vi "Process.vi"(8 "error in":errorcluster, 11 "Lockin.UI":refnum<class "Instrument UI.Lockin.lvclass">) -> (0 "error out":errorcluster, 3 "Lockin.UI out":refnum<class "Instrument UI.Lockin.lvclass">)   [LabVIEW 2019, in "Instrument.Lockin.lvlib" / "Instrument UI.Lockin.lvclass"]
doc: "---------------------------------------------------------------\nJKI State Machine Objects™\nhttp://jki.net/state-machine-objects/\nCopyright (C) 2005-2015, JKI <info@jki.net>\nALL RIGHTS RESERVEDJKI State Machine Objects (SMO) 1.0.0.5\nJKI - JKI\nCopyright (c) 2016, JKI"
uses:
  Instrument UI.Lockin.lvclass
  Instrument.DAQ/Typedefs/DAQ.Calibration--Cluster--Array.ctl
  Instrument.DAQ/Typedefs/DAQ.Calibration--Cluster.ctl
  Instrument.Lockin/Typedefs/Results Type--Enum.ctl
  Instrument.DAQ/Typedefs/Channel.Gain--Cluster--Array.ctl
  Instrument.DAQ/Typedefs/Channel.Gain--Cluster.ctl
  Instrument.DAQ/Typedefs/Sweep.Channel--Cluster--Array.ctl
  Instrument.DAQ/Typedefs/Sweep.Channel--Cluster.ctl
  Instrument.DAQ/Typedefs/Sweep.Pattern--Enum.ctl
  Instrument.DAQ/Typedefs/DAQ.Configuration--Cluster--Array.ctl
  Instrument.DAQ/Typedefs/DAQ.Configuration--Cluster.ctl
  Instrument.DAQ/Typedefs/DAQ.Config.AO.Range--enum.ctl
  Instrument.DAQ/Typedefs/DAQ.Config.AI.Range--enum.ctl
  Instrument.DAQ/Typedefs/DAQ.Config.AI.Coupling--enum.ctl
  Instrument.DAQ/Typedefs/DAQ.Sampling.Fs Mode--enum.ctl
  Instrument.DAQ/Typedefs/Simulation Mode--enum.ctl
  Instrument.DAQ/Typedefs/AI.Channel--Cluster--Array.ctl
  Instrument.DAQ/Typedefs/AI.Channel--Cluster.ctl
  Instrument.DAQ/Typedefs/AO.Channel--Cluster--Array.ctl
  Instrument.DAQ/Typedefs/AO.Channel--Cluster.ctl
  Instrument.DAQ/Typedefs/AO.Channel.Function--Enum.ctl
  Instrument.DAQ/Typedefs/REF.Channel--Cluster--Array.ctl
  Instrument.DAQ/Typedefs/REF.Channel--Cluster.ctl
  Typedefs/Display-Enum.ctl
  C:/Program Files/National Instruments/LabVIEW 2019/vi.lib/JKI/JKI SMO/SMO/SMO.lvclass
  C:/Program Files/National Instruments/LabVIEW 2019/user.lib/LevyLab/Instrument Framework/Instrument UI/Instrument UI.lvclass
  C:/Program Files/National Instruments/LabVIEW 2019/vi.lib/JKI/JKI SMO/SMO.UI/SMO.UI.lvclass
  Instrument.DAQ/Typedefs/Get State-enum.ctl
  Instrument.Lockin/Typedefs/API/Lockin.Commands--Enum.ctl
  Instrument.Lockin/Typedefs/API/Lockin.Commands.Local--Enum.ctl
  Instrument.DAQ/Typedefs/Set State-enum.ctl
  Instrument.DAQ/Typedefs/DAQ.Sampling.Sample Mode--Ring.ctl
  Instrument.Lockin/Typedefs/API/Lockin.setSweep_Table--cluster.ctl
  Instrument.Lockin/Typedefs/Offset Mode--Enum.ctl
  Instrument.DAQ/Typedefs/PrivateEvents--DAQ.setCalibration.ctl
  Typedefs/UI.References--Cluster.ctl
  Typedefs/UI.References.Booleans--Cluster.ctl
  Typedefs/UI.References.Clusters--Cluster.ctl
  Typedefs/UI.References.Graphs--Cluster.ctl
  <userlib>/LevyLab/Configuration/Configuration.lvclass
  Instrument.Lockin/Typedefs/Lockin.getAllData--Cluster.ctl
  Instrument.DAQ/Typedefs/PublicEvents--DAQ.getWaveforms.ctl
  Instrument.DAQ/Typedefs/Results--Cluster.ctl
  Instrument.DAQ/Typedefs/PublicEvents--DAQ.getSweepWaveforms.ctl
  Typedefs/UI.Configuration--Cluster.ctl
  Instrument.DAQ/Typedefs/Configuration.Channels--Cluster.ctl
  Instrument.DAQ/Typedefs/DAQ.Sampling--Cluster.ctl
  Instrument.DAQ/Typedefs/DAQ.Sampling.Sampling--Cluster.ctl
  Instrument.DAQ/Typedefs/Configuration.Prefilter--Cluster.ctl
  Instrument.DAQ/Typedefs/Channel.GainsAndOffsets--Cluster.ctl
  Instrument.DAQ/Typedefs/Configuration.AmplitudeLimit--Cluster.ctl
  Instrument.DAQ/Typedefs/Configuration.DCLimit--Cluster.ctl
  Instrument.DAQ/Typedefs/Configuration.LinkFrequencies--Cluster.ctl
  Instrument.DAQ/Typedefs/Sweep.Configuration--Cluster.ctl
  Instrument.Lockin/Instrument.Lockin.lvclass
  C:/Program Files/National Instruments/LabVIEW 2019/user.lib/LevyLab/Instrument Framework/Instrument/Instrument.lvclass
  <userlib>/LevyLab/Instrument Framework/Instrument UI/Instrument UI.lvclass/Instrument UI.ctl
  <userlib>/LevyLab/Configuration/Configuration.lvclass/Configuration.ctl
  <vilib>/JKI/JKI SMO/SMO/SMO.lvclass/SMO.ctl
  <vilib>/JKI/JKI SMO/SMO.UI/SMO.UI.lvclass/SMO.UI.ctl
  Instrument.Lockin/Typedefs/API/Lockin.setState--cluster.ctl
  Instrument.DAQ/Typedefs/PrivateEvents--DAQ.showUI.ctl
  Instrument.Lockin/Typedefs/API/Lockin.setLogMode--cluster.ctl
  Instrument.Lockin/Typedefs/API/Lockin.setSamplingMode--cluster.ctl
  Instrument.Lockin/Typedefs/API/Lockin.setSamplingFsMode--cluster.ctl
  3787d8ba-7746-42f4-a076-e634e239a42a.vi
  <vilib>/JKI/JKI SMO/SMO/Private/ReftoDVR--SMO.vi
  <vilib>/JKI/JKI SMO/SMO.UI/SMO.UI.ReftoDVR.vi
  3787d8ba-7746-42f4-a076-e634e239a42a.vi/a8b20e46-8953-45b0-93f7-28fc699f087e.vi
  3787d8ba-7746-42f4-a076-e634e239a42a.vi/bdb78403-1b99-4c02-9c62-cc137de50f7f.vi
  <vilib>/Platform/browser.llb/Open URL in Default Browser (string).vi
  <vilib>/Waveform/WDTOps.llb/WDT Waveform Duration DBL.vi
  private/Set All Plot Visibility (WFChart).vi
  private/Get Plot Visibility (WFChart).vi
  private/Set Plot Visibility (WFChart).vi
  private/Set Plot Visibility (WDTWFGraph).vi
  private/Set Legend (WDTWFGraph).vi
  private/Set Plot Color (WFChart).vi
  <vilib>/Utility/Data Type/Get Type Information.vi
  <vilib>/Utility/Data Type/Get Numeric Information.vi
  <userlib>/_OpenG.lib/lvdata/lvdata.llb/Unwrap VVariant__ogtk.vi
  <vilib>/JDP Science/JSONtext/Variant to JSON Text.vi
  <userlib>/LevyLab/Instrument Framework/Instrument/API/Instrument.sendMessageToProcess (string).vi
  <userlib>/LevyLab/Instrument Framework/Instrument/Instrument.lvclass
  <vilib>/JDP Science/JSONtext/LVClass Serializer/JSONtext LVClass Serializer.lvclass
  <userlib>/LevyLab/Instrument Framework/Instrument UI/Instrument UI.lvclass
  Instrument.DAQ/Instrument.DAQ.lvclass
  <vilib>/measure/NI_MAPro.lvlib
  <vilib>/JKI/JKI SMO/SMO/SMO.lvclass
  <vilib>/JKI/JKI SMO/SMO.UI/SMO.UI.lvclass
  Lockin.Utilities/Lockin.Utilities.lvlib
  private/Set All Plot Visibility (WFGraph).vi
  private/Set All Plot Visibility (XYGraph).vi
  private/Get Plot Visibility (WFGraph).vi
  private/Set Plot Visibility (WFGraph).vi
  private/Set Plot Visibility (XYGraph).vi
  private/Set Legend (WFGraph).vi
  private/Set Plot Color (WFGraph).vi
  private/Set Plot Color (WDTWFGraph).vi
  private/Set Legend (WFChart).vi
  private/Set Legend (XYGraph).vi
  private/Set Plot Color (XYGraph).vi
  <vilib>/measure/maspectr.llb/FFT Power Spectrum and PSD for N Chan.vi
panel:
  in  "Decimation (post DSP)":i32=1
  in  "....................State....................":bool
  in  "....................Graph and UI....................":bool
  in  "....................DAQ and Channel....................":bool
  in  "....................Dynamic Events....................":bool
  out "Version":string="vDevelopment" caption="V"
  in  "Left Tab":T1(tab)=enum."Sweep"
  in  "AO DC Limit":dbl=0.009999999 format="%.3p"
  in  "Limit DC (V)":bool
  in  "Disable all AI Ref":bool
  in  "Enable only AI Ref1":bool
  in  "Reset Phase":bool
  in  "AI Channels":T2 {"References" items=["", "1", "2", "3"]; "Channel" min=1}
  in  "AO freq link":dbl=13.0 format="%.3p"
  in  "AO Amp Limit":dbl=0.009999999 format="%.3p"
  in  "Limit Amplitude (V)":bool
  in  "Link Frequencies":bool
  in  "LP f (Hz)":dbl=100.0 format="%.3p"
  in  "Line":bool
  in  "Lowpass":bool
  in  "AO Channels":T4 {"Phase" format="%.3g"; "Frequency" min=0.0001 max=10000.0 format="%.3g"; "Offset" format="%.3p"; "Amplitude" min=0.0 max=10.0 format="%.3p"}
  in  "REF Channels":T7 {"Roll-Off" min=1; "TC" min=0.0001 format="%#_3p"; "Phase" format="%.3g"; "Frequency" min=0.0001 max=10000.0 format="%.3g"; "Channel" min=1}
  in  "Input Gain":T9
  in  "Output Gain":T9
  in  "Input Offsets":T9 {"Gain" format="%#_3p"}
  in  "Show UI":bool
  in  "Fs Output (S/s)":dbl=10.0 format="%#_13g"
  in  "Fs (S/s)":dbl=10.0 format="%#_13g"
  in  "#s (S)":i32=10
  in  "DAQ Config":T11 {"AI.Coupling" items=["AC"=10045, "DC"=10050, "GND"=10066]}
  in  "Auto DAQ":bool caption="Auto"
  in  "Refresh Rate (Hz)":dbl=10.0 format="%#_13g"
  in  "Fs Mode":T16
  in  "Fs Multiplier":dbl=5000.0 format="%#_13g"
  in  "Decimation (pre DSP)":i32=1
  in  "Remove Offset":bool caption="Remove"
  in  "Measure Offset":bool caption="Measure"
  in  "Logging":bool
  in  "AI Simulation mode":T17=enum."AI = noise*AO"
  in  "Sweep Pattern":cluster{"Channel":u16, "Sweep Pattern":dbl[]}[](array[cluster])=[{"Channel"=0, "Sweep Pattern"=[]}] {"Sweep Pattern" format="%#_3p"; "Channel" min=1 max=128}
  in  "Sweep Channels":T18=[{"Enable?"=FALSE, "Channel"=0, "Start"=0.0, "End"=0.1, "Pattern"=enum."Table", "Table"=[]}] {"Table" format="%#_1f"; "Channel" min=1 max=128; "Start" format="%#_6p"; "End" format="%#_6p"}
  in  "Sweep Time (s)":dbl=20.0
  in  "Initial Wait (s)":dbl=1.0
  out "Sweep Timer (s)":dbl caption="Timer (s)"
  in  "Return to Start?":bool
  out "Sampling Status":string="Good"
  out "State History":string
  out "WFM Refresh time (ms)":u32=103
  out "Instrument.DAQ SMO State":string caption="SMO State"
  out "UI Refresh time (ms)":u32=103
  in  "Update":bool
  in  "Enable Output":bool caption="Enable"
  in  "Output Channel":i32=1 min=1
  out "Output (V)":dbl
  in  "Aux Channel":tag="Dev2/ao0"
  in  "Voltage Output (V)":dbl min=-50.0 max=50.0
  in  "Amplifier Gain":dbl=1.0 min=-15.0 max=15.0
  out "DAQ Output (V)":dbl=-0.0 min=-3.5 max=3.5
  out "Amplified Output (V)":dbl=-0.0 min=-3.5 max=3.5
  in  "AI Channel":i32=1
  in  "Reference Channel":i32=1
  in  "Type":T21
  out "state":T22=enum."created"
  out "current time":dbl format="%<%I:%M:%S %p %m/%d/%Y>T"
  out "getAll.DAQ state":T22=enum."created"
  out "current time 2":dbl format="%<%I:%M:%S %p %m/%d/%Y>T"
  in  "Get Calibration":bool
  out "Cal Info":T23 {"DevTemp" format="%.1f"; "SelfCal.LastTemp" format="%.1f"; "SelfCal.LastDate/Time" format="%<%I:%M %p %m/%d/%Y>T"}
  in  "Self Calibrate":bool
  in  "Tab Control 3":enum32{"Page 1"}(tab)
  out "X":dbl caption="X (V)" format="%#_3p"
  out "Y":dbl caption="Y (V)" format="%#_3p"
  in  "Channel":i32(ring)=1 items=["AI1 Ref1", "AI2 Ref1", "AI3 Ref1", "AI4 Ref1", "AI5 Ref1", "AI6 Ref1", "AI7 Ref1", "AI8 Ref1"]
  out "R":dbl caption="R (V)" format="%#_3p"
  out "Theta":dbl caption="Theta (°)" format="%#_3p"
  in  "Display":T25=enum."R and Theta" caption="Enum"
  in  "Close":bool
  out "Status":string="Shutdown"
  in  "Pause":bool
  in  "Reset":bool
  in  "Start":bool
  in  "Help":bool
  in  "Start Sweep":bool
  in  "Stop Sweep":bool
  in  "Right Tab":T26(tab)
  in  "AI Graph All":bool
  in  "AI Graph None":bool
  in  "Y Axis (Output)":enum16{"Analog Output", "Reference"}(ring) caption="Enum 3"
  in  "Y Axis (Input)":enum16{"Device", "ADC"}(ring) caption="Enum 3"
  in  "Decimate (UI)":enum16{"1", "10", "100", "1000"}(ring) caption="Enum 3"
  in  "X Axis":enum16{"Time", "Samples"}(ring) caption="Enum 3"
  out "AI Graph":waveform(dbl)[](graph)
  out "AO Graph":waveform(dbl)[](graph)
  in  "AO Graph All":bool
  in  "AO Graph None":bool
  in  "Y/Theta Range":dbl caption="Axis Range" format="%#_6p"
  in  "X/R Range":dbl caption="Axis Range" format="%#_6p"
  out "Lockin 2":waveform(dbl)[](graph) caption="Lockin Display 2"
  out "Lockin 1":waveform(dbl)[](graph)
  in  "Lockin Graph None":bool
  in  "Lockin Graph All":bool
  out "Results":string[][](table)
  out "XY Graph":cluster{"Wavenumber":dbl[], "Data":dbl[]}[](graph)
  in  "XY Range":dbl caption="Axis Range" format="%#_6p"
  out "Sweep AI":waveform(dbl)[](graph)
  out "Sweep AO":waveform(dbl)[](graph)
  out "Sweep Results Y":waveform(dbl)[](graph)
  out "Sweep Results X":waveform(dbl)[](graph)
  in  "# averages":u32=10 min=1
  in  "weighting mode":enum16{"Linear", "Exponential"}(ring)=enum."Exponential"
  in  "averaging mode":T27(ring)=enum."RMS averaging"
  in  "window":u16(ring) items=["Rectangle", "Hanning"]
  in  "export mode":u16(ring)=1 items=["Power Spectrum", "Power Spectral Density"]
  in  "restart":bool
  out "done?":bool=TRUE
  out "PS Chart":dbl[][](graph)
  out "PS WFGraph":cluster{"f0":dbl, "df":dbl, "magnitude":dbl[]}[](graph)
  out "averages":dbl=180.0
  # "Lockin UI"
  # "For instructions on how to use the JKI State Machine Objects, examples and video tutorials, visit:\nhttp://jki.net/state-machine-objects/\n\nJKI State Machine Objects™\nhttp://jki.net/state-machine-objects/\nCopyright (C) 2005-2015, JKI <info@jki.net>\nALL RIGHTS RESERVED"
  # "Output"
  # "Input"
  # ">> DEVICE >>"
  # "(*)"
  # "Ch"
  # "Amp (V)"
  # "DC (V)"
  # "f (Hz)"
  # "Phase (°)"
  # "Function"
  # "Sweep"
  # "(*)"
  # "Ch"
  # "Ref1   2     3    4"
  # "Input: Pre-Filter"
  # "Output Settings"
  # "Reference"
  # "Reference Settings"
  # "Ch"
  # "f (Hz)"
  # "Phase (°)"
  # "TC (s)"
  # "Order (n/2)"
  # "Ch"
  # "Input Gain"
  # "Ch"
  # "Output Gain"
  # "Ch"
  # "Offset"
  # "DAQ Channels"
  # "AI"
  # "Device"
  # "AO"
  # "DAQ"
  # "Ch"
  # "Range"
  # "Ch"
  # "Range"
  # "Coupling"
  # "Logging"
  # "Sampling"
  # "Input: Offset"
  # "Sweep"
  # "Pattern"
  # "(*)"
  # "Ch"
  # "Start"
  # "End"
  # "Ch"
  # "Table"
  # "Status"
  # "Auxiliary Output"
  # "Configuration"
  # "- Use to control an auxiliiary card such as a multifunction DAQ (6115, 6120, etc)"
  # "Forward Lockin Input --> Lockin Output"
  # "- Choose an input lockin channel and value (X,Y, etc) and it will be written as a DC value to an output channel of your choosing.\n- Output is scaled by the input amplifier gain."
  # "Calibration"
  # "Self Cal\nLast Time"
  # "Self Cal\nLast Temp"
  # "Temp\nNow"
  # "Cal\nDue"
  # "Device"
  # "DAQ"
  # "Sweep"
  # "Application"
  # "Status"
  # "AI Graph"
  # "AO/Reference Graph"
  # "Lockin Results 1"
  # "Lockin Results 2"
  # "Lockin Results 3"
  # "Sweep AO/AI"
  # "Sweep Results"
  # "Power Spectra"
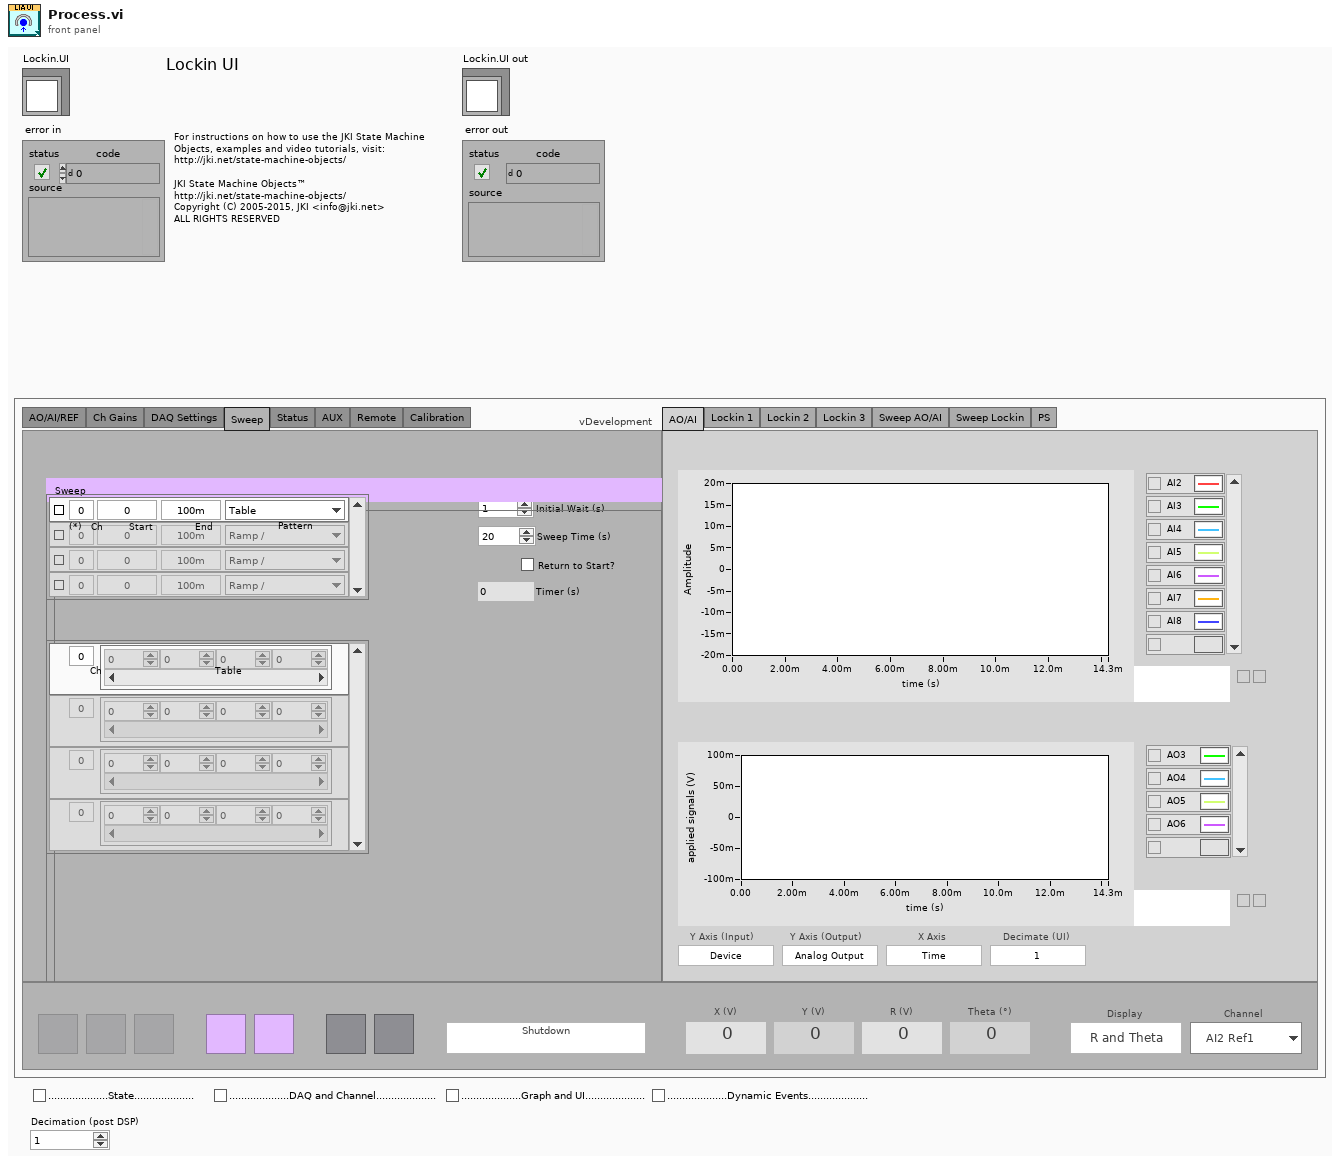
[diagram p1: front panel]
types:
  T1 = enum32{"AO/AI/REF", "Ch Gains", "DAQ Settings", "Sweep", "Status", "AUX", "Remote", "Calibration"}
  T2 = typedef "Instrument.Lockin.lvlib/Instrument.DAQ.lvclass/AI.Channel--Cluster--Array.ctl" = T3[]
  T3 = typedef "Instrument.Lockin.lvlib/Instrument.DAQ.lvclass/AI.Channel--Cluster.ctl" = cluster{"Enable?":bool, "Channel":i32, "References":i32[]}
  T4 = typedef "Instrument.Lockin.lvlib/Instrument.DAQ.lvclass/AO.Channel--Cluster--Array.ctl" = T5[]
  T5 = typedef "Instrument.Lockin.lvlib/Instrument.DAQ.lvclass/AO.Channel--Cluster.ctl" = cluster{"Enable?":bool, "Channel":i32, "Amplitude":dbl, "Offset":dbl, "Frequency":dbl, "Phase":dbl, "Function":T6, "Sweeping?":bool}
  T6 = typedef "Instrument.Lockin.lvlib/Instrument.DAQ.lvclass/AO.Channel.Function--Enum.ctl" = enum16{"Sine", "Triangle", "Square"}
  T7 = typedef "Instrument.Lockin.lvlib/Instrument.DAQ.lvclass/REF.Channel--Cluster--Array.ctl" = T8[]
  T8 = typedef "Instrument.Lockin.lvlib/Instrument.DAQ.lvclass/REF.Channel--Cluster.ctl" = cluster{"Enable?":bool, "Channel":i32, "Frequency":dbl, "Phase":dbl, "TC":dbl, "Roll-Off":i32}
  T9 = typedef "Instrument.Lockin.lvlib/Instrument.DAQ.lvclass/Channel.Gain--Cluster--Array.ctl" = T10[]
  T10 = typedef "Instrument.Lockin.lvlib/Instrument.DAQ.lvclass/Channel.Gain--Cluster.ctl" = cluster{"Channel":string, "Gain":dbl}
  T11 = typedef "Instrument.Lockin.lvlib/Instrument.DAQ.lvclass/DAQ.Configuration--Cluster--Array.ctl" = T12[]
  T12 = typedef "Instrument.Lockin.lvlib/Instrument.DAQ.lvclass/DAQ.Configuration--Cluster.ctl" = cluster{"Device":string, "AO.Ch":string, "AO.Range":T13, "AI.Ch":string, "AI.Range":T14, "AI.Coupling":T15}
  T13 = typedef "Instrument.Lockin.lvlib/Instrument.DAQ.lvclass/DAQ.Config.AO.Range--enum.ctl" = enum16{"±0.1", "±1.0", "±10.0"}
  T14 = typedef "Instrument.Lockin.lvlib/Instrument.DAQ.lvclass/DAQ.Config.AI.Range--enum.ctl" = enum16{"±0.316", "±1.00", "±3.16", "±10.0", "±31.6", "±42.4"}
  T15 = typedef "Instrument.Lockin.lvlib/Instrument.DAQ.lvclass/DAQ.Config.AI.Coupling--enum.ctl" = u16
  T16 = typedef "Instrument.Lockin.lvlib/Instrument.DAQ.lvclass/DAQ.Sampling.Fs Mode--enum.ctl" = enum16{"Manual", "Auto Fs", "Max Fs"}
  T17 = typedef "Instrument.Lockin.lvlib/Instrument.DAQ.lvclass/Simulation Mode--enum.ctl" = enum16{"AI = HW simulated", "AI = noise*AO", "AI = waveguide"}
  T18 = typedef "Instrument.Lockin.lvlib/Instrument.DAQ.lvclass/Sweep.Channel--Cluster--Array.ctl" = T19[]
  T19 = typedef "Instrument.Lockin.lvlib/Instrument.DAQ.lvclass/Sweep.Channel--Cluster.ctl" = cluster{"Enable?":bool, "Channel":u16, "Start":dbl, "End":dbl, "Pattern":T20, "Table":dbl[]}
  T20 = typedef "Instrument.Lockin.lvlib/Instrument.DAQ.lvclass/Sweep.Pattern--Enum.ctl" = enum16{"Ramp /", "Ramp /\\", "Smooth Ramp _/", "Smooth Ramp _/\\_", "Table"}
  T21 = typedef "Instrument.Lockin.lvlib/Instrument.Lockin.lvclass/Results Type--Enum.ctl" = enum16{"X", "Y", "R", "Theta", "Mean"}
  T22 = typedef "Instrument.Lockin.lvlib/Instrument.DAQ.lvclass/Get State-enum.ctl" = enum16{"idle", "created", "started", "stopped", "sweeping"}
  T23 = typedef "Instrument.Lockin.lvlib/Instrument.DAQ.lvclass/DAQ.Calibration--Cluster--Array.ctl" = T24[]
  T24 = typedef "Instrument.Lockin.lvlib/Instrument.DAQ.lvclass/DAQ.Calibration--Cluster.ctl" = cluster{"Active Device":string, "SelfCal.LastDate/Time":dbl, "SelfCal.LastTemp":dbl, "DevTemp":dbl, "calibration due?":bool}
  T25 = typedef "Instrument.Lockin.lvlib/Instrument UI.Lockin.lvclass/Display-Enum.ctl" = enum16{"X and Y", "R and Theta", "Mean"}
  T26 = enum32{"AO/AI", "Lockin 1", "Lockin 2", "Lockin 3", "Sweep AO/AI", "Sweep Lockin", "PS"}
  T27 = enum16{"No averaging", "Vector averaging", "RMS averaging", "Peak hold"}
  T28 = typedef "Instrument.Lockin.lvlib/Instrument.Lockin.lvclass/Lockin.Commands.Local--Enum.ctl" = enum16{"autoConfigureDAQ", "setSimulationMode", "zeroPhase", "setCalibration", "setPreFilter", "setLinkFrequencies", "setLimitAmplitude", "setLimitDC", "setSamplingDecimationPreDSP", "setSamplingDecimationPostDSP", "setSamplingMode", "setSamplingFsMultiplier", "setSamplingFsOutput", "setSamplingRefreshRate", "setData_State", "setData_DAQ", "setData_Sampling", "setData_Waveforms", "setData_Results", "setData_SweepWaveforms", "setData_AIChannels", "setData_AOChannels", "setData_REFChannels", "setData_InputGain", "setData_OutputGain", "showUI", "setAI", "setOffset", "setOffsetMode"}
  T29 = typedef "Instrument.Lockin.lvlib/Instrument.Lockin.lvclass/Lockin.Commands--Enum.ctl" = enum16{"setAO", "setAO_Amplitude", "setAO_DC", "setAO_Frequency", "setAO_Phase", "setAO_Function", "setREF", "setREF_Frequency", "setREF_Phase", "setREF_TC", "setREF_Roll-Off", "setDAQ", "setSampling", "setState", "getState", "getAO", "getAI", "getResults", "getSampling", "getAOconfig", "getREFconfig", "setInputGain", "setOutputGain", "getInputGain", "getOutputGain", "setSamplingFsMode", "getSamplingFsMode", "setSweep", "setSweep_Time", "setSweep_Table", "getStatus", "getSweepResults", "getSweepWaveforms", "startLogging", "stopLogging"}
  T30 = enum16{"Spinner 1", "Spinner 2", "Spinner 3", "Spinner 4", "Spinner 5", "Spinner 6"}
  T31 = typedef "Instrument.Lockin.lvlib/Instrument.DAQ.lvclass/Set State-enum.ctl" = enum16{"start", "stop", "reset", "start sweep", "stop sweep"}
  T32 = typedef "Instrument.Lockin.lvlib/Instrument.Lockin.lvclass/Lockin.setSweep_Table--cluster.ctl" = cluster{"Channel":i32, "Table":dbl[]}
  T33 = typedef "Instrument.Lockin.lvlib/Instrument.Lockin.lvclass/Offset Mode--Enum.ctl" = enum16{"Measure", "Remove"}
  T34 = typedef "Instrument.Lockin.lvlib/Instrument.DAQ.lvclass/PrivateEvents--DAQ.setCalibration.ctl" = enum16{"Check", "Calibrate"}
  T35 = enum32{"invalid app kind", "Development System", "Run Time System", "Student Edition", "Embedded LabVIEW", "Evaluation", "Custom"}
  T36 = enum8{"Enabled", "Disabled", "Disabled and Grayed Out"}
  T37 = enum32{"Invalid", "Standard", "Closed", "Hidden", "Minimized", "Maximized"}
  T38 = typedef "Instrument.Lockin.lvlib/Instrument.Lockin.lvclass/Lockin.setState--cluster.ctl" = cluster{"State":T31}
  T39 = typedef "Instrument.Lockin.lvlib/Instrument.DAQ.lvclass/PrivateEvents--DAQ.showUI.ctl" = bool
  T40 = typedef "Instrument.Lockin.lvlib/Instrument.Lockin.lvclass/Lockin.setLogMode--cluster.ctl" = cluster{"interval":u32}
  T41 = typedef "Instrument.Lockin.lvlib/Instrument.Lockin.lvclass/Lockin.setSamplingMode--cluster.ctl" = cluster{"SampleMode":T42}
  T42 = typedef "Instrument.Lockin.lvlib/Instrument.DAQ.lvclass/DAQ.Sampling.Sample Mode--Ring.ctl" = i32
  T43 = typedef "Instrument.Lockin.lvlib/Instrument.Lockin.lvclass/Lockin.setSamplingFsMode--cluster.ctl" = cluster{"FsMode":T16}
  T44 = cluster{"averaging mode":enum16{"No averaging", "Vector averaging", "RMS averaging", "Peak hold"}, "weighting mode":enum16{"Linear", "Exponential"}, "number of averages":u32}
  T45 = typedef "Instrument.Lockin.lvlib/Instrument UI.Lockin.lvclass/UI.Configuration--Cluster.ctl" = cluster{"Channels":T46, "DAQ":cluster{"Configuration":T11, "cfg.Sampling":T47, "Calibration":T23, "Simulation mode":T17}, "PreFilter":T49, "Amplifers":T50, "Limit Amplitude":T51, "Limit DC":T52, "Link Frequencies":T53, "Aux Channel":tag, "Sweep":T54, "Plot":cluster{"visibility.AI":bool[], "visibility.AO":bool[], "visibility.Lockin":bool[]}}
  T46 = typedef "Instrument.Lockin.lvlib/Instrument.DAQ.lvclass/Configuration.Channels--Cluster.ctl" = cluster{"Cfg_AO":T4, "Cfg_AI":T2, "Cfg_REF":T7}
  T47 = typedef "Instrument.Lockin.lvlib/Instrument.DAQ.lvclass/DAQ.Sampling--Cluster.ctl" = cluster{"Sampling":T48, "sample mode":i32, "Fs Mode":T16, "Fs Multiplier":dbl, "Refresh Rate (Hz)":dbl, "Decimation.PreDSP":i32, "Decimation.PostDSP":i32, "Fs.Output":dbl}
  T48 = typedef "Instrument.Lockin.lvlib/Instrument.DAQ.lvclass/DAQ.Sampling.Sampling--Cluster.ctl" = cluster{"Fs":dbl, "#s":i32}
  T49 = typedef "Instrument.Lockin.lvlib/Instrument.DAQ.lvclass/Configuration.Prefilter--Cluster.ctl" = cluster{"60 Hz":bool, "Low Pass":bool, "Low Pass Cutoff (Hz)":dbl}
  T50 = typedef "Instrument.Lockin.lvlib/Instrument.DAQ.lvclass/Channel.GainsAndOffsets--Cluster.ctl" = cluster{"Offset_AI":T9, "Gain_AI":T9, "Gain_AO":T9}
  T51 = typedef "Instrument.Lockin.lvlib/Instrument.DAQ.lvclass/Configuration.AmplitudeLimit--Cluster.ctl" = cluster{"Limit?":bool, "Limit (V)":dbl}
  T52 = typedef "Instrument.Lockin.lvlib/Instrument.DAQ.lvclass/Configuration.DCLimit--Cluster.ctl" = cluster{"Limit?":bool, "Limit (V)":dbl}
  T53 = typedef "Instrument.Lockin.lvlib/Instrument.DAQ.lvclass/Configuration.LinkFrequencies--Cluster.ctl" = cluster{"Link?":bool, "Frequency (Hz)":dbl}
  T54 = typedef "Instrument.Lockin.lvlib/Instrument.DAQ.lvclass/Sweep.Configuration--Cluster.ctl" = cluster{"Sweep Time (s)":dbl, "Initial Wait (s)":dbl, "Return to Start":bool, "Channels":T18}
  T55 = typedef "Instrument.Lockin.lvlib/Instrument.Lockin.lvclass/Lockin.getAllData--Cluster.ctl" = cluster{"DAQ State":T22, "Waveforms":T56, "Results":T57, "SweepWaveforms":T58}
  T56 = typedef "Instrument.Lockin.lvlib/Instrument.DAQ.lvclass/PublicEvents--DAQ.getWaveforms.ctl" = cluster{"AO_wfm":waveform(dbl)[], "AI_wfm":waveform(dbl)[], "Ref_X_wfm":waveform(dbl)[], "Ref_Y_wfm":waveform(dbl)[], "X_wfm":waveform(dbl)[], "Y_wfm":waveform(dbl)[]}
  T57 = typedef "Instrument.Lockin.lvlib/Instrument.DAQ.lvclass/Results--Cluster.ctl" = cluster{"Time Stamp":timestamp, "Results (Dictionary)":cluster{"key":string, "value":dbl}[]}
  T58 = typedef "Instrument.Lockin.lvlib/Instrument.DAQ.lvclass/PublicEvents--DAQ.getSweepWaveforms.ctl" = cluster{"AO_wfm":waveform(dbl)[], "AI_wfm":waveform(dbl)[], "X_wfm":waveform(dbl)[], "Y_wfm":waveform(dbl)[]}
  T59 = typedef "Instrument.Lockin.lvlib/Instrument UI.Lockin.lvclass/UI.References--Cluster.ctl" = cluster{"Booleans":T60, "Clusters":T61, "Graphs":T62}
  T60 = typedef "Instrument.Lockin.lvlib/Instrument UI.Lockin.lvclass/UI.References.Booleans--Cluster.ctl" = cluster{"Start":refnum<vi>, "Pause":refnum<vi>, "Reset":refnum<vi>, "Trigger":refnum<vi>, "Help":refnum<vi>, "Close":refnum<vi>, "Start Sweep":refnum<vi>, "Stop Sweep":refnum<vi>}
  T61 = typedef "Instrument.Lockin.lvlib/Instrument UI.Lockin.lvclass/UI.References.Clusters--Cluster.ctl" = cluster{"AO Channels":refnum<vi>, "AI Channels":refnum<vi>, "REF Channels":refnum<vi>, "DAQ Config":refnum<vi>, "Sweep Channels":refnum<vi>, "Cal Info":refnum<vi>}
  T62 = typedef "Instrument.Lockin.lvlib/Instrument UI.Lockin.lvclass/UI.References.Graphs--Cluster.ctl" = cluster{"AI Graph":refnum<vi>, "AO Graph":refnum<vi>, "Lockin 1":refnum<vi>, "Lockin 2":refnum<vi>, "XY Graph":refnum<vi>, "Sweep X Graph":refnum<vi>, "Sweep Y Graph":refnum<vi>, "Sweep AI Graph":refnum<vi>, "Sweep AO Graph":refnum<vi>, "PS WFGraph":refnum<vi>, "PS Chart":refnum<vi>}
  T63 = cluster{"Core":cluster{"Current VI Reference":refnum<vi>, "Close Panel on Exit?":bool, "Last Error":cluster{"error":errorcluster, "previous state":string, "remaining states":string}, "Shutdown?":bool}, "SelfRef":refnum<class "Instrument UI.Lockin.lvclass">, "Lockin":refnum<class "Instrument.Lockin.lvclass">, "Configuration":refnum<class "Configuration.lvclass">, "UI Config":T45, "DAQ state":T22, "getAll":T55, "References":T59, "Message":cluster{"Command":variant, "Data":variant}, "Plot Names":string[], "Front Panel":refnum<vi>}
  T64 = typedef "SMO.lvclass/SMOState --Enum.ctl" = enum16{"unknown", "Created", "Started", "Stopped"}
  T65 = cluster{"Current VI Reference":refnum<vi>, "Close Panel on Exit?":bool, "Last Error":cluster{"error":errorcluster, "previous state":string, "remaining states":string}, "Shutdown?":bool}
  T66 = typedef "SMO.lvclass/Protected Events.ctl" = cluster{"StopProcesses":refnum<user-event>, "AbortProcesses":refnum<user-event>, "Config Changed":refnum<user-event>, "Dependency":refnum<user-event>}
  T67 = typedef "Instrument.lvlib/Instrument.lvclass/PublicEvents--Cluster.ctl" = cluster{"MessageFromProcess":refnum<user-event>}
  T68 = typedef "SMO.UI.lvclass/PublicEvents--Cluster.ctl" = cluster{"UI Hidden":refnum<user-event>, "UI State":refnum<user-event>}
  T69 = typedef "SMO.lvclass/Public Events.ctl" = cluster{"Error":refnum<user-event>, "State":refnum<user-event>, "Reserve State":refnum<user-event>}
  T70 = typedef "Instrument.Lockin.lvlib/Instrument.DAQ.lvclass/PublicEvents--Cluster.ctl" = cluster{"getAIChannels":refnum<user-event>, "getAOChannels":refnum<user-event>, "getREFChannels":refnum<user-event>, "getWaveforms":refnum<user-event>, "getResults":refnum<user-event>, "getSweepWaveforms":refnum<user-event>, "getCalibration":refnum<user-event>, "getDAQState":refnum<user-event>, "getDAQconfig":refnum<user-event>, "getInputGain":refnum<user-event>, "getOutputGain":refnum<user-event>, "getInputOffset":refnum<user-event>, "getSampling":refnum<user-event>, "getSweepChannels":refnum<user-event>, "getDeviceIDN":refnum<user-event>}
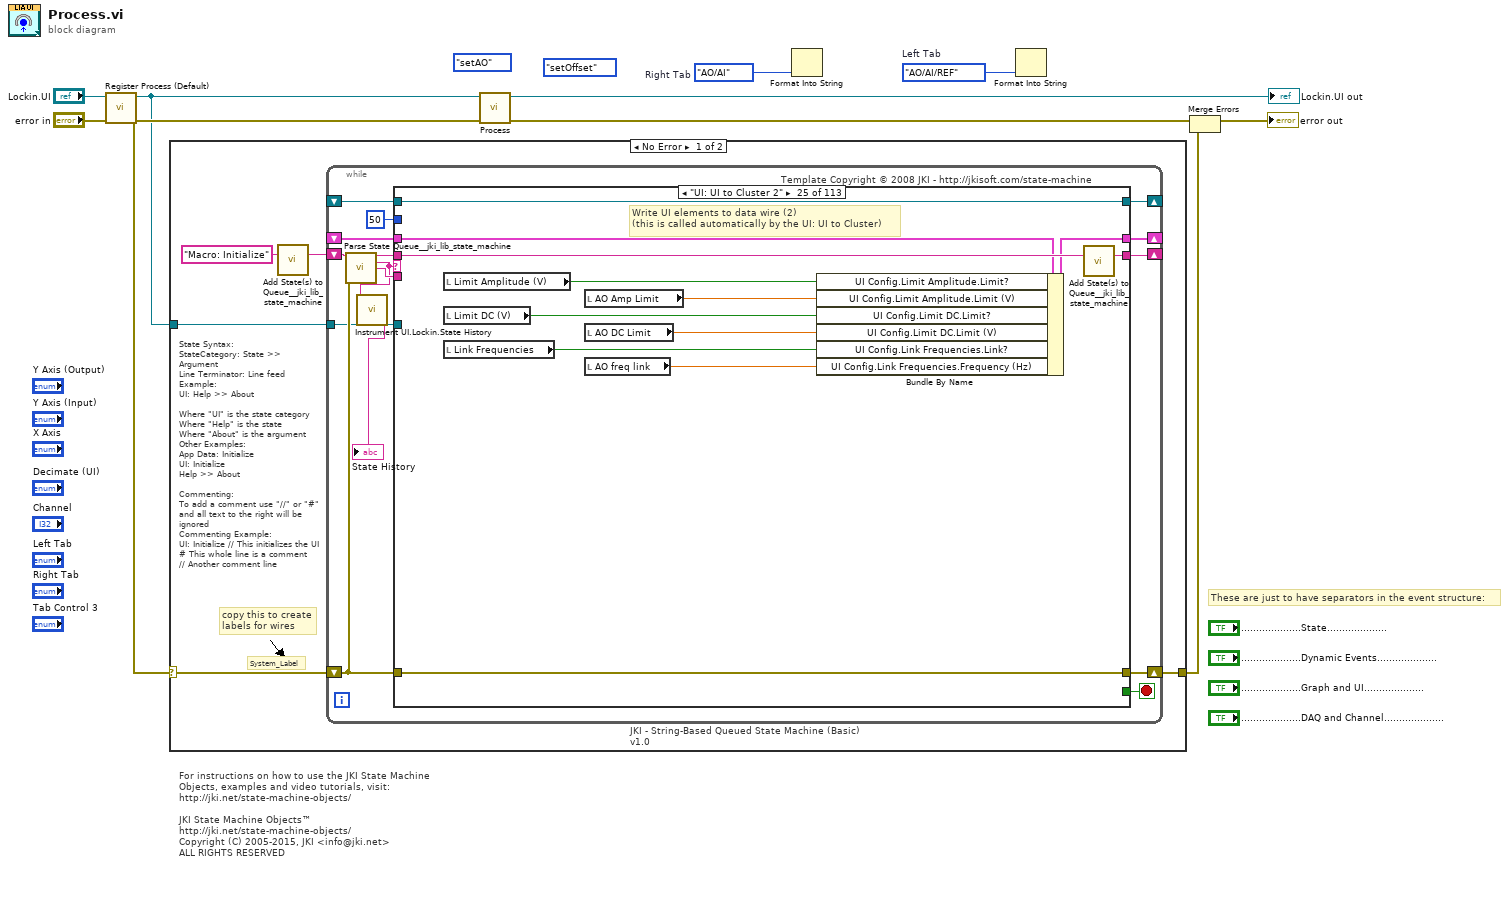
[diagram p0: block diagram]
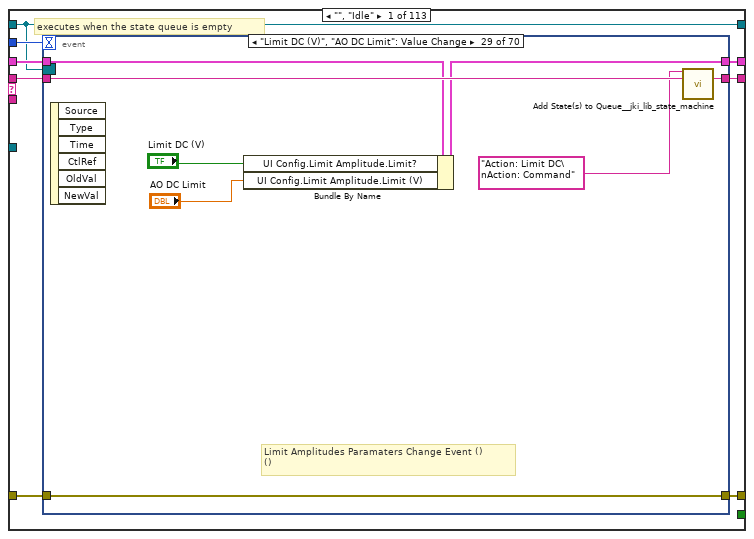
[diagram p2: hidden frame]
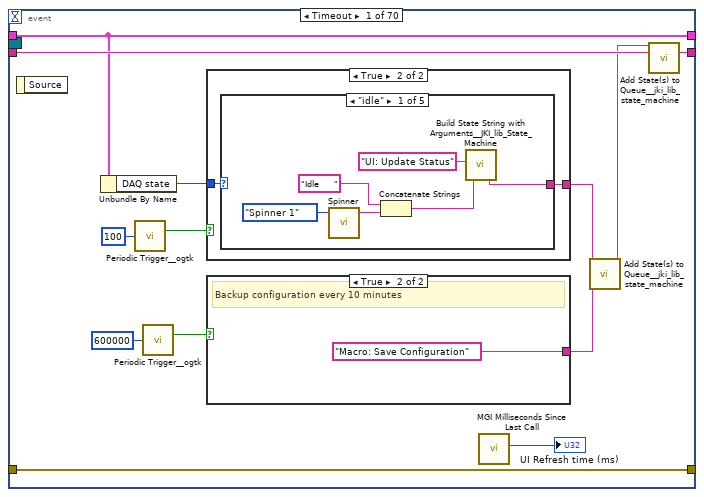
[diagram p3: hidden frame]
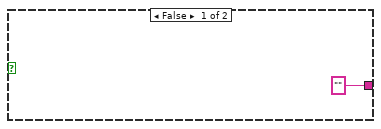
[diagram p4: hidden frame]
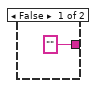
[diagram p5: hidden frame]
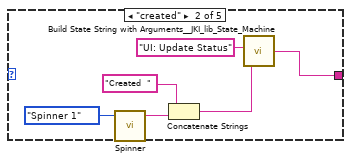
[diagram p6: hidden frame]
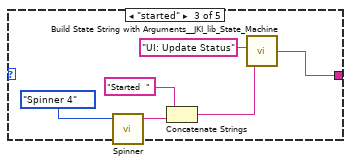
[diagram p7: hidden frame]
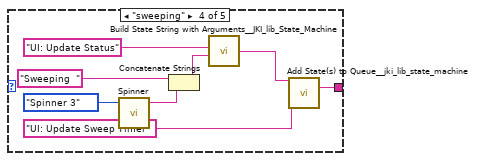
[diagram p8: hidden frame]
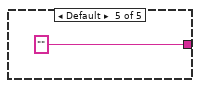
[diagram p9: hidden frame]
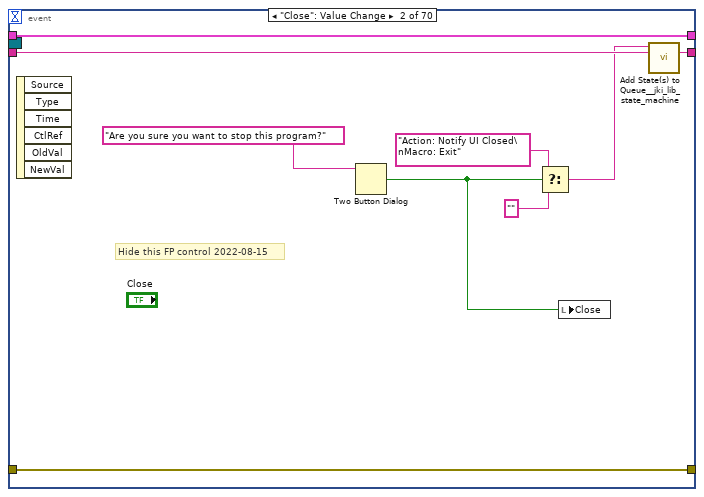
[diagram p10: hidden frame]
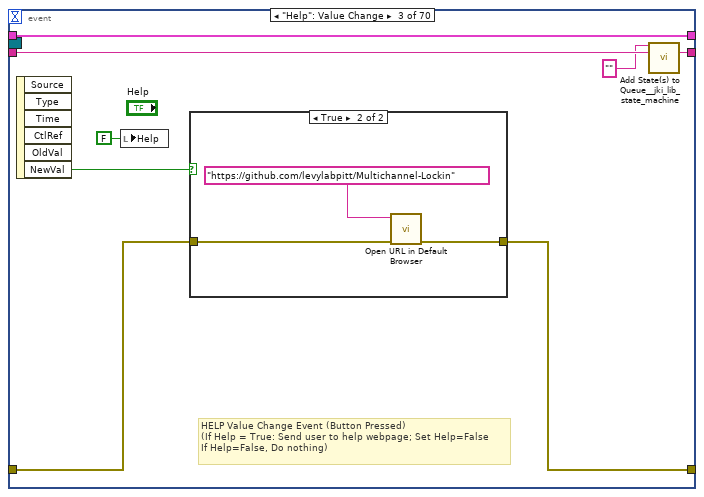
[diagram p11: hidden frame]
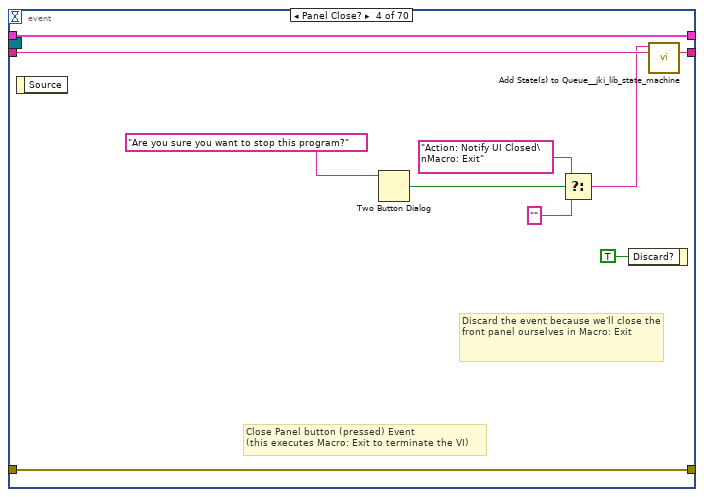
[diagram p13: hidden frame]
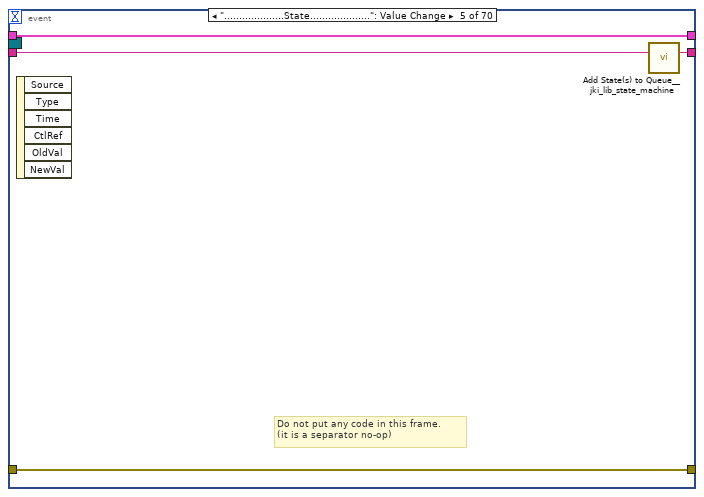
[diagram p14: hidden frame]
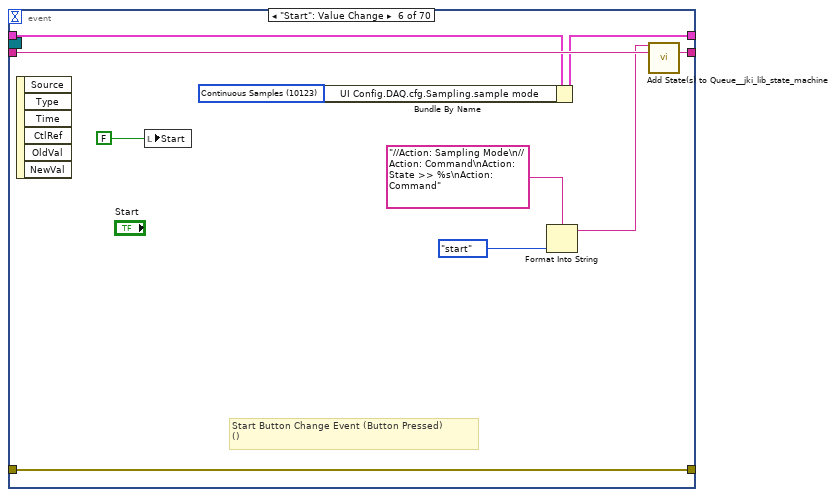
[diagram p15: hidden frame]
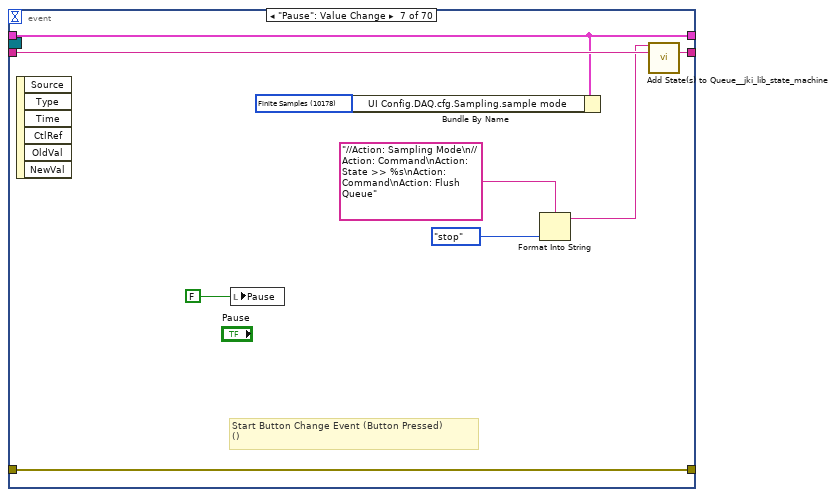
[diagram p16: hidden frame]
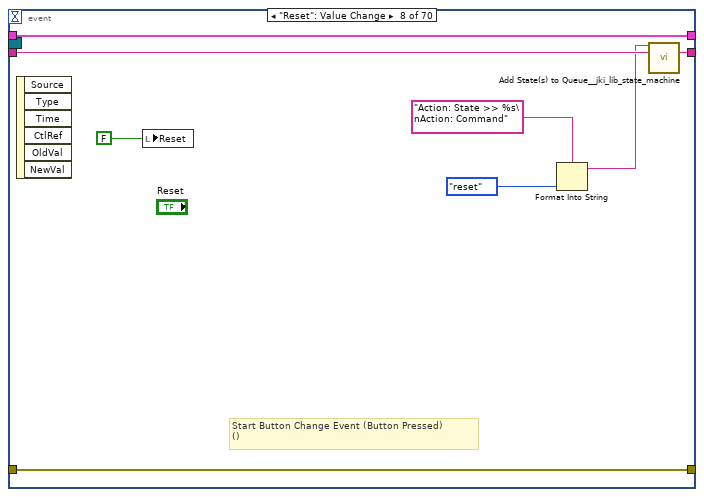
[diagram p17: hidden frame]
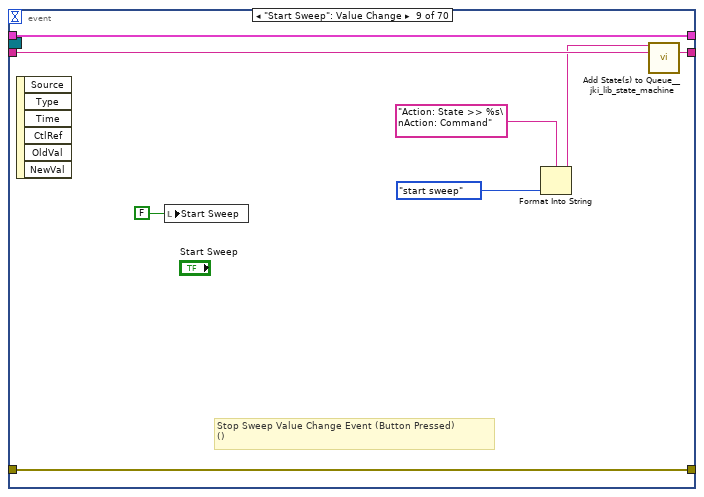
[diagram p18: hidden frame]
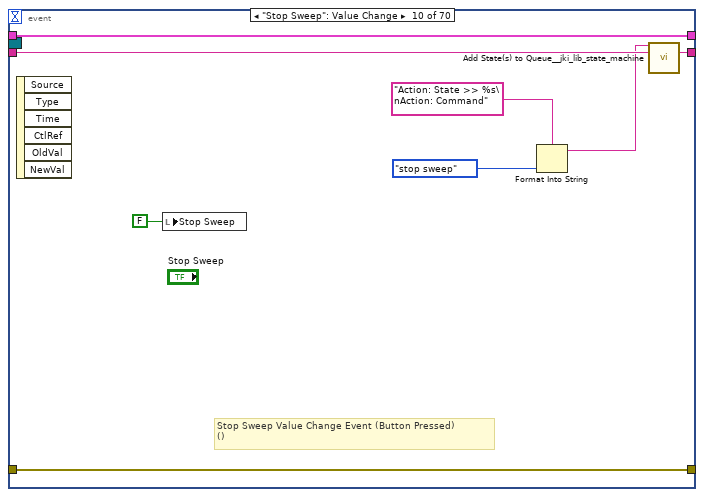
[diagram p19: hidden frame]
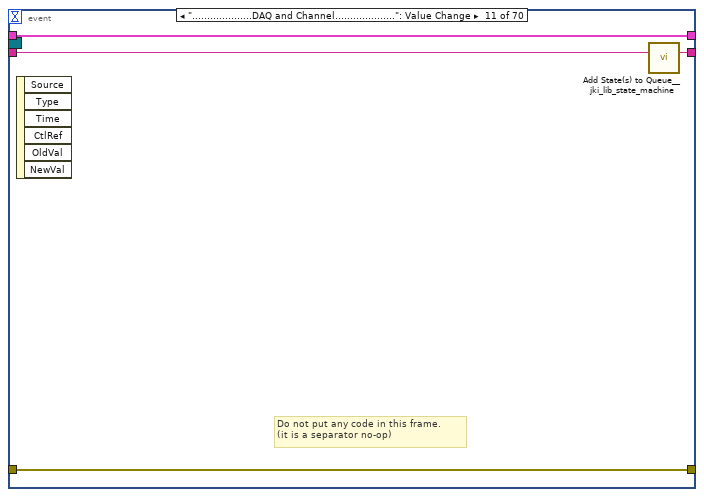
[diagram p20: hidden frame]
diagram:
  w1 = T26."AO/AI"  # Right Tab
  w2 = T1."AO/AI/REF"  # Left Tab
  (unwired) Lockin.Commands.Local--Enum."setOffset" ("Locking.Commands.Local")
  (unwired) Lockin.Commands--Enum."setAO" ("Locking.Commands")
  # "These are just to have separators in the event structure:"
  # "For instructions on how to use the JKI State Machine Objects, examples and video tutorials, visit:\nhttp://jki.net/state-machine-objects/\n\nJKI State Machine Objects™\nhttp://jki.net/state-machine-objects/\nCopyright (C) 2005-2015, JKI <info@jki.net>\nALL RIGHTS RESERVED"
  n1 = call <vilib>:"Register Process (Default).vi"("error in (no error)"="error in", "SMO"="Lockin.UI") -> ("error out"=w7:errorcluster, "SelfRef"=w6:refnum<class "Instrument UI.Lockin.lvclass">)  [unwired: 8 in]
  n2 = case shown="No Error" w7 {
    selector: w7 -> [w12 w2205]
    tunnel: w6 -> [w13 _]
    tunnel: [w11 w2205] -> w3
    frame No Error {
      # "State Syntax:\nStateCategory: State >> Argument\nLine Terminator: Line feed\nExample:\nUI: Help >> About\n\nWhere \"UI\" is the state category\nWhere \"Help\" is the state\nWhere \"About\" is the argument\nOther Examples:\nApp Data: Initialize\nUI: Initialize\nHelp >> About\n\nCommenting:\nTo add a comment use \"//\" or \"#\" and all text to the right will be ignored\nCommenting Example:\nUI: Initialize // This initializes the UI\n# This whole line is a comment\n// Another comment line"
      # "copy this to create labels for wires"
      # "System_Label"
      n3 = call <vilib>:"Add State(s) to Queue__jki_lib_state_machine.vi"("State(s) in (\"\")"="Macro: Initialize") -> ("States Out"=w15:string)  [unwired: 14 in]
      n4 = while "JKI - String-Based Queued State Machine (Basic) v1.0" {
        shift-right: [w24] -> _
        shift-left: _ -> [w23]
        shift-right: [w27] -> w11
        shift-left: w12 -> [w21]
        shift-right: [w26] -> _
        shift-left: w15 -> [w28]
        tunnel: w13 -> [w20]
        shift-right: [w19] -> _
        shift-left: _ -> [w18]
        stop <- w25 stop-if-true
        # "Template Copyright © 2008 JKI - http://jkisoft.com/state-machine"
        n5 = call <vilib>:"Parse State Queue__jki_lib_state_machine.vi"("State Queue"=w28, "Error In (no error)"=w21) -> ("Remaining States"=w30:string, "Current State"=w17:string, "Arguments"=w29:string)  [unwired: 11 in]
        n6 = call "Instrument UI.Lockin.State History.vi"("Current State"=w17) -> ("History"=→"State History":string)  [unwired: 10 in]
        n7 = case shown="\"UI: UI to Cluster 2\"" w17 {
          selector: w17 -> [_ _ w732 _ _ _ _ _ _ _ _ _ _ _ _ _ _ _ _ _ _ _ _ _ _ _ _ _ _ _ _ _ _ _ _ _ _ _ _ _ _ _ _ _ _ _ _ _ _ _ _ _ _ _ _ _ _ _ _ _ _ _ _ _ _ _ _ _ _ _ _ _ _ _ _ _ _ _ _ _ _ _ _ _ _ _ _ _ _ _ _ _ _ _ _ _ _ _ _ _ _ _ _ _ _ _ _ _ _ _ _ _ _]
          tunnel: w30 -> [w38 w730 w736 w755 w758 w774 w779 w799 w821 w838 w846 w853 w858 w872 w882 w895 w900 w911 w919 w927 w933 w962 w973 w1002 w1014 w1023 w1031 w1040 w1053 w1066 w1085 w1107 w1137 w1164 w1186 w1207 w1237 w1264 w1293 w1326 w1352 w1383 w1430 w1453 w1461 w1488 w1502 w1512 w1531 w1540 w1549 w1569 w1580 w1589 w1598 w1608 w1620 w1637 w1645 w1677 w1688 w1700 w1711 w1720 w1729 w1743 w1753 w1774 w1783 w1800 w1805 w1816 w1823 w1828 w1847 w1853 w1860 w1865 w1872 w1880 w1896 w1908 w1918 w1936 w1943 w1951 w1959 w1967 w1977 w1988 w1996 w2004 w2014 w2024 w2032 w2040 w2048 w2056 w2064 w2072 w2080 w2088 w2096 w2104 w2113 w2124 w2135 w2148 w2158 w2165 w2184 w2192 w2204]
          tunnel: w29 -> [_ _ _ _ _ _ _ _ _ _ w839 _ _ _ _ _ _ _ w914 w922 w928 _ _ _ _ _ _ _ w1045 w1058 w1079 _ _ _ _ _ _ _ _ _ _ _ _ _ _ _ _ _ _ _ _ _ _ _ _ w1600 w1614 w1630 w1639 _ _ _ _ _ _ _ _ _ _ _ _ _ _ _ _ _ _ _ _ _ _ w1901 w1912 w1930 _ _ _ _ _ _ _ _ _ _ _ _ _ _ _ _ _ _ _ _ _ _ _ w2141 w2151 _ _ _ _]
          tunnel: w23 -> [w36 w727 w734 w746 w761 w770 w776 _ w801 w827 w843 w848 w855 w868 w878 w891 w897 w905 w916 w924 w930 w943 w969 w997 w1003 w1015 w1026 w1036 w1047 w1060 w1080 w1104 w1123 w1161 w1183 w1204 w1234 w1261 w1290 w1323 w1349 w1380 w1414 w1450 w1457 w1485 w1496 w1505 w1528 w1536 w1542 w1565 w1576 w1584 w1595 w1601 w1618 w1633 w1641 w1674 w1684 w1690 w1708 w1717 w1726 w1740 w1747 w1759 w1780 w1786 w1802 w1813 w1818 w1825 w1845 w1851 w1854 w1861 w1868 w1876 w1889 w1903 w1913 w1931 w1938 w1946 w1954 w1962 w1968 w1983 w1991 w1999 w2009 w2019 w2027 w2035 w2043 w2051 w2059 w2067 w2075 w2083 w2091 w2099 w2108 w2119 w2128 w2143 w2153 w2160 w2181 w2186 w2198]
          tunnel: [w35 w728 w738 w752 w763 w769 w777 w789 w819 w836 w844 w849 w856 w860 w877 w886 w898 w907 w917 w925 w931 w960 w971 w1000 w1012 w1021 w1029 w1038 w1049 w1057 w1075 w1094 w1127 w1160 w1181 w1202 w1233 w1260 w1289 w1322 w1343 w1374 w1409 w1444 w1459 w1483 w1500 w1510 w1524 w1538 w1547 w1567 w1574 w1581 w1592 w1606 w1615 w1635 w1642 w1675 w1686 w1698 w1709 w1718 w1727 w1741 w1745 w1768 w1781 w1798 w1803 w1807 w1819 w1826 w1843 w1848 w1857 w1862 w1866 w1873 w1890 w1905 w1915 w1933 w1940 w1948 w1956 w1964 w1974 w1985 w1993 w2001 w2011 w2021 w2029 w2037 w2045 w2053 w2061 w2069 w2077 w2085 w2093 w2101 w2110 w2121 w2132 w2145 w2155 w2162 w2179 w2189 w2201] -> w27
          tunnel: w21 -> [w34 w728 w737 w752 w766 _ w777 w788 w819 w836 w844 w850 w856 w866 w875 w887 w898 w908 w917 w925 w931 w960 w971 w1000 w1012 w1021 w1029 w1038 w1048 w1061 w1081 w1091 w1124 w1155 w1177 w1195 w1229 w1256 w1285 w1318 w1341 w1372 w1408 w1443 w1459 w1484 w1500 w1510 w1524 w1538 w1547 w1567 w1577 w1582 w1591 w1606 w1616 w1635 w1643 w1675 w1686 w1698 w1709 w1718 w1727 w1741 w1746 w1767 w1781 w1798 w1803 w1808 w1820 w1826 w1838 w1849 w1857 w1862 w1867 w1874 w1891 w1905 w1915 w1933 w1940 w1948 w1956 w1964 w1974 w1985 w1993 w2001 w2011 w2021 w2029 w2037 w2045 w2053 w2061 w2069 w2077 w2085 w2093 w2101 w2110 w2121 w2132 w2145 w2155 w2162 w2178 w2189 w2201]
          tunnel: [w37 w729 w735 w754 w757 w773 w778 w798 w820 w837 w845 w852 w857 w871 w881 w894 w899 w910 w918 w926 w932 w961 w972 w1001 w1013 w1022 w1030 w1039 w1052 w1065 w1084 w1106 w1136 w1163 w1185 w1206 w1236 w1263 w1292 w1325 w1351 w1382 w1429 w1452 w1460 w1487 w1501 w1511 w1530 w1539 w1548 w1568 w1579 w1588 w1597 w1607 w1619 w1636 w1644 w1676 w1687 w1699 w1710 w1719 w1728 w1742 w1752 w1773 w1782 w1799 w1804 w1815 w1822 w1827 w1846 w1852 w1859 w1864 w1871 w1879 w1895 w1907 w1917 w1935 w1942 w1950 w1958 w1966 w1976 w1987 w1995 w2003 w2013 w2023 w2031 w2039 w2047 w2055 w2063 w2071 w2079 w2087 w2095 w2103 w2112 w2123 w2134 w2147 w2157 w2164 w2183 w2191 w2203] -> w26
          tunnel: [_ _ _ _ _ TRUE _ _ _ _ _ _ _ _ _ _ _ _ _ _ _ _ _ _ _ _ _ _ _ _ _ _ _ _ _ _ _ _ _ _ _ _ _ _ _ _ _ _ _ _ _ _ _ _ _ _ _ _ _ _ _ _ _ _ _ _ _ _ _ _ _ _ _ _ _ _ _ _ _ _ _ _ _ _ _ _ _ _ _ _ _ _ _ _ _ _ _ _ _ _ _ _ _ _ _ _ _ _ _ _ _ _ _] -> w25
          tunnel: [w33 w727 w734 w753 w760 w770 w776 w797 w817 w826 w843 w848 w855 w869 w879 w892 w897 w905 w916 w924 w930 w943 w969 w998 w1004 w1015 w1026 w1036 w1047 w1060 w1080 w1103 w1123 w1161 w1183 w1204 w1234 w1261 w1290 w1323 w1349 w1380 w1414 w1450 w1457 w1485 w1496 w1505 w1528 w1536 w1542 w1565 w1576 w1584 w1595 w1602 w1618 w1633 w1641 w1674 w1684 w1691 w1708 w1717 w1726 w1740 w1749 w1760 w1780 w1787 w1802 w1813 w1818 w1825 w1845 w1851 w1855 w1861 w1868 w1877 w1893 w1904 w1914 w1932 w1939 w1947 w1955 w1963 w1969 w1984 w1992 w2000 w2010 w2020 w2028 w2036 w2044 w2052 w2060 w2068 w2076 w2084 w2092 w2100 w2109 w2120 w2131 w2144 w2154 w2161 w2181 w2187 w2199] -> w24
          tunnel: 50 ("Timeout") -> [w32 _ _ _ _ _ _ _ _ _ _ _ _ _ _ _ _ _ _ _ _ _ _ _ _ _ _ _ _ _ _ _ _ _ _ _ _ _ _ _ _ _ _ _ _ _ _ _ _ _ _ _ _ _ _ _ _ _ _ _ _ _ _ _ _ _ _ _ _ _ _ _ _ _ _ _ _ _ _ _ _ _ _ _ _ _ _ _ _ _ _ _ _ _ _ _ _ _ _ _ _ _ _ _ _ _ _ _ _ _ _ _ _]
          tunnel: w20 -> [_ _ _ _ _ _ _ w790 _ _ _ _ _ _ _ _ _ _ _ _ _ _ _ _ _ _ _ _ _ _ _ _ _ _ _ _ _ _ _ _ _ _ _ _ _ _ _ _ _ _ _ _ _ _ _ _ _ _ _ _ _ _ _ _ _ _ _ _ _ _ _ _ _ _ _ _ _ _ _ _ _ _ _ _ _ _ _ _ _ _ _ _ _ _ _ _ _ _ _ _ _ _ _ _ _ _ _ _ _ _ _ _ _]
          tunnel: [w31 w726 w731 w743 w768 w771 w775 w796 w818 w835 w842 w847 w854 w870 w880 w893 w896 w909 w915 w923 w929 w959 w970 w999 w1011 w1020 w1028 w1037 w1051 w1064 w1083 w1105 w1135 w1162 w1184 w1205 w1235 w1262 w1291 w1324 w1350 w1381 w1428 w1451 w1458 w1486 w1499 w1509 w1529 w1537 w1546 w1566 w1578 w1587 w1596 w1605 w1617 w1634 w1638 w1673 w1685 w1697 w1707 w1716 w1725 w1739 w1751 w1772 w1779 w1793 w1801 w1814 w1821 w1824 w1844 w1850 w1858 w1863 w1870 w1875 w1894 w1906 w1916 w1934 w1941 w1949 w1957 w1965 w1975 w1986 w1994 w2002 w2012 w2022 w2030 w2038 w2046 w2054 w2062 w2070 w2078 w2086 w2094 w2102 w2111 w2122 w2133 w2146 w2156 w2163 w2182 w2190 w2202] -> w19
          tunnel: w18 -> [w31 w726 w731 w743 w768 w771 w775 w796 w818 w835 w842 w847 w854 w870 w880 w893 w896 w909 w915 w923 w929 w959 w970 w999 w1011 w1020 w1028 w1037 w1051 w1064 w1083 w1105 w1135 w1162 w1184 w1205 w1235 w1262 w1291 w1324 w1350 w1381 w1428 w1451 w1458 w1486 w1499 w1509 w1529 w1537 w1546 w1566 w1578 w1587 w1596 w1605 w1617 w1634 w1638 w1673 w1685 w1697 w1707 w1716 w1725 w1739 w1751 w1772 w1779 w1793 w1801 w1814 w1821 w1824 _ w1850 w1858 w1863 w1870 w1875 w1894 w1906 w1916 w1934 w1941 w1949 w1957 w1965 w1975 w1986 w1994 w2002 w2012 w2022 w2030 w2038 w2046 w2054 w2062 w2070 w2078 w2086 w2094 w2102 w2111 w2122 w2133 w2146 w2156 w2163 w2182 w2190 w2202]
          frame "", "Idle" {
            # "executes when the state queue is empty"
            n8 = event shown="[28] \"Limit DC (V)\", \"AO DC Limit\": Value Change" {
              selector: w31 -> [_ _ _ _ _ _ _ _ _ _ _ _ _ _ _ _ _ _ _ _ _ _ _ _ _ _ _ _ _ _ _ _ _ _ _ _ _ _ _ _ _ _ _ _ _ _ _ _ _ _ _ _ _ _ _ _ _ _ _ _ _ _ _ _ _ _ _ _ _ _]
              dyn-events: _ -> [_ _ _ _ _ _ _ _ _ _ _ _ _ _ _ _ _ _ _ _ _ _ _ _ _ _ _ _ _ _ _ _ _ _ _ _ _ _ _ _ _ _ _ _ _ _ _ _ _ _ _ _ _ _ _ _ _ _ _ _ _ _ _ _ _ _ _ _ _ _]
              timeout: w32 -> [_ _ _ _ _ _ _ _ _ _ _ _ _ _ _ _ _ _ _ _ _ _ _ _ _ _ _ _ _ _ _ _ _ _ _ _ _ _ _ _ _ _ _ _ _ _ _ _ _ _ _ _ _ _ _ _ _ _ _ _ _ _ _ _ _ _ _ _ _ _]
              tunnel: w38 -> [w51 w92 w100 w114 w118 w128 w137 w145 w153 w161 w165 w171 w178 w188 w205 w222 w241 w254 w267 w280 w292 w299 w306 w313 w320 w327 w334 w342 w350 w358 w364 w373 w389 w402 w410 w418 w426 w433 w440 w444 w449 w454 w459 w464 w478 w492 w504 w516 w521 w526 w530 w535 w540 w544 w548 w554 w576 w629 w636 w643 w650 w657 w664 w671 w688 w695 w704 w711 w718 w725]
              tunnel: [w50 w91 w99 w113 w117 w127 w136 w144 w152 w160 w164 w170 w177 w187 w204 w221 w240 w253 w266 w279 w291 w298 w305 w312 w319 w326 w333 w341 w349 w357 w363 w372 w388 w401 w409 w417 w425 w432 w439 w443 w448 w453 w458 w463 w477 w491 w503 w515 w520 w525 w529 w534 w539 w543 w547 w553 w575 w628 w635 w642 w649 w656 w663 w670 w687 w694 w703 w710 w717 w724] -> w37
              tunnel: w36 -> [w48 w89 w97 w111 w116 w120 w129 w138 w149 w155 w163 w166 w173 w183 w200 w212 w236 w248 w260 w273 w287 w294 w301 w308 w315 w322 w329 w337 w345 w353 w359 w368 w376 w395 w403 w414 w422 w430 w437 w442 w445 w450 w455 w460 w475 w489 w501 w513 w518 w523 w528 w532 w537 w541 w545 w551 w570 w625 w632 w638 w645 w652 w659 w666 w680 w690 w699 w706 w713 w720]
              tunnel: [w49 w90 w96 w110 w115 w125 w134 w142 w150 w158 w162 w167 w175 w186 w203 w216 w239 w252 w265 w278 w289 w296 w303 w310 w317 w324 w331 w339 w347 w355 w360 w370 w386 w399 w407 w415 w423 w431 w438 w441 w446 w451 w456 w461 w476 w490 w502 w514 w517 w522 w527 w533 w538 w542 w546 w552 w574 w616 w630 w641 w648 w655 w662 w669 w686 w693 w702 w709 w716 w723] -> w35
              tunnel: w34 -> [w49 w90 w95 w110 w115 w125 w134 w142 w150 w158 w162 w167 w175 w186 w203 w216 w239 w252 w265 w278 w289 w296 w303 w310 w317 w324 w331 w339 w347 w355 w360 w370 w386 w399 w407 w415 w423 w431 w438 w441 w446 w451 w456 w461 w476 w490 w502 w514 w517 w522 w527 w533 w538 w542 w546 w552 w574 w615 w630 w641 w648 w655 w662 w669 w686 w693 w702 w709 w716 w723]
              tunnel: [w48 w89 w97 w111 w116 w121 w129 w138 w149 w155 w163 w166 w174 w185 w202 w215 w238 w251 w264 w277 w288 w295 w302 w309 w316 w323 w330 w338 w346 w354 w359 w369 w385 w395 w403 w414 w422 w430 w437 w442 w445 w450 w455 w460 w475 w489 w501 w513 w518 w523 w528 w532 w537 w541 w545 w551 w573 w626 w633 w639 w646 w653 w660 w667 w685 w691 w700 w707 w714 w721] -> w33
              event Timeout {
                n9 = event-data() -> ()  [unwired: 1 in, 1 out]
                n10 = Unbundle By Name(w48) -> ("DAQ state"=w47:T22)
                n11 = call <userlib>:"Periodic Trigger__ogtk.vi"("time (ms)"=u32 100) -> ("Triggered"=w45:bool)  [unwired: 12 in, 2 out]
                n12 = call <userlib>:"Periodic Trigger__ogtk.vi"("time (ms)"=u32 600000) -> ("Triggered"=w42:bool)  [unwired: 12 in, 2 out]
                n13 = case shown="True" w45 {
                  tunnel: w47 -> [_ w56]
                  tunnel: ["" ("States Out") w55] -> w40
                  frame False {
                  }
                  frame True {
                    n14 = case shown="\"idle\"" w56 {
                      tunnel: [w57 w63 w69 w75 ""] -> w55
                      frame "idle" {
                        n15 = call "Spinner.vi"("Enum"=enum16{"Spinner 1", "Spinner 2", "Spinner 3"}."Spinner 1") -> ("Spinner Out"=w60:string)  [unwired: 4 in]
                        n16 = Concatenate Strings("Idle     " ("Status"), w60) -> (w58:string)
                        n17 = call <vilib>:"Build State String with Arguments__JKI_lib_State_Machine.vi"("Arguments (\"\")"=w58, "State"="UI: Update Status") -> ("State with Arguments"=w57:string)  [unwired: 4 in]
                      }
                      frame "created" {
                        n18 = call "Spinner.vi"("Enum"=enum16{"Spinner 1", "Spinner 2", "Spinner 3"}."Spinner 1") -> ("Spinner Out"=w66:string)  [unwired: 4 in]
                        n19 = Concatenate Strings("Created  " ("Status"), w66) -> (w64:string)
                        n20 = call <vilib>:"Build State String with Arguments__JKI_lib_State_Machine.vi"("Arguments (\"\")"=w64, "State"="UI: Update Status") -> ("State with Arguments"=w63:string)  [unwired: 4 in]
                      }
                      frame "started" {
                        n21 = call "Spinner.vi"("Enum"=T30."Spinner 4") -> ("Spinner Out"=w73:string)  [unwired: 4 in]
                        n22 = Concatenate Strings("Started  " ("Status"), w73) -> (w70:string)
                        n23 = call <vilib>:"Build State String with Arguments__JKI_lib_State_Machine.vi"("Arguments (\"\")"=w70, "State"="UI: Update Status") -> ("State with Arguments"=w69:string)  [unwired: 4 in]
                      }
                      frame "sweeping" {
                        n24 = call "Spinner.vi"("Enum"=T30."Spinner 3") -> ("Spinner Out"=w81:string)  [unwired: 4 in]
                        n25 = Concatenate Strings("Sweeping  ", w81) -> (w77:string)
                        n26 = call <vilib>:"Build State String with Arguments__JKI_lib_State_Machine.vi"("Arguments (\"\")"=w77, "State"="UI: Update Status") -> ("State with Arguments"=w78:string)  [unwired: 4 in]
                        n27 = call <vilib>:"Add State(s) to Queue__jki_lib_state_machine.vi"("State(s) in Front (\"\")"=w78, "State(s) at Back (\"\")"="UI: Update Sweep Timer") -> ("States Out"=w75:string)  [unwired: 13 in]
                      }
                      frame Default {
                      }
                    }
                  }
                }
                n28 = case shown="True" w42 {
                  tunnel: ["" "Macro: Save Configuration"] -> w41
                  frame False {
                  }
                  frame True {
                    # "Backup configuration every 10 minutes"
                  }
                }
                n29 = call <userlib>:"MGI Milliseconds Since Last Call.vi"() -> ("ms"=→"UI Refresh time (ms)":u32)  [unwired: 6 in, 1 out]
                n30 = call <vilib>:"Add State(s) to Queue__jki_lib_state_machine.vi"("State(s) in Front (\"\")"=w40, "State(s) at Back (\"\")"=w41) -> ("States Out"=w39:string)  [unwired: 13 in]
                n31 = call <vilib>:"Add State(s) to Queue__jki_lib_state_machine.vi"("State(s) in Front (\"\")"=w39, "State(s) in (\"\")"=w51) -> ("States Out"=w50:string)  [unwired: 13 in]
              }
              event "Close": Value Change {
                # "Hide this FP control 2022-08-15"
                n32 = event-data() -> ()  [unwired: 1 in, 6 out]
                n33 = Two Button Dialog(message="Are you sure you want to stop this program?") -> (T button?=w84:bool)  [unwired: 2 in]
                n34 = Select(t="Action: Notify UI Closed\nMacro: Exit", s=w84, f="") -> (s? t:f=w85:string)
                n35 = local write "Close"(w84) -> ()
                n36 = call <vilib>:"Add State(s) to Queue__jki_lib_state_machine.vi"("State(s) in Front (\"\")"=w85, "State(s) in (\"\")"=w92) -> ("States Out"=w91:string)  [unwired: 13 in]
              }
              event "Help": Value Change {
                # "HELP Value Change Event (Button Pressed)\n(If Help = True: Send user to help webpage; Set Help=False\nIf Help=False, Do nothing)"
                n37 = event-data() -> ("NewVal"=w94:bool)  [unwired: 1 in, 5 out]
                n38 = local write "Help"(FALSE ("Help")) -> ()
                n39 = case shown="True" w94 {
                  tunnel: w95 -> [w101 w104]
                  tunnel: [w101 w103] -> w96
                  frame False {
                  }
                  frame True {
                    n40 = call-poly <vilib>:"Open URL in Default Browser.vi"("error in (no error)"=w104, "URL"="https://github.com/levylabpitt/Multichannel-Lockin") -> ("error out"=w103:errorcluster)  [unwired: 4 in, 1 out]
                  }
                }
                n41 = call <vilib>:"Add State(s) to Queue__jki_lib_state_machine.vi"("State(s) in Front (\"\")"="", "State(s) in (\"\")"=w100) -> ("States Out"=w99:string)  [unwired: 13 in]
              }
              event Panel Close? {
                # "Discard the event because we'll close the front panel ourselves in Macro: Exit"
                # "Close Panel button (pressed) Event\n(this executes Macro: Exit to terminate the VI)"
                n42 = event-data() -> ()  [unwired: 1 in, 1 out]
                n43 = Two Button Dialog(message="Are you sure you want to stop this program?") -> (T button?=w109:bool)  [unwired: 2 in]
                n44 = Select(t="Action: Notify UI Closed\nMacro: Exit", s=w109, f="") -> (s? t:f=w105:string)
                n45 = event-data("Discard?"=TRUE) -> ()  [unwired: 1 in, 1 out]
                n46 = call <vilib>:"Add State(s) to Queue__jki_lib_state_machine.vi"("State(s) in Front (\"\")"=w105, "State(s) in (\"\")"=w114) -> ("States Out"=w113:string)  [unwired: 13 in]
              }
              event "....................State....................": Value Change {
                # "Do not put any code in this frame.\n(it is a separator no-op)"
                n47 = event-data() -> ()  [unwired: 1 in, 6 out]
                n48 = call <vilib>:"Add State(s) to Queue__jki_lib_state_machine.vi"("State(s) in (\"\")"=w118) -> ("States Out"=w117:string)  [unwired: 14 in]
              }
              event "Start": Value Change {
                w119 = T42 10123 items=["Finite Samples"=10178, "Continuous Samples"=10123] ("UI Config.DAQ.Sampling.Sample Mode")
                # "Start Button Change Event (Button Pressed)\n()"
                n49 = event-data() -> ()  [unwired: 1 in, 6 out]
                n50 = local write "Start"(FALSE ("Help")) -> ()
                n51 = Bundle By Name(cluster=w120, "UI Config.DAQ.cfg.Sampling.sample mode"=w119) -> (w121:T63)
                n52 = Format Into String(format string="//Action: Sampling Mode\n//Action: Command\nAction: State >> %s\nAction: Command", Set_State-enum."start" ("State")) -> (resulting string=w122:string)  [unwired: 2 in, 1 out]
                n53 = call <vilib>:"Add State(s) to Queue__jki_lib_state_machine.vi"("State(s) in Front (\"\")"=w122, "State(s) in (\"\")"=w128) -> ("States Out"=w127:string)  [unwired: 13 in]
              }
              event "Pause": Value Change {
                w130 = T42 10178 items=["Finite Samples"=10178, "Continuous Samples"=10123] ("UI Config.DAQ.Sampling.Sample Mode")
                # "Start Button Change Event (Button Pressed)\n()"
                n54 = event-data() -> ()  [unwired: 1 in, 6 out]
                n55 = local write "Pause"(FALSE ("Help")) -> ()
                n56 = Bundle By Name(cluster=w129, "UI Config.DAQ.cfg.Sampling.sample mode"=w130) -> ()  [unwired: 1 out]
                n57 = Format Into String(format string="//Action: Sampling Mode\n//Action: Command\nAction: State >> %s\nAction: Command\nAction: Flush Queue", Set_State-enum."stop" ("State")) -> (resulting string=w131:string)  [unwired: 2 in, 1 out]
                n58 = call <vilib>:"Add State(s) to Queue__jki_lib_state_machine.vi"("State(s) in Front (\"\")"=w131, "State(s) in (\"\")"=w137) -> ("States Out"=w136:string)  [unwired: 13 in]
              }
              event "Reset": Value Change {
                # "Start Button Change Event (Button Pressed)\n()"
                n59 = event-data() -> ()  [unwired: 1 in, 6 out]
                n60 = local write "Reset"(FALSE ("Help")) -> ()
                n61 = Format Into String(format string="Action: State >> %s\nAction: Command", Set_State-enum."reset" ("State")) -> (resulting string=w139:string)  [unwired: 2 in, 1 out]
                n62 = call <vilib>:"Add State(s) to Queue__jki_lib_state_machine.vi"("State(s) in Front (\"\")"=w139, "State(s) in (\"\")"=w145) -> ("States Out"=w144:string)  [unwired: 13 in]
              }
              event "Start Sweep": Value Change {
                # "Stop Sweep Value Change Event (Button Pressed)\n()"
                n63 = event-data() -> ()  [unwired: 1 in, 6 out]
                n64 = local write "Start Sweep"(FALSE ("Help")) -> ()
                n65 = Format Into String(format string="Action: State >> %s\nAction: Command", Set_State-enum."start sweep" ("State")) -> (resulting string=w147:string)  [unwired: 2 in, 1 out]
                n66 = call <vilib>:"Add State(s) to Queue__jki_lib_state_machine.vi"("State(s) in Front (\"\")"=w147, "State(s) in (\"\")"=w153) -> ("States Out"=w152:string)  [unwired: 13 in]
              }
              event "Stop Sweep": Value Change {
                # "Stop Sweep Value Change Event (Button Pressed)\n()"
                n67 = event-data() -> ()  [unwired: 1 in, 6 out]
                n68 = local write "Stop Sweep"(FALSE ("Help")) -> ()
                n69 = Format Into String(format string="Action: State >> %s\nAction: Command", Set_State-enum."stop sweep" ("State")) -> (resulting string=w154:string)  [unwired: 2 in, 1 out]
                n70 = call <vilib>:"Add State(s) to Queue__jki_lib_state_machine.vi"("State(s) in Front (\"\")"=w154, "State(s) in (\"\")"=w161) -> ("States Out"=w160:string)  [unwired: 13 in]
              }
              event "....................DAQ and Channel....................": Value Change {
                # "Do not put any code in this frame.\n(it is a separator no-op)"
                n71 = event-data() -> ()  [unwired: 1 in, 6 out]
                n72 = call <vilib>:"Add State(s) to Queue__jki_lib_state_machine.vi"("State(s) in (\"\")"=w165) -> ("States Out"=w164:string)  [unwired: 14 in]
              }
              event "Auto DAQ": Value Change {
                # "auto DAQ Value Change Event (Button Pressed)\n()"
                n73 = event-data() -> ()  [unwired: 1 in, 6 out]
                n74 = local write "Auto DAQ"(FALSE ("Help")) -> ()
                n75 = call <vilib>:"Add State(s) to Queue__jki_lib_state_machine.vi"("State(s) in Front (\"\")"="Action: Auto DAQ\nAction: Command", "State(s) in (\"\")"=w171) -> ("States Out"=w170:string)  [unwired: 13 in]
              }
              event Value Change {
                # "DAQ Config Value Change Event (Button Pressed)\n()"
                n76 = event-data() -> ()  [unwired: 1 in, 6 out]
                n77 = Bundle By Name(cluster=w173, "UI Config.DAQ.Configuration"="DAQ Config") -> (w174:T63)
                n78 = call <vilib>:"Add State(s) to Queue__jki_lib_state_machine.vi"("State(s) in Front (\"\")"="Action: DAQ Config\nAction: Command", "State(s) in (\"\")"=w178) -> ("States Out"=w177:string)  [unwired: 13 in]
              }
              event "Fs (S/s)", "#s (S)": Value Change {
                # "DAQ Config Value Change Event (Button Pressed)\n()"
                n79 = event-data() -> ()  [unwired: 1 in, 6 out]
                n80 = local read "Fs Output (S/s)"() -> (w179:dbl)
                n81 = Unbundle By Name(w183) -> ("DAQ state"=w182:T22)
                n82 = property on="Fs Output (S/s)" class="DigNum (strict)"("Val(Sgnl)"=w179) -> ()  [unwired: 2 in, 2 out]
                n83 = Bundle By Name(cluster=w183, "UI Config.DAQ.cfg.Sampling.Sampling.Fs"="Fs (S/s)", "UI Config.DAQ.cfg.Sampling.Sampling.#s"="#s (S)") -> (w185:T63)
                n84 = case shown="\"started\"" w182 {
                  tunnel: ["Action: Sampling\nAction: Command" w191] -> w184
                  frame Default {
                  }
                  frame "started" {
                    n85 = Format Into String(format string="Action: State >> %s\nAction: Command\nAction: Sampling\nAction: Command\nAction: State >> %s\nAction: Command", Set_State-enum."stop" ("State"), Set_State-enum."start" ("State")) -> (resulting string=w191:string)  [unwired: 2 in, 1 out]
                  }
                }
                n86 = call <vilib>:"Add State(s) to Queue__jki_lib_state_machine.vi"("State(s) in Front (\"\")"=w184, "State(s) in (\"\")"=w188) -> ("States Out"=w187:string)  [unwired: 13 in]
              }
              event "Fs Output (S/s)": Value Change {
                # "DAQ Config Value Change Event (Button Pressed)\n()"
                n87 = event-data() -> ()  [unwired: 1 in, 6 out]
                n88 = Unbundle By Name(w200) -> ("UI Config.DAQ.cfg.Sampling.Sampling.Fs"=w197:dbl, "UI Config.DAQ.cfg.Sampling.Sampling.#s"=w198:i32, "DAQ state"=w199:T22)
                n89 = Divide(x=w197, y=w198) -> (x/y=w196:dbl)
                n90 = In Range and Coerce(upper limit=w197, x="Fs Output (S/s)", lower limit=w196) -> (coerced(x)=w194:dbl)  [unwired: 1 out]
                n91 = local write "Fs Output (S/s)"(w194) -> ()
                n92 = Bundle By Name(cluster=w200, "UI Config.DAQ.cfg.Sampling.Fs.Output"=w194) -> (w202:T63)
                n93 = case shown="Default" w199 {
                  tunnel: ["Action: Sampling Fs Output\nAction: Command" w208] -> w201
                  frame Default {
                  }
                  frame "started" {
                    n94 = Format Into String(format string="Action: State >> %s\nAction: Command\nAction: Sampling Fs Output\nAction: Command\nAction: State >> %s\nAction: Command", Set_State-enum."stop" ("State"), Set_State-enum."start" ("State")) -> (resulting string=w208:string)  [unwired: 2 in, 1 out]
                  }
                }
                n95 = call <vilib>:"Add State(s) to Queue__jki_lib_state_machine.vi"("State(s) in Front (\"\")"=w201, "State(s) in (\"\")"=w205) -> ("States Out"=w204:string)  [unwired: 13 in]
              }
              event Value Change {
                n96 = event-data() -> ()  [unwired: 1 in, 6 out]
                n97 = control-ref of="Fs Multiplier"() -> (w220:refnum<vi>)
                n98 = control-ref of="Refresh Rate (Hz)"() -> (w219:refnum<vi>)
                n99 = Bundle By Name(cluster=w212, "UI Config.DAQ.cfg.Sampling.Fs Mode"="Fs Mode") -> (w215:T63)
                n100 = Unbundle By Name(w212) -> ("DAQ state"=w213:T22)
                n101 = case shown="\"Manual\"" "Fs Mode" {
                  tunnel: [FALSE ("Visible") TRUE ("Visible") FALSE ("Visible")] -> w218
                  tunnel: [FALSE ("Visible") FALSE ("Visible") TRUE ("Visible")] -> w217
                  frame "Manual" {
                  }
                  frame "Auto Fs" {
                  }
                  frame "Max Fs" {
                  }
                }
                n102 = case shown="Default" w213 {
                  tunnel: ["Action: Sampling Fs Mode\nAction: Command" w225] -> w211
                  frame Default {
                  }
                  frame "started" {
                    n103 = Format Into String(format string="Action: State >> %s\nAction: Command\nAction: Sampling Fs Mode\nAction: Command\nAction: State >> %s\nAction: Command", Set_State-enum."stop" ("State"), Set_State-enum."start" ("State")) -> (resulting string=w225:string)  [unwired: 2 in, 1 out]
                  }
                }
                n104 = property class="DigNum (strict)"(reference=w220, "Visible"=w218) -> ()  [unwired: 1 in, 2 out]
                n105 = property class="DigNum (strict)"(reference=w219, "Visible"=w217) -> ()  [unwired: 1 in, 2 out]
                n106 = call <vilib>:"Add State(s) to Queue__jki_lib_state_machine.vi"("State(s) in Front (\"\")"=w211, "State(s) in (\"\")"=w222) -> ("States Out"=w221:string)  [unwired: 13 in]
              }
              event "Fs Multiplier": Value Change {
                # "DAQ Config Value Change Event (Button Pressed)\n()"
                n107 = event-data() -> ()  [unwired: 1 in, 6 out]
                n108 = Unbundle By Name(w236) -> ("DAQ state"=w234:T22)
                n109 = Bundle By Name(cluster=w236, "UI Config.DAQ.cfg.Sampling.Fs Multiplier"="Fs Multiplier") -> (w238:T63)
                n110 = case shown="Default" w234 {
                  tunnel: ["Action: Sampling Fs Multiplier\nAction: Command" w244] -> w235
                  frame Default {
                  }
                  frame "started" {
                    n111 = Format Into String(format string="Action: State >> %s\nAction: Command\nAction: Sampling Fs Multiplier\nAction: Command\nAction: State >> %s\nAction: Command", Set_State-enum."stop" ("State"), Set_State-enum."start" ("State")) -> (resulting string=w244:string)  [unwired: 2 in, 1 out]
                  }
                }
                n112 = call <vilib>:"Add State(s) to Queue__jki_lib_state_machine.vi"("State(s) in Front (\"\")"=w235, "State(s) in (\"\")"=w241) -> ("States Out"=w240:string)  [unwired: 13 in]
              }
              event "Refresh Rate (Hz)": Value Change {
                # "DAQ Config Value Change Event (Button Pressed)\n()"
                n113 = event-data() -> ()  [unwired: 1 in, 6 out]
                n114 = Unbundle By Name(w248) -> ("DAQ state"=w249:T22)
                n115 = Bundle By Name(cluster=w248, "UI Config.DAQ.cfg.Sampling.Refresh Rate (Hz)"="Refresh Rate (Hz)") -> (w251:T63)
                n116 = case shown="\"started\"" w249 {
                  tunnel: ["Action: Sampling Refresh Rate\nAction: Command" w257] -> w247
                  frame Default {
                  }
                  frame "started" {
                    n117 = Format Into String(format string="Action: State >> %s\nAction: Command\nAction: Sampling Refresh Rate\nAction: Command\nAction: State >> %s\nAction: Command", Set_State-enum."stop" ("State"), Set_State-enum."start" ("State")) -> (resulting string=w257:string)  [unwired: 2 in, 1 out]
                  }
                }
                n118 = call <vilib>:"Add State(s) to Queue__jki_lib_state_machine.vi"("State(s) in Front (\"\")"=w247, "State(s) in (\"\")"=w254) -> ("States Out"=w253:string)  [unwired: 13 in]
              }
              event "Decimation (pre DSP)": Value Change {
                # "Decimation Value Change Event (Button Pressed)\n()"
                n119 = event-data() -> ()  [unwired: 1 in, 6 out]
                n120 = Unbundle By Name(w260) -> ("DAQ state"=w262:T22)
                n121 = Bundle By Name(cluster=w260, "UI Config.DAQ.cfg.Sampling.Decimation.PreDSP"="Decimation (pre DSP)") -> (w264:T63)
                n122 = case shown="Default" w262 {
                  tunnel: ["Action: Sampling Decimation Pre DSP\nAction: Command" w270] -> w261
                  frame Default {
                  }
                  frame "started" {
                    n123 = Format Into String(format string="Action: State >> %s\nAction: Command\nAction: Sampling Decimation Pre DSP\nAction: Command\nAction: State >> %s\nAction: Command", Set_State-enum."stop" ("State"), Set_State-enum."start" ("State")) -> (resulting string=w270:string)  [unwired: 2 in, 1 out]
                  }
                }
                n124 = call <vilib>:"Add State(s) to Queue__jki_lib_state_machine.vi"("State(s) in Front (\"\")"=w261, "State(s) in (\"\")"=w267) -> ("States Out"=w266:string)  [unwired: 13 in]
              }
              event "Decimation (post DSP)": Value Change {
                # "hide from user for now (8/12/2022)"
                # "Decimation Value Change Event (Button Pressed)\n()"
                n125 = event-data() -> ()  [unwired: 1 in, 6 out]
                n126 = Unbundle By Name(w273) -> ("DAQ state"=w275:T22)
                n127 = Bundle By Name(cluster=w273, "UI Config.DAQ.cfg.Sampling.Decimation.PostDSP"="Decimation (post DSP)") -> (w277:T63)
                n128 = case shown="\"started\"" w275 {
                  tunnel: ["Action: Sampling Decimation Post DSP\nAction: Command" w283] -> w274
                  frame Default {
                  }
                  frame "started" {
                    n129 = Format Into String(format string="Action: State >> %s\nAction: Command\nAction: Sampling Decimation Post DSP\nAction: Command\nAction: State >> %s\nAction: Command", Set_State-enum."stop" ("State"), Set_State-enum."start" ("State")) -> (resulting string=w283:string)  [unwired: 2 in, 1 out]
                  }
                }
                n130 = call <vilib>:"Add State(s) to Queue__jki_lib_state_machine.vi"("State(s) in Front (\"\")"=w274, "State(s) in (\"\")"=w280) -> ("States Out"=w279:string)  [unwired: 13 in]
              }
              event Value Change {
                # "AI Channels Value Change Event (Button Pressed)\n()"
                n131 = event-data() -> ()  [unwired: 1 in, 6 out]
                n132 = Bundle By Name(cluster=w287, "UI Config.Channels.Cfg_AI"="AI Channels") -> (w288:T63)
                n133 = call <vilib>:"Add State(s) to Queue__jki_lib_state_machine.vi"("State(s) in Front (\"\")"="Action: AI Channels\nAction: Command", "State(s) in (\"\")"=w292) -> ("States Out"=w291:string)  [unwired: 13 in]
              }
              event Value Change {
                # "AO Channels Value Change Event (Button Pressed)\n()"
                n134 = event-data() -> ()  [unwired: 1 in, 6 out]
                n135 = Bundle By Name(cluster=w294, "UI Config.Channels.Cfg_AO"="AO Channels") -> (w295:T63)
                n136 = call <vilib>:"Add State(s) to Queue__jki_lib_state_machine.vi"("State(s) in Front (\"\")"="Action: AO Channels\nAction: Command", "State(s) in (\"\")"=w299) -> ("States Out"=w298:string)  [unwired: 13 in]
              }
              event Value Change {
                # "REF Channels Value Change Event (Button Pressed)\n()"
                n137 = event-data() -> ()  [unwired: 1 in, 6 out]
                n138 = Bundle By Name(cluster=w301, "UI Config.Channels.Cfg_REF"="REF Channels") -> (w302:T63)
                n139 = call <vilib>:"Add State(s) to Queue__jki_lib_state_machine.vi"("State(s) in Front (\"\")"="Action: REF Channels\nAction: Command", "State(s) in (\"\")"=w306) -> ("States Out"=w305:string)  [unwired: 13 in]
              }
              event Value Change {
                # "DAQ Config Value Change Event (Button Pressed)\n()"
                n140 = event-data() -> ()  [unwired: 1 in, 6 out]
                n141 = Bundle By Name(cluster=w308, "UI Config.DAQ.Simulation mode"="AI Simulation mode") -> (w309:T63)
                n142 = call <vilib>:"Add State(s) to Queue__jki_lib_state_machine.vi"("State(s) in Front (\"\")"="Action: AI Simulate Mode\nAction: Command", "State(s) in (\"\")"=w313) -> ("States Out"=w312:string)  [unwired: 13 in]
              }
              event Value Change {
                # "DAQ Config Value Change Event (Button Pressed)\n()"
                n143 = event-data() -> ()  [unwired: 1 in, 6 out]
                n144 = Bundle By Name(cluster=w315, "UI Config.Amplifers.Gain_AI"="Input Gain") -> (w316:T63)
                n145 = call <vilib>:"Add State(s) to Queue__jki_lib_state_machine.vi"("State(s) in Front (\"\")"="Action: Input Gain\nAction: Command", "State(s) in (\"\")"=w320) -> ("States Out"=w319:string)  [unwired: 13 in]
              }
              event Value Change {
                # "DAQ Config Value Change Event (Button Pressed)\n()"
                n146 = event-data() -> ()  [unwired: 1 in, 6 out]
                n147 = Bundle By Name(cluster=w322, "UI Config.Amplifers.Offset_AI"="Input Offsets") -> (w323:T63)
                n148 = call <vilib>:"Add State(s) to Queue__jki_lib_state_machine.vi"("State(s) in Front (\"\")"="Action: Offset\nAction: Command", "State(s) in (\"\")"=w327) -> ("States Out"=w326:string)  [unwired: 13 in]
              }
              event Value Change {
                # "DAQ Config Value Change Event (Button Pressed)\n()"
                n149 = event-data() -> ()  [unwired: 1 in, 6 out]
                n150 = Bundle By Name(cluster=w329, "UI Config.Amplifers.Gain_AO"="Output Gain") -> (w330:T63)
                n151 = call <vilib>:"Add State(s) to Queue__jki_lib_state_machine.vi"("State(s) in Front (\"\")"="Action: Output Gain\nAction: Command", "State(s) in (\"\")"=w334) -> ("States Out"=w333:string)  [unwired: 13 in]
              }
              event "Limit Amplitude (V)", "AO Amp Limit": Value Change {
                # "Limit Amplitudes Paramaters Change Event ()\n()"
                n152 = event-data() -> ()  [unwired: 1 in, 6 out]
                n153 = Bundle By Name(cluster=w337, "UI Config.Limit Amplitude.Limit?"="Limit Amplitude (V)", "UI Config.Limit Amplitude.Limit (V)"="AO Amp Limit") -> (w338:T63)
                n154 = call <vilib>:"Add State(s) to Queue__jki_lib_state_machine.vi"("State(s) in Front (\"\")"="Action: Limit Amplitude\nAction: Command", "State(s) in (\"\")"=w342) -> ("States Out"=w341:string)  [unwired: 13 in]
              }
              event "Limit DC (V)", "AO DC Limit": Value Change {
                # "Limit Amplitudes Paramaters Change Event ()\n()"
                n155 = event-data() -> ()  [unwired: 1 in, 6 out]
                n156 = Bundle By Name(cluster=w345, "UI Config.Limit Amplitude.Limit?"="Limit DC (V)", "UI Config.Limit Amplitude.Limit (V)"="AO DC Limit") -> (w346:T63)
                n157 = call <vilib>:"Add State(s) to Queue__jki_lib_state_machine.vi"("State(s) in Front (\"\")"="Action: Limit DC\nAction: Command", "State(s) in (\"\")"=w350) -> ("States Out"=w349:string)  [unwired: 13 in]
              }
              event "Link Frequencies", "AO freq link": Value Change {
                # "Link Frequencies Parameters Change Event ()\n()"
                n158 = event-data() -> ()  [unwired: 1 in, 6 out]
                n159 = Bundle By Name(cluster=w353, "UI Config.Link Frequencies.Link?"="Link Frequencies", "UI Config.Link Frequencies.Frequency (Hz)"="AO freq link") -> (w354:T63)
                n160 = call <vilib>:"Add State(s) to Queue__jki_lib_state_machine.vi"("State(s) in Front (\"\")"="Action: Link Frequencies\nAction: Command", "State(s) in (\"\")"=w358) -> ("States Out"=w357:string)  [unwired: 13 in]
              }
              event "Reset Phase": Value Change {
                # "Reset Phase Value Change Event (Button Pressed)\n()"
                n161 = event-data() -> ()  [unwired: 1 in, 6 out]
                n162 = local write "Reset Phase"(FALSE ("Help")) -> ()
                n163 = call <vilib>:"Add State(s) to Queue__jki_lib_state_machine.vi"("State(s) in Front (\"\")"="Action: Zero Phase\nAction: Command", "State(s) in (\"\")"=w364) -> ("States Out"=w363:string)  [unwired: 13 in]
              }
              event "Line", "Lowpass", "LP f (Hz)": Value Change {
                # "Prefilter Paramters Change Event ()\n()"
                n164 = event-data() -> ()  [unwired: 1 in, 6 out]
                n165 = Bundle By Name(cluster=w368, "UI Config.PreFilter.60 Hz"="Line", "UI Config.PreFilter.Low Pass"="Lowpass", "UI Config.PreFilter.Low Pass Cutoff (Hz)"="LP f (Hz)") -> (w369:T63)
                n166 = call <vilib>:"Add State(s) to Queue__jki_lib_state_machine.vi"("State(s) in Front (\"\")"="Action: PreFilter\nAction: Command", "State(s) in (\"\")"=w373) -> ("States Out"=w372:string)  [unwired: 13 in]
              }
              event "Sweep Time (s)", "Return to Start?", "Initial Wait (s)", "Sweep Pattern": Value Change {
                # "Sweep Parameters (Time, Wait, Return, Channels) Change Event ()\n()"
                n167 = event-data() -> ()  [unwired: 1 in, 6 out]
                n168 = Unbundle By Name(w376) -> ("UI Config.Sweep"=w381:T54)
                n169 = for {
                  tunnel: [w394] -> w374 mode=indexing
                  tunnel: "Sweep Pattern" -> [w393] mode=indexing
                  n170 = Unbundle By Name(w393) -> ("Channel"=w392:u16, "Sweep Pattern"=w391:dbl[])
                  n171 = Bundle By Name(cluster=T32 {"Channel"=1, "Table"=[]} ("setSweep_Table"), "Channel"=w392, "Table"=w391) -> (w394:T32)
                }
                n172 = Bundle By Name(cluster=w381, "Sweep Time (s)"="Sweep Time (s)", "Initial Wait (s)"="Initial Wait (s)", "Return to Start"="Return to Start?", "Channels"="Sweep Channels") -> (w375:T54)
                n173 = call "Replace Sweep Waveforms.vi"("Channels New"=w374, "Sweep in"=w375) -> ("Sweep out"=w382:T54)  [unwired: 9 in]
                n174 = Bundle By Name(cluster=w376, "UI Config.Sweep"=w382) -> (w385:T63)
                n175 = call <vilib>:"Add State(s) to Queue__jki_lib_state_machine.vi"("State(s) in Front (\"\")"="Action: Sweep\nAction: Command", "State(s) in (\"\")"=w389) -> ("States Out"=w388:string)  [unwired: 13 in]
                "Sweep Timer (s)" <- 0.0 ("Sweep Timer (s)")
              }
              event "Remove Offset": Value Change {
                # "Remove Offset Value Change Event (Button Pressed)\n()"
                n176 = event-data() -> ()  [unwired: 1 in, 6 out]
                n177 = local write "Remove Offset"(FALSE ("Help")) -> ()
                n178 = Format Into String(format string="Action: Offset Mode >> %s\nAction: Command", Offset_Mode--Enum."Remove" ("Offset Mode")) -> (resulting string=w396:string)  [unwired: 2 in, 1 out]
                n179 = call <vilib>:"Add State(s) to Queue__jki_lib_state_machine.vi"("State(s) in Front (\"\")"=w396, "State(s) in (\"\")"=w402) -> ("States Out"=w401:string)  [unwired: 13 in]
              }
              event "Measure Offset": Value Change {
                # "Measure Offset Value Change Event (Button Pressed)\n()"
                n180 = event-data() -> ()  [unwired: 1 in, 6 out]
                n181 = local write "Measure Offset"(FALSE ("Help")) -> ()
                n182 = Format Into String(format string="Action: Offset Mode >> %s\nAction: Command", Offset_Mode--Enum."Measure" ("Offset Mode")) -> (resulting string=w404:string)  [unwired: 2 in, 1 out]
                n183 = call <vilib>:"Add State(s) to Queue__jki_lib_state_machine.vi"("State(s) in Front (\"\")"=w404, "State(s) in (\"\")"=w410) -> ("States Out"=w409:string)  [unwired: 13 in]
              }
              event "Get Calibration": Value Change {
                # "Get Calibration Value Change Event (Button Pressed)\n()"
                n184 = event-data() -> ()  [unwired: 1 in, 6 out]
                n185 = local write "Get Calibration"(FALSE ("Help")) -> ()
                n186 = Format Into String(format string="Action: Calibrate >> %s\nAction: Command", PrivateEvents--DAQ.setCalibration."Check" ("setCalibration")) -> (resulting string=w412:string)  [unwired: 2 in, 1 out]
                n187 = call <vilib>:"Add State(s) to Queue__jki_lib_state_machine.vi"("State(s) in Front (\"\")"=w412, "State(s) in (\"\")"=w418) -> ("States Out"=w417:string)  [unwired: 13 in]
              }
              event "Self Calibrate": Value Change {
                # "Get Calibration Value Change Event (Button Pressed)\n()"
                n188 = event-data() -> ()  [unwired: 1 in, 6 out]
                n189 = local write "Self Calibrate"(FALSE ("Help")) -> ()
                n190 = Format Into String(format string="Action: Calibrate >> %s\nAction: Command", PrivateEvents--DAQ.setCalibration."Calibrate" ("setCalibration")) -> (resulting string=w419:string)  [unwired: 2 in, 1 out]
                n191 = call <vilib>:"Add State(s) to Queue__jki_lib_state_machine.vi"("State(s) in Front (\"\")"=w419, "State(s) in (\"\")"=w426) -> ("States Out"=w425:string)  [unwired: 13 in]
              }
              event "Show UI": Value Change {
                # "Get Calibration Value Change Event (Button Pressed)\n()"
                n192 = event-data() -> ()  [unwired: 1 in, 6 out]
                n193 = Format Into String(format string="Action: showUI >> %s\nAction: Command", "Show UI") -> (resulting string=w427:string)  [unwired: 2 in, 1 out]
                n194 = call <vilib>:"Add State(s) to Queue__jki_lib_state_machine.vi"("State(s) in Front (\"\")"=w427, "State(s) in (\"\")"=w433) -> ("States Out"=w432:string)  [unwired: 13 in]
              }
              event "Logging": Value Change {
                # "Get Calibration Value Change Event (Button Pressed)\n()"
                n195 = event-data() -> ("NewVal"=w434:bool)  [unwired: 1 in, 5 out]
                n196 = Format Into String(format string="Action: Logging >> %s\nAction: Command", w434) -> (resulting string=w435:string)  [unwired: 2 in, 1 out]
                n197 = call <vilib>:"Add State(s) to Queue__jki_lib_state_machine.vi"("State(s) in Front (\"\")"=w435, "State(s) in (\"\")"=w440) -> ("States Out"=w439:string)  [unwired: 13 in]
              }
              event "....................Graph and UI....................": Value Change {
                # "Do not put any code in this frame.\n(it is a separator no-op)"
                n198 = event-data() -> ()  [unwired: 1 in, 6 out]
                n199 = call <vilib>:"Add State(s) to Queue__jki_lib_state_machine.vi"("State(s) in (\"\")"=w444) -> ("States Out"=w443:string)  [unwired: 14 in]
              }
              event Value Change {
                # "Display Value Change Event (Button Pressed)\n()"
                n200 = event-data() -> ()  [unwired: 1 in, 6 out]
                n201 = call <vilib>:"Add State(s) to Queue__jki_lib_state_machine.vi"("State(s) in Front (\"\")"="UI: Update Lockin Graph Labels", "State(s) in (\"\")"=w449) -> ("States Out"=w448:string)  [unwired: 13 in]
              }
              event "AI Graph": Plot Attribute Change {
                # "Display Value Change Event (Button Pressed)\n()"
                n202 = event-data() -> ()  [unwired: 1 in, 8 out]
                n203 = call <vilib>:"Add State(s) to Queue__jki_lib_state_machine.vi"("State(s) in Front (\"\")"="UI: Sync AI Plot Visibility", "State(s) in (\"\")"=w454) -> ("States Out"=w453:string)  [unwired: 13 in]
              }
              event "AO Graph": Value Change {
                # "Display Value Change Event (Button Pressed)\n()"
                n204 = event-data() -> ()  [unwired: 1 in, 6 out]
                n205 = call <vilib>:"Add State(s) to Queue__jki_lib_state_machine.vi"("State(s) in Front (\"\")"="UI: Sync AO Plot Visibility", "State(s) in (\"\")"=w459) -> ("States Out"=w458:string)  [unwired: 13 in]
              }
              event "Lockin 1": Plot Attribute Change {
                # "Display Value Change Event (Button Pressed)\n()"
                n206 = event-data() -> ()  [unwired: 1 in, 8 out]
                n207 = call <vilib>:"Add State(s) to Queue__jki_lib_state_machine.vi"("State(s) in Front (\"\")"="UI: Sync Lockin Plot Visibility", "State(s) in (\"\")"=w464) -> ("States Out"=w463:string)  [unwired: 13 in]
              }
              event "Disable all AI Ref", "Enable only AI Ref1": Value Change {
                # "AI Disable or Enable Change Event (Button Pressed)\n()"
                n208 = event-data() -> ("CtlRef"=w465:refnum<vi>)  [unwired: 1 in, 5 out]
                n209 = control-ref of="Disable all AI Ref"() -> (w467:refnum<vi>)
                n210 = Equal?(x=w465, y=w467) -> (x = y?=w466:bool)
                n211 = flat-sequence {
                  tunnel: w466 -> [_]
                  frame #0 {
                    n212 = local write "Enable only AI Ref1"(FALSE ("Disable all AI Ref")) -> ()
                    n213 = local write "Disable all AI Ref"(FALSE ("Disable all AI Ref")) -> ()
                  }
                }
                n214 = Select(t="Disable" ("Arguments (\"\")"), s=w466, f="ALL 1" ("Arguments (\"\")")) -> (s? t:f=w468:string)
                n215 = call <vilib>:"Build State String with Arguments__JKI_lib_State_Machine.vi"("Arguments (\"\")"=w468, "State"="UI: Update AI REF Channels") -> ("State with Arguments"=w473:string)  [unwired: 4 in]
                n216 = call <vilib>:"Add State(s) to Queue__jki_lib_state_machine.vi"("State(s) in Front (\"\")"=w473, "State(s) at Back (\"\")"="Action: AI Channels\nAction: Command") -> ("States Out"=w471:string)  [unwired: 13 in]
                n217 = call <vilib>:"Add State(s) to Queue__jki_lib_state_machine.vi"("State(s) in Front (\"\")"=w471, "State(s) in (\"\")"=w478) -> ("States Out"=w477:string)  [unwired: 13 in]
              }
              event "AI Graph All", "AI Graph None": Value Change {
                # "AI Graph All/None Value Change Event (Button Pressed)\n()"
                n218 = event-data() -> ("CtlRef"=w486:refnum<vi>)  [unwired: 1 in, 5 out]
                n219 = control-ref of="AI Graph All"() -> (w485:refnum<vi>)
                n220 = Equal?(x=w486, y=w485) -> (x = y?=w481:bool)
                n221 = Select(t="ALL" ("Arguments (\"\")"), s=w481, f="NONE" ("Arguments (\"\")")) -> (s? t:f=w482:string)
                n222 = call <vilib>:"Build State String with Arguments__JKI_lib_State_Machine.vi"("Arguments (\"\")"=w482, "State"="UI: AI Graphs Plot Visibility") -> ("State with Arguments"=w487:string)  [unwired: 4 in]
                n223 = call <vilib>:"Add State(s) to Queue__jki_lib_state_machine.vi"("State(s) in Front (\"\")"=w487, "State(s) in (\"\")"=w492) -> ("States Out"=w491:string)  [unwired: 13 in]
              }
              event "AO Graph All", "AO Graph None": Value Change {
                # "AO Graph All Value Change Event (Button Pressed)\n()"
                n224 = event-data() -> ("CtlRef"=w498:refnum<vi>)  [unwired: 1 in, 5 out]
                n225 = control-ref of="AO Graph All"() -> (w497:refnum<vi>)
                n226 = Equal?(x=w498, y=w497) -> (x = y?=w496:bool)
                n227 = Select(t="ALL" ("Arguments (\"\")"), s=w496, f="NONE" ("Arguments (\"\")")) -> (s? t:f=w493:string)
                n228 = call <vilib>:"Build State String with Arguments__JKI_lib_State_Machine.vi"("Arguments (\"\")"=w493, "State"="UI: AO Graphs Plot Visibility") -> ("State with Arguments"=w499:string)  [unwired: 4 in]
                n229 = call <vilib>:"Add State(s) to Queue__jki_lib_state_machine.vi"("State(s) in Front (\"\")"=w499, "State(s) in (\"\")"=w504) -> ("States Out"=w503:string)  [unwired: 13 in]
              }
              event "Lockin Graph All", "Lockin Graph None": Value Change {
                # "Lockin Graph All Value Change Event (Button Pressed)\n()"
                n230 = event-data() -> ("CtlRef"=w510:refnum<vi>)  [unwired: 1 in, 5 out]
                n231 = control-ref of="Lockin Graph All"() -> (w509:refnum<vi>)
                n232 = Equal?(x=w510, y=w509) -> (x = y?=w506:bool)
                n233 = Select(t="ALL" ("Arguments (\"\")"), s=w506, f="NONE" ("Arguments (\"\")")) -> (s? t:f=w505:string)
                n234 = call <vilib>:"Build State String with Arguments__JKI_lib_State_Machine.vi"("Arguments (\"\")"=w505, "State"="UI: Lockin Graphs Plot Visibility") -> ("State with Arguments"=w511:string)  [unwired: 4 in]
                n235 = call <vilib>:"Add State(s) to Queue__jki_lib_state_machine.vi"("State(s) in Front (\"\")"=w511, "State(s) in (\"\")"=w516) -> ("States Out"=w515:string)  [unwired: 13 in]
              }
              event "X/R Range", "Y/Theta Range", "XY Range": Value Change {
                # "X/R Range, Y/Theta Range, XY Range Value Change Event\n(this executes UI: Update Lockin Graph Range)"
                n236 = event-data() -> ()  [unwired: 1 in, 6 out]
                n237 = call <vilib>:"Add State(s) to Queue__jki_lib_state_machine.vi"("State(s) in Front (\"\")"="UI: Update Lockin Graph Range", "State(s) in (\"\")"=w521) -> ("States Out"=w520:string)  [unwired: 13 in]
              }
              event "Y Axis (Output)", "X Axis": Value Change {
                # "Y Axis (Output), X Axis Value Change Event\n(this executes UI: Update Waveform Graph Labels)"
                n238 = event-data() -> ()  [unwired: 1 in, 6 out]
                n239 = call <vilib>:"Add State(s) to Queue__jki_lib_state_machine.vi"("State(s) in Front (\"\")"="UI: Update Waveform Graph Labels", "State(s) in (\"\")"=w526) -> ("States Out"=w525:string)  [unwired: 13 in]
              }
              event "....................Dynamic Events....................": Value Change {
                # "Do not put any code in this frame.\n(it is a separator no-op)"
                n240 = event-data() -> ()  [unwired: 1 in, 6 out]
                n241 = call <vilib>:"Add State(s) to Queue__jki_lib_state_machine.vi"("State(s) in (\"\")"=w530) -> ("States Out"=w529:string)  [unwired: 14 in]
              }
              event User Event {
                # "<SMO Protected Events.StopProcesses>: User Event"
                n242 = event-data() -> ()  [unwired: 1 in, 5 out]
                n243 = call <vilib>:"Add State(s) to Queue__jki_lib_state_machine.vi"("State(s) in Front (\"\")"="Macro: Exit", "State(s) in (\"\")"=w535) -> ("States Out"=w534:string)  [unwired: 13 in]
              }
              event User Event {
                # "<SMO Protected Events.AbortProcesses>: User Event"
                # "On Abort, no nice macro exit, but exit right away"
                n244 = event-data() -> ()  [unwired: 1 in, 5 out]
                n245 = call <vilib>:"Add State(s) to Queue__jki_lib_state_machine.vi"("State(s) in Front (\"\")"="Exit", "State(s) in (\"\")"=w540) -> ("States Out"=w539:string)  [unwired: 13 in]
              }
              event User Event {
                # "<SMO.UI Public Events.UI Hidden>: User Event"
                n246 = event-data() -> ()  [unwired: 1 in, 5 out]
                n247 = call <vilib>:"Add State(s) to Queue__jki_lib_state_machine.vi"("State(s) in (\"\")"=w544) -> ("States Out"=w543:string)  [unwired: 14 in]
              }
              event User Event {
                # "<DAQ SMO Public Events.Error>: User Event"
                n248 = event-data() -> ()  [unwired: 1 in, 7 out]
                n249 = call <vilib>:"Add State(s) to Queue__jki_lib_state_machine.vi"("State(s) in (\"\")"=w548) -> ("States Out"=w547:string)  [unwired: 14 in]
              }
              event User Event {
                # "<DAQ SMO Public Events.State>: User Event"
                n250 = event-data() -> ("SMO State"=w549:T64)  [unwired: 1 in, 4 out]
                n251 = case shown="\"Started\"" w549 {
                  tunnel: ["UI: Enable Buttons" ("State Queue") "//DONE: Stop\n//DONE: Start" ("State Queue")] -> w550
                  frame "Started" {
                  }
                  frame Default {
                  }
                }
                n252 = call <vilib>:"Add State(s) to Queue__jki_lib_state_machine.vi"("State(s) in Front (\"\")"=w550, "State(s) in (\"\")"=w554) -> ("States Out"=w553:string)  [unwired: 13 in]
              }
              event User Event {
                # "<DAQ Public Events.getDAQState>: User Event"
                n253 = event-data() -> ("state"=w559:T22)  [unwired: 1 in, 4 out]
                "state" <- w559
                n254 = Unbundle By Name(w570) -> ("References.Booleans.Start"=w568:refnum<vi>, "References.Booleans.Pause"=w567:refnum<vi>, "References.Booleans.Reset"=w569:refnum<vi>, "References.Booleans.Trigger"=w566:refnum<vi>, "References.Booleans.Start Sweep"=w565:refnum<vi>, "References.Booleans.Stop Sweep"=w561:refnum<vi>)
                n255 = Get Date/Time In Seconds() -> (seconds since 1Jan1904=w558:timestamp)
                n256 = Format Into String(w559) -> (resulting string=→"Instrument.DAQ SMO State":string)  [unwired: 3 in, 1 out]
                n257 = To Double Precision Float(number=w558) -> (double precision float=→"current time":dbl)
                n258 = Bundle By Name(cluster=w570, "DAQ state"=w559) -> (w573:T63)
                n259 = case shown="\"started\"" w559 {
                  tunnel: ["Idle" ("Status") "Started" ("Status") "Stopped" ("Status") "Running" ("Status") "Sweeping" ("Status")] -> w564
                  tunnel: w569 -> [w583 w590 w594 w598 _]
                  tunnel: w568 -> [w584 w587 w595 w599 _]
                  tunnel: w567 -> [_ _ _ _ _]
                  tunnel: w566 -> [w582 _ w593 _ _]
                  tunnel: w565 -> [_ w589 _ _ _]
                  tunnel: [w581 w591 w596 w601 _] -> w563
                  tunnel: [_ w586 _ w600 _] -> w562
                  tunnel: w561 -> [_ w588 _ _ _]
                  frame "idle", Default {
                    n260 = Build Array(w584, w583, w582) -> (w581:refnum<vi>[])
                  }
                  frame "started" {
                    n261 = Build Array(w587) -> (w586:refnum<vi>[])
                    n262 = Build Array(w590, w589, w588) -> (w591:refnum<vi>[])
                  }
                  frame "stopped" {
                    n263 = Build Array(w595, w594, w593) -> (w596:refnum<vi>[])
                  }
                  frame "created" {
                    n264 = Build Array(w599) -> (w600:refnum<vi>[])
                    n265 = Build Array(w598) -> (w601:refnum<vi>[])
                  }
                  frame "sweeping" {
                    n266 = call <userlib>:"MGI Milliseconds Since Last Reset.vi"("Reset (F)"=TRUE) -> ()  [unwired: 5 in, 2 out]
                  }
                }
                n267 = call <vilib>:"Build State String with Arguments__JKI_lib_State_Machine.vi"("Arguments (\"\")"=w564, "State"="UI: Update Status") -> ("State with Arguments"=w571:string)  [unwired: 4 in]
                n268 = for {
                  tunnel: w562 -> [w577] mode=indexing
                  n269 = property class="Bool (strict)"(reference=w577, "Value"=TRUE) -> ()  [unwired: 1 in, 2 out]
                }
                n270 = for {
                  tunnel: w563 -> [w579] mode=indexing
                  n271 = property class="Bool (strict)"(reference=w579, "Value"=FALSE) -> ()  [unwired: 1 in, 2 out]
                }
                n272 = call <vilib>:"Add State(s) to Queue__jki_lib_state_machine.vi"("State(s) in Front (\"\")"=w571, "State(s) in (\"\")"=w576) -> ("States Out"=w575:string)  [unwired: 13 in]
              }
              event User Event {
                # "<DAQ Public Events.getWaveforms>: User Event"
                n273 = event-data() -> ("AO_wfm"=w609:waveform(dbl)[], "AI_wfm"=w608:waveform(dbl)[], "Ref_X_wfm"=w607:waveform(dbl)[], "Ref_Y_wfm"=w606:waveform(dbl)[])  [unwired: 1 in, 4 out]
                n274 = Bundle By Name(cluster=w625, "getAll.Waveforms.AO_wfm"=w609, "getAll.Waveforms.AI_wfm"=w608, "getAll.Waveforms.Ref_X_wfm"=w607, "getAll.Waveforms.Ref_Y_wfm"=w606) -> (w626:T63)
                n275 = call <userlib>:"MGI Milliseconds Since Last Call.vi"() -> ("ms"=w605:u32)  [unwired: 6 in, 1 out]
                "WFM Refresh time (ms)" <- w605
                n276 = Index Array(array=w608) -> (element=w624:waveform(dbl))  [unwired: 1 in]
                n277 = call-poly <vilib>:"Waveform Duration.vi"("error in (no error)"=w615, "waveform in"=w624) -> ("error out"=w616:errorcluster, "duration"=w623:dbl)  [unwired: 7 in, 1 out]
                n278 = Multiply(x=w623, y=1000.0) -> (x*y=w618:dbl)
                n279 = Multiply(x=w618, y=2.0) -> (x*y=w617:dbl)
                n280 = Less?(x=w605, y=w617) -> (x < y?=w611:bool)
                n281 = Select(t=u32 6618880, s=w611, f=u32 16711680) -> (s? t:f=w614:u32)
                n282 = Select(t="Good", s=w611, f="#s/Fs: too small!") -> (s? t:f=→"Sampling Status":string)
                n283 = property on="Sampling Status" class="Str"("Text.BGColor"=w614) -> ()  [unwired: 2 in, 2 out]
                n284 = call <vilib>:"Add State(s) to Queue__jki_lib_state_machine.vi"("State(s) in Front (\"\")"="Macro: Update Graphs", "State(s) in (\"\")"=w629) -> ("States Out"=w628:string)  [unwired: 13 in]
              }
              event User Event {
                # "<DAQ Public Events.getResults>: User Event"
                n285 = event-data() -> ("Results"=w631:T57)  [unwired: 1 in, 4 out]
                n286 = Bundle By Name(cluster=w632, "getAll.Results"=w631) -> (w633:T63)
                n287 = call <vilib>:"Add State(s) to Queue__jki_lib_state_machine.vi"("State(s) in Front (\"\")"="", "State(s) in (\"\")"=w636) -> ("States Out"=w635:string)  [unwired: 13 in]
              }
              event User Event {
                # "<DAQ Public Events.getCalibration>: User Event"
                n288 = event-data() -> ("Calibration"=w637:T23)  [unwired: 1 in, 4 out]
                "Cal Info" <- w637
                n289 = Bundle By Name(cluster=w638, "UI Config.DAQ.Calibration"=w637) -> (w639:T63)
                n290 = call <vilib>:"Add State(s) to Queue__jki_lib_state_machine.vi"("State(s) in Front (\"\")"="", "State(s) in (\"\")"=w643) -> ("States Out"=w642:string)  [unwired: 13 in]
              }
              event User Event {
                # "<DAQ Public Events.getAOChannels>: User Event"
                n291 = event-data() -> ("Channels: AO"=w644:T4)  [unwired: 1 in, 4 out]
                n292 = Bundle By Name(cluster=w645, "UI Config.Channels.Cfg_AO"=w644) -> (w646:T63)
                n293 = local write "AO Channels"(w644) -> ()
                n294 = call <vilib>:"Add State(s) to Queue__jki_lib_state_machine.vi"("State(s) in Front (\"\")"="", "State(s) in (\"\")"=w650) -> ("States Out"=w649:string)  [unwired: 13 in]
              }
              event User Event {
                # "<DAQ Public Events.getAIChannels>: User Event"
                n295 = event-data() -> ("Channels.AI"=w651:T2)  [unwired: 1 in, 4 out]
                n296 = Bundle By Name(cluster=w652, "UI Config.Channels.Cfg_AI"=w651) -> (w653:T63)
                n297 = local write "AI Channels"(w651) -> ()
                n298 = call <vilib>:"Add State(s) to Queue__jki_lib_state_machine.vi"("State(s) in Front (\"\")"="", "State(s) in (\"\")"=w657) -> ("States Out"=w656:string)  [unwired: 13 in]
              }
              event User Event {
                # "<DAQ Public Events.getREFChannels>: User Event"
                n299 = event-data() -> ("Channels: REF"=w658:T7)  [unwired: 1 in, 4 out]
                n300 = Bundle By Name(cluster=w659, "UI Config.Channels.Cfg_REF"=w658) -> (w660:T63)
                n301 = local write "REF Channels"(w658) -> ()
                n302 = call <vilib>:"Add State(s) to Queue__jki_lib_state_machine.vi"("State(s) in Front (\"\")"="UI: Update Channel Ring\nUI: Update AI REF Channel Ring\nUI: Remove Unused References", "State(s) in (\"\")"=w664) -> ("States Out"=w663:string)  [unwired: 13 in]
              }
              event User Event {
                # "<DAQ Public Events.getSweepChannels>: User Event"
                n303 = event-data() -> ("Channels.Sweep"=w665:T54)  [unwired: 1 in, 4 out]
                n304 = Bundle By Name(cluster=w666, "UI Config.Sweep"=w665) -> (w667:T63)
                n305 = call <vilib>:"Add State(s) to Queue__jki_lib_state_machine.vi"("State(s) in Front (\"\")"="UI: Update Sweep Config", "State(s) in (\"\")"=w671) -> ("States Out"=w670:string)  [unwired: 13 in]
              }
              event User Event {
                # "<DAQ Public Events.getSweepWaveforms>: User Event"
                n306 = event-data() -> ("AO_wfm"=w684:waveform(dbl)[], "AI_wfm"=w683:waveform(dbl)[], "X_wfm"=w682:waveform(dbl)[], "Y_wfm"=w681:waveform(dbl)[])  [unwired: 1 in, 4 out]
                n307 = Bundle By Name(cluster=w680, "getAll.Waveforms.AO_wfm"=w684, "getAll.Waveforms.AI_wfm"=w683, "getAll.Waveforms.X_wfm"=w682, "getAll.Waveforms.Y_wfm"=w681) -> (w685:T63)
                n308 = Unbundle By Name(w680) -> ("DAQ state"=w674:T22)
                "getAll.DAQ state" <- w674
                n309 = Get Date/Time In Seconds() -> (seconds since 1Jan1904=w673:timestamp)
                n310 = To Double Precision Float(number=w673) -> (double precision float=→"current time 2":dbl)
                n311 = Equal?(x=Get_State-enum."idle" ("getAll.DAQ state"), y=w674) -> (x = y?=w677:bool)
                n312 = Select(t="Macro: Initialize Graphs", s=w677, f="UI: Update Sweep Graphs") -> (s? t:f=w675:string)
                n313 = call <vilib>:"Add State(s) to Queue__jki_lib_state_machine.vi"("State(s) in Front (\"\")"=w675, "State(s) in (\"\")"=w688) -> ("States Out"=w687:string)  [unwired: 13 in]
              }
              event User Event {
                # "<DAQ Public Events.getDAQconfig>: User Event"
                n314 = event-data() -> ("New Ch []"=w689:T11)  [unwired: 1 in]
                n315 = Bundle By Name(cluster=w690, "UI Config.DAQ.Configuration"=w689) -> (w691:T63)
                n316 = local write "DAQ Config"(w689) -> ()
                n317 = call <vilib>:"Add State(s) to Queue__jki_lib_state_machine.vi"("State(s) in Front (\"\")"="UI: Update AI Waveform Graphs Legends\nUI: Update AI Waveform Graphs Colors\nUI: Update AO Waveform Graphs Legends\nUI: Update AO Waveform Graphs Colors", "State(s) in (\"\")"=w695) -> ("States Out"=w694:string)  [unwired: 13 in]
              }
              event User Event {
                # "<DAQ Public Events.getSampling>: User Event"
                n318 = event-data() -> ("Sampling"=w698:T47)  [unwired: 1 in]
                n319 = Unbundle By Name(w698) -> ("Sampling.Fs"=w697:dbl, "Sampling.#s"=w696:i32)
                n320 = Bundle By Name(cluster=w699, "UI Config.DAQ.cfg.Sampling"=w698) -> (w700:T63)
                n321 = local write "Fs (S/s)"(w697) -> ()
                n322 = local write "#s (S)"(w696) -> ()
                n323 = call <vilib>:"Add State(s) to Queue__jki_lib_state_machine.vi"("State(s) in Front (\"\")"="", "State(s) in (\"\")"=w704) -> ("States Out"=w703:string)  [unwired: 13 in]
              }
              event User Event {
                # "<DAQ Public Events.getInputGain>: User Event"
                n324 = event-data() -> ("Input Gain"=w705:T9)  [unwired: 1 in, 4 out]
                n325 = Bundle By Name(cluster=w706, "UI Config.Amplifers.Gain_AI"=w705) -> (w707:T63)
                n326 = local write "Input Gain"(w705) -> ()
                n327 = call <vilib>:"Add State(s) to Queue__jki_lib_state_machine.vi"("State(s) in Front (\"\")"="", "State(s) in (\"\")"=w711) -> ("States Out"=w710:string)  [unwired: 13 in]
              }
              event User Event {
                # "<DAQ Public Events.getOutputGain>: User Event"
                n328 = event-data() -> ("Output Gain"=w712:T9)  [unwired: 1 in, 4 out]
                n329 = Bundle By Name(cluster=w713, "UI Config.Amplifers.Gain_AO"=w712) -> (w714:T63)
                n330 = local write "Output Gain"(w712) -> ()
                n331 = call <vilib>:"Add State(s) to Queue__jki_lib_state_machine.vi"("State(s) in Front (\"\")"="", "State(s) in (\"\")"=w718) -> ("States Out"=w717:string)  [unwired: 13 in]
              }
              event User Event {
                # "<DAQ Public Events.getInputOffset>: User Event"
                n332 = event-data() -> ("Input Offset"=w719:T9)  [unwired: 1 in, 4 out]
                n333 = Bundle By Name(cluster=w720, "UI Config.Amplifers.Offset_AI"=w719) -> (w721:T63)
                n334 = local write "Input Offsets"(w719) -> ()
                n335 = call <vilib>:"Add State(s) to Queue__jki_lib_state_machine.vi"("State(s) in Front (\"\")"="", "State(s) in (\"\")"=w725) -> ("States Out"=w724:string)  [unwired: 13 in]
              }
            }
          }
          frame "---------- Core ----------" {
            # "Do not put any code in this frame.\n(it is a separator no-op)"
            n336 = call <vilib>:"Add State(s) to Queue__jki_lib_state_machine.vi"("State(s) in (\"\")"=w730) -> ("States Out"=w729:string)  [unwired: 14 in]
          }
          frame Default {
            w741 = 42 items=["No error", "Argument error", "Memory is full", "Out of zone", "End of file", "File already open", "Generic file I/O error", "File not found", "File permission error", "Disk is full", "Duplicate path", "Too many files open", "System feature not enabled", "Resource file not found", "Cannot add resource", "Resource not found", "Image not found", "Image memory error", "Pen does not exist", "Config type invalid", "Config token not found", "Config parse error", "Config memory error", "Bad external code format", "Bad external code offset", "External code not present", "Null window", "Destroy window error", "Null menu", "Print aborted", "Bad print record", "Print driver error", "Windows error during printing", "Memory error during printing", "Print dialog error", "Generic print error", "Invalid device refnum", "Device not found", "Device parameter error", "Device unit error", "Cannot open device", "Device call aborted", "Generic error", "Cancelled by user", "Object ID too low", "Object ID too high", "Object not in heap", "Unknown heap", "Unknown object (invalid DefProc)", "Unknown object (DefProc not in table)", "Message out of range", "Invalid (null) method", "Unknown message", "Manager call not supported", "Bad address", "Network operation in progress", "Network operation timed out", "Connection is busy", "Network attribute not supported", "Network error", "Address in use", "System out of memory", "Connection aborted", "Connection refused", "Not connected", "Already connected", "Connection closed", "Initialization error (interapplication manager)", "Bad occurrence", "Wait on unbound occurrence handler", "Occurrence queue overflow", "Datalog type conflict", "Unused", "Unrecognized type (interapplication manager)", "Memory corrupt", "Failed to make temporary DLL", "Old CIN version", "Drag socket not found", "Failed to load drop-object", "Failed to register OLE object", "Failed to release OLE object", "Format specifier type mismatch", "Unknown format specifier", "Too few format specifiers", "Too many format specifiers", "Scan failed", "Newer CIN version", "Error converting to variant", "Runtime menu error", "Password tampered", "Variant attribute not found", "Incompatible variant data type", "Event data is not available", "Event Store is not present", "Occurrence is not found", "Event Queue is not created", "Event info is not available", "Refnum passed is NULL", "Error retrieving Class GUID", "Error retrieving CoClass GUID", "Error retrieving TypeLib GUID.", "Bad built application magic bytes.", "Specific driver is different from the specific driver associated with the Logical Name.", "There is no session opened to the class driver.", "Max Error", "MAX - Error with config objects", "MAX - Error loading configuration", "MAX - Group not supported"]
            # "Current State"
            # "Do not delete, rename, or modify this frame.\n(this is used to capture unhandled states and typos)"
            # "Handle mistyped state name (developer tool)"
            n337 = Format Into String(format string="Software Exception: Unhandled State \"%s\"." ("message"), error in=w737, w732) -> (resulting string=w740:string, error out=w739:errorcluster)  [unwired: 1 in]
            n338 = call <vilib>:"Error Cluster From Error Code.vi"("show call chain? (False)"=TRUE, "error in (no error)"=w739, "error message (\"\")"=w740, "error code (0)"=w741) -> ("error out"=w738:errorcluster)  [unwired: 5 in]
            n339 = call <vilib>:"Add State(s) to Queue__jki_lib_state_machine.vi"("State(s) in (\"\")"=w736) -> ("States Out"=w735:string)  [unwired: 14 in]
          }
          frame "Initialize Core Data" {
            # "Do not delete, rename, or modify this frame.\n(this is used to determine panel behavior on exit)"
            # "originally closed?"
            # "exe?"
            # "If panel starts closed or is an EXE, then close it when we exit"
            n340 = property class="VI"() -> ("Front Panel.Open"=w751:bool)  [unwired: 2 in, 2 out]
            n341 = property class="App"() -> ("App.Kind"=w750:T35)  [unwired: 2 in, 2 out]
            n342 = control-ref of="Current VI Reference"() -> (w744:refnum<vi>)
            n343 = Not(x=w751) -> (.not. x?=w748:bool)
            n344 = Equal?(x=w750, y=T35."Run Time System" ("Application:Kind")) -> (x = y?=w747:bool)
            n345 = Or(x=w748, y=w747) -> (x .or. y?=w745:bool)
            n346 = Bundle By Name(cluster=w746, "Core.Current VI Reference"=w744, "Core.Close Panel on Exit?"=w745) -> (w753:T63)
            n347 = call <vilib>:"Add State(s) to Queue__jki_lib_state_machine.vi"("State(s) in (\"\")"=w755) -> ("States Out"=w754:string)  [unwired: 14 in]
          }
          frame "Error Handler" {
            w763 = errorcluster {"status"=FALSE, "code"=0, "source"=""}  # No error
            # "There was an error while handling the error.\nStop the process. This error can only occur if public events references are invalid or if the state machine object is destroyed."
            # "Overwrite this method to handle errors and pass to parent if not handled. Parent will fire a public event if the error is not handled up the chain of classes."
            # "Handle any errors here.\nYou can also output any states to clean-up after errors occur"
            n348 = Unbundle By Name(w761) -> ("SelfRef"=w767:refnum<class "Instrument UI.Lockin.lvclass">)
            n349 = call-dynamic "Handle Error.vi"("Stop on Unhandled Error (T)"=FALSE, "error in"=w766, "SMO"=w767) -> ("handling error"=w764:errorcluster, "Unhandled error"=w762:errorcluster)  [unwired: 6 in, 1 out]
            n350 = Bundle By Name(cluster=w761, "Core.Last Error.remaining states"=w758, "Core.Last Error.error"=w762) -> (w760:T63)
            n351 = Select(t="Exit", s=w764, f="Macro: Post Error Handling") -> (s? t:f=w757:string)
          }
          frame "Exit" {
            # "Do not put any code in this frame.\n(No errors that occur here will be handled.)"
            n352 = Unbundle By Name(w770) -> ("Core.Last Error.error"=w769:errorcluster)
            n353 = call <vilib>:"Add State(s) to Queue__jki_lib_state_machine.vi"("State(s) in (\"\")"=w774) -> ("States Out"=w773:string)  [unwired: 14 in]
          }
          frame "---------- Data ----------" {
            # "Do not put any code in this frame.\n(It is a separator no-op. You can make a copy of this frame to create a new Data frame)"
            n354 = call <vilib>:"Add State(s) to Queue__jki_lib_state_machine.vi"("State(s) in (\"\")"=w779) -> ("States Out"=w778:string)  [unwired: 14 in]
          }
          frame "Data: Initialize" {
            w783 = T65 {"Current VI Reference"=refnum, "Close Panel on Exit?"=FALSE, "Last Error"={"error"={"status"=FALSE, "code"=0, "source"=""}, "previous state"="", "remaining states"=""}, "Shutdown?"=FALSE}  # Core
            w782 = refnum<vi> refnum  # Front Panel
            w781 = Get_State-enum."idle"  # DAQ state
            w784 = string[] []  # Plot Names
            w786 = refnum<class "Instrument.Lockin.lvclass"> refnum  # Lockin
            w792 = T45 {"Channels"={"Cfg_AO"=[], "Cfg_AI"=[], "Cfg_REF"=[]}, "DAQ"={"Configuration"=[], "cfg.Sampling"={"Sampling"={"Fs"=0.0, "#s"=0}, "sample mode"=0, "Fs Mode"=enum."Manual", "Fs Multiplier"=0.0, "Refresh Rate (Hz)"=0.0, "Decimation.PreDSP"=0, "Decimation.PostDSP"=0, "Fs.Output"=204789.0}, "Calibration"=[], "Simulation mode"=enum."AI = HW simulated"}, "PreFilter"={"60 Hz"=FALSE, "Low Pass"=FALSE, "Low Pass Cutoff (Hz)"=0.0}, "Amplifers"={"Offset_AI"=[], "Gain_AI"=[], "Gain_AO"=[]}, "Limit Amplitude"={"Limit?"=FALSE, "Limit (V)"=0.0}, "Limit DC"={"Limit?"=FALSE, "Limit (V)"=0.0}, "Link Frequencies"={"Link?"=FALSE, "Frequency (Hz)"=0.0}, "Aux Channel"="", "Sweep"={"Sweep Time (s)"=0.0, "Initial Wait (s)"=0.0, "Return to Start"=FALSE, "Channels"=[]}, "Plot"={"visibility.AI"=[], "visibility.AO"=[], "visibility.Lockin"=[]}}  # UI Config
            w793 = cluster{"Command":variant, "Data":variant} {"Command"=variant, "Data"=variant}  # Message
            w780 = T55 {"DAQ State"=enum."idle", "Waveforms"={"AO_wfm"=[], "AI_wfm"=[], "Ref_X_wfm"=[], "Ref_Y_wfm"=[], "X_wfm"=[], "Y_wfm"=[]}, "Results"={"Time Stamp"=timestamp(0 s since 1904-01-01), "Results (Dictionary)"=[]}, "SweepWaveforms"={"AO_wfm"=[], "AI_wfm"=[], "X_wfm"=[], "Y_wfm"=[]}}  # getAll
            w794 = refnum<class "Configuration.lvclass"> refnum  # Configuration
            w795 = T59 {"Booleans"={"Start"=refnum, "Pause"=refnum, "Reset"=refnum, "Trigger"=refnum, "Help"=refnum, "Close"=refnum, "Start Sweep"=refnum, "Stop Sweep"=refnum}, "Clusters"={"AO Channels"=refnum, "AI Channels"=refnum, "REF Channels"=refnum, "DAQ Config"=refnum, "Sweep Channels"=refnum, "Cal Info"=refnum}, "Graphs"={"AI Graph"=refnum, "AO Graph"=refnum, "Lockin 1"=refnum, "Lockin 2"=refnum, "XY Graph"=refnum, "Sweep X Graph"=refnum, "Sweep Y Graph"=refnum, "Sweep AI Graph"=refnum, "Sweep AO Graph"=refnum, "PS WFGraph"=refnum, "PS Chart"=refnum}}  # References
            # "do not delete - used by framework"
            # "Data names and types of shift register data are defined by this bundle."
            # "Initialize the shift-register data, here.\n(data names are defined by what you wire into the bundle function)"
            n355 = call <userlib>:"Read Instrument.vi"("error in (no error)"=w788, "Instrument UI in"=w790) -> ("error out"=w787:errorcluster, "Instrument"=w791:refnum<class "Instrument.lvclass">)  [unwired: 7 in, 1 out]
            n356 = To More Specific Class(target class=w786, reference=w791, error in=w787) -> (specific class reference=w785:refnum<class "Instrument.Lockin.lvclass">, error out=w789:errorcluster)
            n357 = Bundle("Core"=w783, "SelfRef"=w790, "Lockin"=w785, "Configuration"=w794, "UI Config"=w792, "DAQ state"=w781, "getAll"=w780, "References"=w795, "Message"=w793, "Plot Names"=w784, "Front Panel"=w782) -> (w797:T63)  [unwired: 1 in]
            n358 = call <vilib>:"Add State(s) to Queue__jki_lib_state_machine.vi"("State(s) in (\"\")"=w799) -> ("States Out"=w798:string)  [unwired: 14 in]
          }
          frame "Data: Initialize Control References" {
            n359 = Unbundle By Name(w801) -> ("Core.Current VI Reference"=w800:refnum<vi>)
            n360 = control-ref of="Start"() -> (w810:refnum<vi>)
            n361 = control-ref of="Pause"() -> (w809:refnum<vi>)
            n362 = control-ref of="Reset"() -> (w808:refnum<vi>)
            n363 = control-ref of="Help"() -> (w807:refnum<vi>)
            n364 = control-ref of="Close"() -> (w806:refnum<vi>)
            n365 = control-ref of="Start Sweep"() -> (w805:refnum<vi>)
            n366 = control-ref of="Stop Sweep"() -> (w804:refnum<vi>)
            n367 = control-ref of="AO Channels"() -> (w816:refnum<vi>)
            n368 = control-ref of="AI Channels"() -> (w811:refnum<vi>)
            n369 = control-ref of="REF Channels"() -> (w815:refnum<vi>)
            n370 = control-ref of="DAQ Config"() -> (w814:refnum<vi>)
            n371 = control-ref of="Sweep Channels"() -> (w813:refnum<vi>)
            n372 = control-ref of="Cal Info"() -> (w812:refnum<vi>)
            n373 = property class="VI"(reference=w800) -> ("Front Panel"=w802:refnum<vi>)  [unwired: 1 in, 2 out]
            n374 = Bundle By Name(cluster=w801, "References.Booleans.Start"=w810, "References.Booleans.Pause"=w809, "References.Booleans.Reset"=w808, "References.Booleans.Trigger"=refnum<vi> refnum, "References.Booleans.Help"=w807, "References.Booleans.Close"=w806, "References.Booleans.Start Sweep"=w805, "References.Booleans.Stop Sweep"=w804, "References.Clusters.AO Channels"=w816, "References.Clusters.AI Channels"=w811, "References.Clusters.REF Channels"=w815, "References.Clusters.DAQ Config"=w814, "References.Clusters.Sweep Channels"=w813, "References.Clusters.Cal Info"=w812, "Front Panel"=w802) -> (w817:T63)
            n375 = call <vilib>:"Add State(s) to Queue__jki_lib_state_machine.vi"("State(s) in (\"\")"=w821) -> ("States Out"=w820:string)  [unwired: 14 in]
          }
          frame "Data: Initialize Graph References" {
            n376 = control-ref of="AI Graph"() -> (w834:refnum<vi>)
            n377 = control-ref of="AO Graph"() -> (w833:refnum<vi>)
            n378 = control-ref of="Lockin 1"() -> (w832:refnum<vi>)
            n379 = control-ref of="Lockin 2"() -> (w831:refnum<vi>)
            n380 = control-ref of="XY Graph"() -> (w830:refnum<vi>)
            n381 = control-ref of="Sweep Results X"() -> (w822:refnum<vi>)
            n382 = control-ref of="Sweep Results Y"() -> (w823:refnum<vi>)
            n383 = control-ref of="Sweep AI"() -> (w824:refnum<vi>)
            n384 = control-ref of="Sweep AO"() -> (w825:refnum<vi>)
            n385 = control-ref of="PS WFGraph"() -> (w829:refnum<vi>)
            n386 = control-ref of="PS Chart"() -> (w828:refnum<vi>)
            n387 = Bundle By Name(cluster=w827, "References.Graphs.AI Graph"=w834, "References.Graphs.AO Graph"=w833, "References.Graphs.Lockin 1"=w832, "References.Graphs.Lockin 2"=w831, "References.Graphs.XY Graph"=w830, "References.Graphs.Sweep X Graph"=w822, "References.Graphs.Sweep Y Graph"=w823, "References.Graphs.Sweep AI Graph"=w824, "References.Graphs.Sweep AO Graph"=w825, "References.Graphs.PS WFGraph"=w829, "References.Graphs.PS Chart"=w828) -> (w826:T63)
            n388 = call <vilib>:"Add State(s) to Queue__jki_lib_state_machine.vi"("State(s) in (\"\")"=w838) -> ("States Out"=w837:string)  [unwired: 14 in]
          }
          frame "Data: Wait" {
            # "Do not put any code in this frame.\n(It is a separator no-op. You can make a copy of this frame to create a new Data frame)"
            n389 = Scan From String(input string=w839, default 1=u32 0 ("milliseconds to wait")) -> (output 1=w840:u32)  [unwired: 3 in, 3 out]
            n390 = Wait (ms)(milliseconds to wait=w840) -> ()  [unwired: 1 out]
            n391 = call <vilib>:"Add State(s) to Queue__jki_lib_state_machine.vi"("State(s) in (\"\")"=w846) -> ("States Out"=w845:string)  [unwired: 14 in]
          }
          frame "Data: Cleanup" {
            # "Cleanup any data and references, here.\n(this is called automatically, by the Macro: Exit)"
            n392 = Unbundle By Name(w848) -> ("Core.Current VI Reference"=w851:refnum<vi>)
            n393 = Close Reference(reference=w851, error in (no error)=w850) -> (error out=w849:errorcluster)
            n394 = call <vilib>:"Add State(s) to Queue__jki_lib_state_machine.vi"("State(s) in (\"\")"=w853) -> ("States Out"=w852:string)  [unwired: 14 in]
          }
          frame "---------- Configuration ----------" {
            # "Do not put any code in this frame.\n(It is a separator no-op. You can make a copy of this frame to create a new Data frame)"
            n395 = call <vilib>:"Add State(s) to Queue__jki_lib_state_machine.vi"("State(s) in (\"\")"=w858) -> ("States Out"=w857:string)  [unwired: 14 in]
          }
          frame "Configuration: Initialize" {
            # "Do not put any code in this frame.\n(It is a separator no-op. You can make a copy of this frame to create a new Data frame)"
            n396 = Unbundle By Name(w868) -> ("Lockin"=w867:refnum<class "Instrument.Lockin.lvclass">)
            n397 = call <vilib>:"GetName.vi"("error in (no error)"=w866, "SMO"=w867) -> ("error out"=w864:errorcluster, "Name"=w865:string)  [unwired: 6 in, 2 out]
            n398 = call <userlib>:"Default Path.vi"("error in (no error)"=w864, "Folder Name [Application Name]"=w865) -> ("error out"=w861:errorcluster, "Configuration out"=w863:refnum<class "Configuration.lvclass">)  [unwired: 8 in]
            n399 = call <userlib>:"Write Section.vi"("error in (no error)"=w861, "Section"="UI", "Configuration in"=w863) -> ("error out"=w860:errorcluster, "Configuration out"=w862:refnum<class "Configuration.lvclass">)  [unwired: 7 in]
            n400 = Bundle By Name(cluster=w868, "Configuration"=w862) -> (w869:T63)
            n401 = call <vilib>:"Add State(s) to Queue__jki_lib_state_machine.vi"("State(s) in (\"\")"=w872) -> ("States Out"=w871:string)  [unwired: 14 in]
          }
          frame "Configuration: Write File" {
            # "Do not put any code in this frame.\n(It is a separator no-op. You can make a copy of this frame to create a new Data frame)"
            n402 = Unbundle By Name(w878) -> ("Configuration"=w873:refnum<class "Configuration.lvclass">, "UI Config"=w874:T45)
            n403 = call <userlib>:"Write Configuration.vi"("error in (no error)"=w875, "Variant"=w874, "Configuration in"=w873) -> ("error out"=w877:errorcluster, "Configuration out"=w876:refnum<class "Configuration.lvclass">)  [unwired: 7 in]
            n404 = Bundle By Name(cluster=w878, "Configuration"=w876) -> (w879:T63)
            n405 = call <vilib>:"Add State(s) to Queue__jki_lib_state_machine.vi"("State(s) in (\"\")"=w882) -> ("States Out"=w881:string)  [unwired: 14 in]
          }
          frame "Configuration: Read File" {
            # "Do not put any code in this frame.\n(It is a separator no-op. You can make a copy of this frame to create a new Data frame)"
            n406 = Unbundle By Name(w891) -> ("Configuration"=w883:refnum<class "Configuration.lvclass">, "UI Config"=w885:T45)
            n407 = call <userlib>:"Read Configuration.vi"("INI Fomatted Cluster Type"=w885, "error in (no error)"=w887, "Configuration in"=w883) -> ("error out"=w889:errorcluster, "Configuration"=w890:variant, "Configuration out"=w888:refnum<class "Configuration.lvclass">)  [unwired: 6 in]
            n408 = Variant To Data(error in=w889, type=w885, Variant=w890) -> (data=w884:T45, error out=w886:errorcluster)
            n409 = Bundle By Name(cluster=w891, "Configuration"=w888, "UI Config"=w884) -> (w892:T63)
            n410 = call <vilib>:"Add State(s) to Queue__jki_lib_state_machine.vi"("State(s) in (\"\")"=w895) -> ("States Out"=w894:string)  [unwired: 14 in]
          }
          frame "---------- UI ----------" {
            # "Do not put any code in this frame.\n(It is a separator no-op. You can make a copy of this frame to create a new UI frame)"
            n411 = call <vilib>:"Add State(s) to Queue__jki_lib_state_machine.vi"("State(s) in (\"\")"=w900) -> ("States Out"=w899:string)  [unwired: 14 in]
          }
          frame "UI: Initialize" {
            # "size window to decoration box on front panel"
            # "Initialize the User Interface here.\n(this is called automatically, by the Macro: Init)"
            n412 = call "Application Version.vi"() -> ("Version"=→"Version":string)
            n413 = call <userlib>:"Fit VI window to Largest Dec__ogtk.vi"("error in (no error)"=w908, "border spacing (2 px)"=-4) -> ("error out"=w907:errorcluster)  [unwired: 4 in, 1 out]
            n414 = call <vilib>:"Build State String with Arguments__JKI_lib_State_Machine.vi"("Arguments (\"\")"="Initializing..." ("Status"), "State"="UI: Update Status") -> ("State with Arguments"=w902:string)  [unwired: 4 in]
            n415 = call <vilib>:"Add State(s) to Queue__jki_lib_state_machine.vi"("State(s) in Front (\"\")"=w902, "State(s) in (\"\")"=w911) -> ("States Out"=w910:string)  [unwired: 13 in]
          }
          frame "UI: Set Left Tab" {
            w913 = T1."AO/AI/REF"  # Left Tab
            # "Do not put any code in this frame.\n(It is a separator no-op. You can make a copy of this frame to create a new UI frame)"
            n416 = Scan From String(input string=w914, default 1=w913) -> (output 1=w912:T1)  [unwired: 3 in, 3 out]
            n417 = local write "Left Tab"(w912) -> ()
            n418 = call <vilib>:"Add State(s) to Queue__jki_lib_state_machine.vi"("State(s) in (\"\")"=w919) -> ("States Out"=w918:string)  [unwired: 14 in]
          }
          frame "UI: Set Right Tab" {
            w920 = T26."AO/AI"  # Right Tab
            # "Do not put any code in this frame.\n(It is a separator no-op. You can make a copy of this frame to create a new UI frame)"
            n419 = Scan From String(input string=w922, default 1=w920) -> (output 1=w921:T26)  [unwired: 3 in, 3 out]
            n420 = local write "Right Tab"(w921) -> ()
            n421 = call <vilib>:"Add State(s) to Queue__jki_lib_state_machine.vi"("State(s) in (\"\")"=w927) -> ("States Out"=w926:string)  [unwired: 14 in]
          }
          frame "UI: Update Status" {
            # "Do not put any code in this frame.\n(It is a separator no-op. You can make a copy of this frame to create a new UI frame)"
            n422 = case shown="Default" w928 {
              selector: w928 -> [w934 _]
              frame Default {
                "Status" <- w934
              }
              frame "" {
              }
            }
            n423 = call <vilib>:"Add State(s) to Queue__jki_lib_state_machine.vi"("State(s) in (\"\")"=w933) -> ("States Out"=w932:string)  [unwired: 14 in]
          }
          frame "UI: Cluster to UI" {
            # "Initialize the UI elements from data wire\n(this is called automatically, by the Macro: Init)"
            n424 = Unbundle By Name(w943) -> ("UI Config.Channels.Cfg_AO"=w958:T4, "UI Config.Channels.Cfg_AI"=w956:T2, "UI Config.Channels.Cfg_REF"=w957:T7, "UI Config.DAQ.Configuration"=w950:T11, "UI Config.DAQ.cfg.Sampling.Sampling.Fs"=w941:dbl, "UI Config.DAQ.cfg.Sampling.Sampling.#s"=w938:i32, "UI Config.DAQ.cfg.Sampling.Fs Mode"=w940:T16, "UI Config.DAQ.cfg.Sampling.Fs Multiplier"=w951:dbl, "UI Config.DAQ.cfg.Sampling.Refresh Rate (Hz)"=w952:dbl, "UI Config.DAQ.cfg.Sampling.Fs.Output"=w939:dbl, "UI Config.DAQ.cfg.Sampling.Decimation.PreDSP"=w948:i32, "UI Config.DAQ.Simulation mode"=w949:T17, "UI Config.PreFilter.60 Hz"=w955:bool, "UI Config.PreFilter.Low Pass"=w954:bool, "UI Config.PreFilter.Low Pass Cutoff (Hz)"=w953:dbl, "UI Config.Amplifers.Offset_AI"=w942:T9, "UI Config.Amplifers.Gain_AI"=w936:T9, "UI Config.Amplifers.Gain_AO"=w937:T9, "UI Config.Sweep.Sweep Time (s)"=w944:dbl, "UI Config.Sweep.Initial Wait (s)"=w945:dbl, "UI Config.Sweep.Return to Start"=w946:bool, "UI Config.Sweep.Channels"=w947:T18)
            n425 = local write "Input Offsets"(w942) -> ()
            n426 = local write "Input Gain"(w936) -> ()
            n427 = local write "Output Gain"(w937) -> ()
            n428 = local write "Fs Output (S/s)"(w939) -> ()
            n429 = local write "Fs (S/s)"(w941) -> ()
            n430 = local write "#s (S)"(w938) -> ()
            n431 = local write "AO Channels"(w958) -> ()
            n432 = local write "AI Channels"(w956) -> ()
            n433 = local write "REF Channels"(w957) -> ()
            n434 = local write "DAQ Config"(w950) -> ()
            n435 = property on="Fs Mode" class="Enum (strict)"("Val(Sgnl)"=w940) -> ()  [unwired: 2 in, 2 out]
            n436 = local write "Fs Multiplier"(w951) -> ()
            n437 = local write "Refresh Rate (Hz)"(w952) -> ()
            n438 = local write "Decimation (pre DSP)"(w948) -> ()
            n439 = local write "AI Simulation mode"(w949) -> ()
            n440 = local write "Line"(w955) -> ()
            n441 = local write "Lowpass"(w954) -> ()
            n442 = local write "LP f (Hz)"(w953) -> ()
            n443 = local write "Sweep Time (s)"(w944) -> ()
            n444 = local write "Initial Wait (s)"(w945) -> ()
            n445 = local write "Return to Start?"(w946) -> ()
            n446 = local write "Sweep Channels"(w947) -> ()
            n447 = call <vilib>:"Add State(s) to Queue__jki_lib_state_machine.vi"("State(s) in Front (\"\")"="UI: Cluster to UI 2" ("State(s) in Front (\"\")"), "State(s) in (\"\")"=w962) -> ("States Out"=w961:string)  [unwired: 13 in]
          }
          frame "UI: Cluster to UI 2" {
            # "Initialize the UI elements from data wire (2)\n(this is called automatically by UI: Cluster to UI)"
            n448 = Unbundle By Name(w969) -> ("UI Config.Limit Amplitude.Limit?"=w968:bool, "UI Config.Limit Amplitude.Limit (V)"=w967:dbl, "UI Config.Limit DC.Limit?"=w964:bool, "UI Config.Limit DC.Limit (V)"=w963:dbl, "UI Config.Link Frequencies.Link?"=w965:bool, "UI Config.Link Frequencies.Frequency (Hz)"=w966:dbl)
            n449 = local write "Limit Amplitude (V)"(w968) -> ()
            n450 = local write "Limit DC (V)"(w964) -> ()
            n451 = local write "Link Frequencies"(w965) -> ()
            n452 = local write "AO Amp Limit"(w967) -> ()
            n453 = local write "AO DC Limit"(w963) -> ()
            n454 = local write "AO freq link"(w966) -> ()
            n455 = call <vilib>:"Add State(s) to Queue__jki_lib_state_machine.vi"("State(s) in (\"\")"=w973) -> ("States Out"=w972:string)  [unwired: 14 in]
          }
          frame "UI: UI to Cluster" {
            # "Write UI elements to data wire\n(this is called automatically, by the Macro: Init)"
            n456 = local read "AO Channels"() -> (w996:T4)
            n457 = local read "AI Channels"() -> (w994:T2)
            n458 = local read "REF Channels"() -> (w995:T7)
            n459 = local read "DAQ Config"() -> (w987:T11)
            n460 = local read "Fs Mode"() -> (w990:T16)
            n461 = local read "Fs Multiplier"() -> (w988:dbl)
            n462 = local read "Refresh Rate (Hz)"() -> (w989:dbl)
            n463 = local read "Decimation (pre DSP)"() -> (w985:i32)
            n464 = local read "AI Simulation mode"() -> (w986:T17)
            n465 = local read "Line"() -> (w993:bool)
            n466 = local read "Lowpass"() -> (w992:bool)
            n467 = local read "LP f (Hz)"() -> (w991:dbl)
            n468 = local read "Sweep Time (s)"() -> (w981:dbl)
            n469 = local read "Initial Wait (s)"() -> (w982:dbl)
            n470 = local read "Return to Start?"() -> (w983:bool)
            n471 = local read "Sweep Channels"() -> (w984:T18)
            n472 = local read "Fs (S/s)"() -> (w976:dbl)
            n473 = local read "#s (S)"() -> (w977:i32)
            n474 = local read "Fs Output (S/s)"() -> (w975:dbl)
            n475 = local read "Input Offsets"() -> (w978:T9)
            n476 = local read "Input Gain"() -> (w980:T9)
            n477 = local read "Output Gain"() -> (w979:T9)
            n478 = Bundle By Name(cluster=w997, "UI Config.Channels.Cfg_AO"=w996, "UI Config.Channels.Cfg_AI"=w994, "UI Config.Channels.Cfg_REF"=w995, "UI Config.DAQ.Configuration"=w987, "UI Config.DAQ.cfg.Sampling.Sampling.Fs"=w976, "UI Config.DAQ.cfg.Sampling.Sampling.#s"=w977, "UI Config.DAQ.cfg.Sampling.Fs Mode"=w990, "UI Config.DAQ.cfg.Sampling.Fs Multiplier"=w988, "UI Config.DAQ.cfg.Sampling.Refresh Rate (Hz)"=w989, "UI Config.DAQ.cfg.Sampling.Fs.Output"=w975, "UI Config.DAQ.cfg.Sampling.Decimation.PreDSP"=w985, "UI Config.DAQ.Simulation mode"=w986, "UI Config.PreFilter.60 Hz"=w993, "UI Config.PreFilter.Low Pass"=w992, "UI Config.PreFilter.Low Pass Cutoff (Hz)"=w991, "UI Config.Amplifers.Offset_AI"=w978, "UI Config.Amplifers.Gain_AI"=w980, "UI Config.Amplifers.Gain_AO"=w979, "UI Config.Sweep.Sweep Time (s)"=w981, "UI Config.Sweep.Initial Wait (s)"=w982, "UI Config.Sweep.Return to Start"=w983, "UI Config.Sweep.Channels"=w984) -> (w998:T63)
            n479 = call <vilib>:"Add State(s) to Queue__jki_lib_state_machine.vi"("State(s) in Front (\"\")"="UI: UI to Cluster 2" ("State(s) in Front (\"\")"), "State(s) in (\"\")"=w1002) -> ("States Out"=w1001:string)  [unwired: 13 in]
          }
          frame "UI: UI to Cluster 2" {
            # "Write UI elements to data wire (2)\n(this is called automatically by the UI: UI to Cluster)"
            n480 = local read "Limit Amplitude (V)"() -> (w1010:bool)
            n481 = local read "Limit DC (V)"() -> (w1008:bool)
            n482 = local read "Link Frequencies"() -> (w1006:bool)
            n483 = local read "AO Amp Limit"() -> (w1009:dbl)
            n484 = local read "AO DC Limit"() -> (w1007:dbl)
            n485 = local read "AO freq link"() -> (w1005:dbl)
            n486 = Bundle By Name(cluster=w1003, "UI Config.Limit Amplitude.Limit?"=w1010, "UI Config.Limit Amplitude.Limit (V)"=w1009, "UI Config.Limit DC.Limit?"=w1008, "UI Config.Limit DC.Limit (V)"=w1007, "UI Config.Link Frequencies.Link?"=w1006, "UI Config.Link Frequencies.Frequency (Hz)"=w1005) -> (w1004:T63)
            n487 = call <vilib>:"Add State(s) to Queue__jki_lib_state_machine.vi"("State(s) in (\"\")"=w1014) -> ("States Out"=w1013:string)  [unwired: 14 in]
          }
          frame "UI: Reinit To Default" {
            # "Do not put any code in this frame.\n(It is a separator no-op. You can make a copy of this frame to create a new UI frame)"
            n488 = Unbundle By Name(w1015) -> ("References.Booleans"=w1017:T60, "References.Graphs.Lockin 1"=w1019:refnum<vi>, "References.Graphs.Lockin 2"=w1018:refnum<vi>)
            n489 = Cluster To Array(cluster=w1017) -> (array=w1016:refnum<vi>[])
            n490 = for {
              tunnel: w1016 -> [w1024] mode=indexing
              n491 = invoke on="Invoke Node" class="Bool (strict)" method="Reinit To Default"(reference=w1024) -> ()  [unwired: 2 in, 3 out]
            }
            n492 = invoke on="Invoke Node" class="WFChart (strict)" method="Reinit To Default"(reference=w1019) -> ()  [unwired: 2 in, 3 out]
            n493 = invoke on="Invoke Node" class="WFChart (strict)" method="Reinit To Default"(reference=w1018) -> ()  [unwired: 2 in, 3 out]
            n494 = call <vilib>:"Add State(s) to Queue__jki_lib_state_machine.vi"("State(s) in (\"\")"=w1023) -> ("States Out"=w1022:string)  [unwired: 14 in]
          }
          frame "UI: Disable Buttons" {
            # "Disable all booleans\n()"
            n495 = Unbundle By Name(w1026) -> ("References.Booleans"=w1027:T60)
            n496 = Cluster To Array(cluster=w1027) -> (array=w1025:refnum<vi>[])
            n497 = for {
              tunnel: w1025 -> [w1032] mode=indexing
              n498 = property class="Bool (strict)"(reference=w1032, "DisabledEnum"=T36."Disabled and Grayed Out" ("Disabled")) -> ()  [unwired: 1 in, 2 out]
            }
            n499 = call <vilib>:"Add State(s) to Queue__jki_lib_state_machine.vi"("State(s) in (\"\")"=w1031) -> ("States Out"=w1030:string)  [unwired: 14 in]
          }
          frame "UI: Enable Buttons" {
            # "Enable booleans after SMO starts.\n()"
            n500 = Unbundle By Name(w1036) -> ("References.Booleans"=w1035:T60)
            n501 = Cluster To Array(cluster=w1035) -> (array=w1034:refnum<vi>[])
            n502 = for {
              tunnel: w1034 -> [w1041] mode=indexing
              n503 = property class="Bool (strict)"(reference=w1041, "DisabledEnum"=T36."Enabled" ("Disabled")) -> ()  [unwired: 1 in, 2 out]
            }
            n504 = call <vilib>:"Add State(s) to Queue__jki_lib_state_machine.vi"("State(s) in (\"\")"=w1040) -> ("States Out"=w1039:string)  [unwired: 14 in]
          }
          frame "UI: AI Graphs Plot Visibility" {
            # "Do not put any code in this frame.\n(It is a separator no-op. You can make a copy of this frame to create a new UI frame)"
            n505 = Unbundle By Name(w1047) -> ("References.Graphs.AI Graph"=w1046:refnum<vi>, "References.Graphs.Sweep AI Graph"=w1043:refnum<vi>)
            n506 = case shown="\"None\", Default" w1045 {
              tunnel: [FALSE TRUE] -> w1044
              frame "None", Default {
              }
              frame "ALL" {
              }
            }
            n507 = call-poly "Set All Plot Visibility.vi"("error in (no error)"=w1048, "All Visible?"=w1044, "WFGraph in"=w1043) -> ("error out"=w1050:errorcluster)  [unwired: 7 in, 1 out]
            n508 = call-poly "Set All Plot Visibility.vi"("error in (no error)"=w1050, "All Visible?"=w1044, "WFGraph in"=w1046) -> ("error out"=w1049:errorcluster)  [unwired: 7 in, 1 out]
            n509 = call <vilib>:"Add State(s) to Queue__jki_lib_state_machine.vi"("State(s) in (\"\")"=w1053) -> ("States Out"=w1052:string)  [unwired: 14 in]
          }
          frame "UI: AO Graphs Plot Visibility" {
            # "Do not put any code in this frame.\n(It is a separator no-op. You can make a copy of this frame to create a new UI frame)"
            n510 = Unbundle By Name(w1060) -> ("References.Graphs.AO Graph"=w1059:refnum<vi>, "References.Graphs.Sweep AO Graph"=w1056:refnum<vi>)
            n511 = case shown="\"ALL\"" w1058 {
              tunnel: [FALSE TRUE] -> w1063
              frame "None", Default {
              }
              frame "ALL" {
              }
            }
            n512 = call-poly "Set All Plot Visibility.vi"("error in (no error)"=w1061, "All Visible?"=w1063, "WFGraph in"=w1056) -> ("error out"=w1062:errorcluster)  [unwired: 7 in, 1 out]
            n513 = call-poly "Set All Plot Visibility.vi"("error in (no error)"=w1062, "All Visible?"=w1063, "WFGraph in"=w1059) -> ("error out"=w1057:errorcluster)  [unwired: 7 in, 1 out]
            n514 = call <vilib>:"Add State(s) to Queue__jki_lib_state_machine.vi"("State(s) in (\"\")"=w1066) -> ("States Out"=w1065:string)  [unwired: 14 in]
          }
          frame "UI: Lockin Graphs Plot Visibility" {
            # "Do not put any code in this frame.\n(It is a separator no-op. You can make a copy of this frame to create a new UI frame)"
            n515 = Unbundle By Name(w1080) -> ("References.Graphs.Lockin 1"=w1071:refnum<vi>, "References.Graphs.Lockin 2"=w1072:refnum<vi>, "References.Graphs.XY Graph"=w1073:refnum<vi>, "References.Graphs.Sweep X Graph"=w1070:refnum<vi>, "References.Graphs.Sweep Y Graph"=w1069:refnum<vi>)
            n516 = case shown="\"None\", Default" w1079 {
              tunnel: [FALSE TRUE] -> w1074
              frame "None", Default {
              }
              frame "ALL" {
              }
            }
            n517 = call-poly "Set All Plot Visibility.vi"("error in (no error)"=w1081, "All Visible?"=w1074, "WFGraph in"=w1069) -> ("error out"=w1082:errorcluster)  [unwired: 7 in, 1 out]
            n518 = call-poly "Set All Plot Visibility.vi"("error in (no error)"=w1082, "All Visible?"=w1074, "WFGraph in"=w1070) -> ("error out"=w1078:errorcluster)  [unwired: 7 in, 1 out]
            n519 = call-poly "Set All Plot Visibility.vi"("error in (no error)"=w1078, "All Visible?"=w1074, "XYGraph in"=w1073) -> ("error out"=w1077:errorcluster)  [unwired: 7 in, 1 out]
            n520 = call-poly "Set All Plot Visibility.vi"("error in (no error)"=w1077, "All Visible?"=w1074, "WaveformChart in"=w1072) -> ("error out"=w1076:errorcluster)  [unwired: 7 in, 1 out]
            n521 = call-poly "Set All Plot Visibility.vi"("error in (no error)"=w1076, "All Visible?"=w1074, "WaveformChart in"=w1071) -> ("error out"=w1075:errorcluster)  [unwired: 7 in, 1 out]
            n522 = call <vilib>:"Add State(s) to Queue__jki_lib_state_machine.vi"("State(s) in (\"\")"=w1085) -> ("States Out"=w1084:string)  [unwired: 14 in]
          }
          frame "UI: Get Plot Visibility" {
            # "Do not put any code in this frame.\n(It is a separator no-op. You can make a copy of this frame to create a new UI frame)"
            n523 = Unbundle By Name(w1104) -> ("References.Graphs.AI Graph"=w1099:refnum<vi>, "UI Config.DAQ.Configuration"=w1090:T11, "References.Graphs.AO Graph"=w1098:refnum<vi>, "References.Graphs.Lockin 1"=w1100:refnum<vi>, "Plot Names"=w1101:string[])  [unwired: 1 out]
            n524 = call "Get AO Channel Count.vi"("DAQ []"=w1090) -> ("# AO channels"=w1089:i32)  [unwired: 2 in]
            n525 = call "Get AI Channel Count.vi"("DAQ []"=w1090) -> ("# AI channels"=w1088:i32)  [unwired: 2 in]
            n526 = for {
              N: w1088 -> [_]
              tunnel: w1099 -> [w1112]
              tunnel: [w1110] -> w1096 mode=indexing
              tunnel: w1091 -> [w1109]
              tunnel: [w1108] -> w1092 mode=indexing
              i -> [w1111]
              n527 = call-poly "Get Plot Visibility.vi"("error in (no error)"=w1109, "ActPlot"=w1111, "WFGraph in"=w1112) -> ("error out"=w1108:errorcluster, "Plot.Visible?"=w1110:bool)  [unwired: 6 in, 1 out]
            }
            n528 = for {
              N: w1089 -> [_]
              tunnel: w1098 -> [w1117]
              tunnel: [w1115] -> w1097 mode=indexing
              tunnel: w1091 -> [w1114]
              tunnel: [w1113] -> w1093 mode=indexing
              i -> [w1116]
              n529 = call-poly "Get Plot Visibility.vi"("error in (no error)"=w1114, "ActPlot"=w1116, "WFGraph in"=w1117) -> ("error out"=w1113:errorcluster, "Plot.Visible?"=w1115:bool)  [unwired: 6 in, 1 out]
            }
            n530 = for {
              tunnel: w1100 -> [w1122]
              tunnel: w1101 -> [_] mode=indexing
              tunnel: [w1120] -> w1102 mode=indexing
              tunnel: [w1119] -> w1095 mode=indexing
              tunnel: w1091 -> [w1118]
              i -> [w1121]
              n531 = call-poly "Get Plot Visibility.vi"("error in (no error)"=w1118, "ActPlot"=w1121, "WaveformChart in"=w1122) -> ("error out"=w1119:errorcluster, "Plot.Visible?"=w1120:bool)  [unwired: 6 in, 1 out]
            }
            n532 = Bundle By Name(cluster=w1104, "UI Config.Plot.visibility.AI"=w1096, "UI Config.Plot.visibility.AO"=w1097, "UI Config.Plot.visibility.Lockin"=w1102) -> (w1103:T63)
            n533 = Merge Errors(w1092, w1093, w1095) -> (w1094:errorcluster)
            n534 = call <vilib>:"Add State(s) to Queue__jki_lib_state_machine.vi"("State(s) in (\"\")"=w1107) -> ("States Out"=w1106:string)  [unwired: 14 in]
          }
          frame "UI: Set Plot Visibility" {
            # "Do not put any code in this frame.\n(It is a separator no-op. You can make a copy of this frame to create a new UI frame)"
            n535 = Unbundle By Name(w1123) -> ("References.Graphs.AI Graph"=w1132:refnum<vi>, "UI Config.Plot.visibility.AI"=w1131:bool[], "References.Graphs.AO Graph"=w1130:refnum<vi>, "UI Config.Plot.visibility.AO"=w1129:bool[], "References.Graphs.Lockin 1"=w1133:refnum<vi>, "UI Config.Plot.visibility.Lockin"=w1134:bool[])
            n536 = for {
              tunnel: w1132 -> [w1142]
              tunnel: w1131 -> [w1138] mode=indexing
              tunnel: w1124 -> [w1140]
              tunnel: [w1139] -> w1125 mode=indexing
              i -> [w1141]
              n537 = call-poly "Set Plot Visibility.vi"("error in (no error)"=w1140, "Plot.Visible?"=w1138, "ActPlot"=w1141, "WFGraph in"=w1142) -> ("error out"=w1139:errorcluster)  [unwired: 6 in, 1 out]
            }
            n538 = for {
              tunnel: w1130 -> [w1147]
              tunnel: w1129 -> [w1143] mode=indexing
              tunnel: w1124 -> [w1145]
              tunnel: [w1144] -> w1126 mode=indexing
              i -> [w1146]
              n539 = call-poly "Set Plot Visibility.vi"("error in (no error)"=w1145, "Plot.Visible?"=w1143, "ActPlot"=w1146, "WFGraph in"=w1147) -> ("error out"=w1144:errorcluster)  [unwired: 6 in, 1 out]
            }
            n540 = for {
              tunnel: w1133 -> [w1152]
              tunnel: w1134 -> [w1148] mode=indexing
              tunnel: [w1150] -> w1128 mode=indexing
              tunnel: w1124 -> [w1149]
              i -> [w1151]
              n541 = call-poly "Set Plot Visibility.vi"("error in (no error)"=w1149, "Plot.Visible?"=w1148, "ActPlot"=w1151, "WaveformChart in"=w1152) -> ("error out"=w1150:errorcluster)  [unwired: 6 in, 1 out]
            }
            n542 = Merge Errors(w1125, w1126, w1128) -> (w1127:errorcluster)
            n543 = call <vilib>:"Add State(s) to Queue__jki_lib_state_machine.vi"("State(s) in (\"\")"=w1137) -> ("States Out"=w1136:string)  [unwired: 14 in]
          }
          frame "UI: Sync AI Plot Visibility" {
            # "Do not put any code in this frame.\n(It is a separator no-op. You can make a copy of this frame to create a new UI frame)"
            n544 = Unbundle By Name(w1161) -> ("UI Config.DAQ.Configuration"=w1156:T11, "References.Graphs.PS WFGraph"=w1154:refnum<vi>, "References.Graphs.Sweep AI Graph"=w1157:refnum<vi>, "References.Graphs.AI Graph"=w1158:refnum<vi>)
            n545 = call "Get AI Channel Count.vi"("DAQ []"=w1156) -> ("# AI channels"=w1159:i32)  [unwired: 2 in]
            n546 = for {
              N: w1159 -> [_]
              tunnel: w1158 -> [w1174]
              tunnel: w1157 -> [w1170]
              tunnel: [w1165] -> w1153 mode=indexing
              tunnel: w1155 -> [w1175]
              tunnel: w1154 -> [w1169]
              i -> [w1171]
              n547 = call-poly "Get Plot Visibility.vi"("error in (no error)"=w1175, "ActPlot"=w1171, "WFGraph in"=w1174) -> ("error out"=w1172:errorcluster, "Plot.Visible?"=w1167:bool, "Active Plot"=w1173:i32)  [unwired: 6 in]
              n548 = call-poly "Set Plot Visibility.vi"("error in (no error)"=w1172, "Plot.Visible?"=w1167, "ActPlot"=w1173, "WFGraph in"=w1170) -> ("error out"=w1166:errorcluster, "Active Plot"=w1168:i32)  [unwired: 6 in]
              n549 = call-poly "Set Plot Visibility.vi"("error in (no error)"=w1166, "Plot.Visible?"=w1167, "ActPlot"=w1168, "WFGraph (WDT) in"=w1169) -> ("error out"=w1165:errorcluster)  [unwired: 6 in, 1 out]
            }
            n550 = Merge Errors(w1153) -> (w1160:errorcluster)
            n551 = call <vilib>:"Add State(s) to Queue__jki_lib_state_machine.vi"("State(s) in (\"\")"=w1164) -> ("States Out"=w1163:string)  [unwired: 14 in]
          }
          frame "UI: Sync AO Plot Visibility" {
            # "Do not put any code in this frame.\n(It is a separator no-op. You can make a copy of this frame to create a new UI frame)"
            n552 = Unbundle By Name(w1183) -> ("UI Config.DAQ.Configuration"=w1176:T11, "References.Graphs.Sweep AO Graph"=w1182:refnum<vi>, "References.Graphs.AO Graph"=w1179:refnum<vi>)
            n553 = call "Get AO Channel Count.vi"("DAQ []"=w1176) -> ("# AO channels"=w1180:i32)  [unwired: 2 in]
            n554 = for {
              N: w1180 -> [_]
              tunnel: w1179 -> [w1193]
              tunnel: w1182 -> [w1187]
              tunnel: [w1189] -> w1178 mode=indexing
              tunnel: w1177 -> [w1194]
              i -> [w1188]
              n555 = call-poly "Get Plot Visibility.vi"("error in (no error)"=w1194, "ActPlot"=w1188, "WFGraph in"=w1193) -> ("error out"=w1190:errorcluster, "Plot.Visible?"=w1191:bool, "Active Plot"=w1192:i32)  [unwired: 6 in]
              n556 = call-poly "Set Plot Visibility.vi"("error in (no error)"=w1190, "Plot.Visible?"=w1191, "ActPlot"=w1192, "WFGraph in"=w1187) -> ("error out"=w1189:errorcluster)  [unwired: 6 in, 1 out]
            }
            n557 = Merge Errors(w1178) -> (w1181:errorcluster)
            n558 = call <vilib>:"Add State(s) to Queue__jki_lib_state_machine.vi"("State(s) in (\"\")"=w1186) -> ("States Out"=w1185:string)  [unwired: 14 in]
          }
          frame "UI: Sync Lockin Plot Visibility" {
            # "Do not put any code in this frame.\n(It is a separator no-op. You can make a copy of this frame to create a new UI frame)"
            n559 = Unbundle By Name(w1204) -> ("References.Graphs.Sweep X Graph"=w1197:refnum<vi>, "References.Graphs.Sweep Y Graph"=w1198:refnum<vi>, "References.Graphs.XY Graph"=w1199:refnum<vi>, "References.Graphs.Lockin 2"=w1203:refnum<vi>, "References.Graphs.Lockin 1"=w1201:refnum<vi>, "Plot Names"=w1196:string[])
            n560 = for {
              tunnel: w1201 -> [w1223]
              tunnel: w1203 -> [w1222]
              tunnel: [w1213] -> w1200 mode=indexing
              tunnel: w1195 -> [w1224]
              tunnel: w1199 -> [w1212]
              tunnel: w1198 -> [w1209]
              tunnel: w1197 -> [w1208]
              tunnel: w1196 -> [_] mode=indexing
              i -> [w1219]
              n561 = call-poly "Get Plot Visibility.vi"("error in (no error)"=w1224, "ActPlot"=w1219, "WaveformChart in"=w1223) -> ("error out"=w1220:errorcluster, "Plot.Visible?"=w1215:bool, "Active Plot"=w1221:i32)  [unwired: 6 in]
              n562 = call-poly "Set Plot Visibility.vi"("error in (no error)"=w1220, "Plot.Visible?"=w1215, "ActPlot"=w1221, "WaveformChart in"=w1222) -> ("error out"=w1216:errorcluster, "Active Plot"=w1211:i32)  [unwired: 6 in]
              n563 = call-poly "Set Plot Visibility.vi"("error in (no error)"=w1216, "Plot.Visible?"=w1215, "ActPlot"=w1211, "XYGraph in"=w1212) -> ("error out"=w1218:errorcluster, "Active Plot"=w1217:i32)  [unwired: 6 in]
              n564 = call-poly "Set Plot Visibility.vi"("error in (no error)"=w1218, "Plot.Visible?"=w1215, "ActPlot"=w1217, "WFGraph in"=w1209) -> ("error out"=w1214:errorcluster, "Active Plot"=w1210:i32)  [unwired: 6 in]
              n565 = call-poly "Set Plot Visibility.vi"("error in (no error)"=w1214, "Plot.Visible?"=w1215, "ActPlot"=w1210, "WFGraph in"=w1208) -> ("error out"=w1213:errorcluster)  [unwired: 6 in, 1 out]
            }
            n566 = Merge Errors(w1200) -> (w1202:errorcluster)
            n567 = call <vilib>:"Add State(s) to Queue__jki_lib_state_machine.vi"("State(s) in (\"\")"=w1207) -> ("States Out"=w1206:string)  [unwired: 14 in]
          }
          frame "UI: Update AI Waveform Graphs Legends" {
            # "Do not put any code in this frame.\n(It is a separator no-op. You can make a copy of this frame to create a new UI frame)"
            n568 = Unbundle By Name(w1234) -> ("References.Graphs.PS WFGraph"=w1225:refnum<vi>, "References.Graphs.AI Graph"=w1227:refnum<vi>, "References.Graphs.Sweep AI Graph"=w1232:refnum<vi>, "UI Config.DAQ.Configuration"=w1231:T11)
            n569 = call "Get AI StringsAndValues.vi"("error in (no error)"=w1229, "Configuration.DAQ"=w1231) -> ("error out"=w1228:errorcluster, "AI StringsAndValues"=w1230:cluster{string, i32}[])  [unwired: 8 in]
            n570 = for {
              tunnel: w1232 -> [w1244]
              tunnel: w1230 -> [w1251] mode=indexing
              tunnel: w1228 -> [w1249]
              tunnel: w1227 -> [w1243]
              tunnel: [w1238] -> w1226 mode=indexing
              tunnel: w1225 -> [w1239]
              i -> [w1248]
              n571 = Unbundle(w1251) -> (w1250:string)  [unwired: 1 out]
              n572 = call-poly "Set Legend.vi"("error in (no error)"=w1249, "Plot.Plot Name"=w1250, "Active Plot"=w1248, "WFGraph in"=w1244) -> ("error out"=w1245:errorcluster, "Plot.Plot Name"=w1246:string, "Active Plot"=w1247:i32)  [unwired: 4 in, 1 out]
              n573 = call-poly "Set Legend.vi"("error in (no error)"=w1245, "Plot.Plot Name"=w1246, "Active Plot"=w1247, "WFGraph in"=w1243) -> ("error out"=w1242:errorcluster, "Plot.Plot Name"=w1241:string, "Active Plot"=w1240:i32)  [unwired: 4 in, 1 out]
              n574 = call-poly "Set Legend.vi"("error in (no error)"=w1242, "Plot.Plot Name"=w1241, "Active Plot"=w1240, "WFGraph (WDT) in"=w1239) -> ("error out"=w1238:errorcluster)  [unwired: 4 in, 3 out]
            }
            n575 = Merge Errors(w1226) -> (w1233:errorcluster)
            n576 = call <vilib>:"Add State(s) to Queue__jki_lib_state_machine.vi"("State(s) in (\"\")"=w1237) -> ("States Out"=w1236:string)  [unwired: 14 in]
          }
          frame "UI: Update AI Waveform Graphs Colors" {
            # "Do not put any code in this frame.\n(It is a separator no-op. You can make a copy of this frame to create a new UI frame)"
            n577 = Unbundle By Name(w1261) -> ("References.Graphs.PS WFGraph"=w1252:refnum<vi>, "References.Graphs.AI Graph"=w1254:refnum<vi>, "References.Graphs.Sweep AI Graph"=w1259:refnum<vi>, "UI Config.DAQ.Configuration"=w1258:T11)
            n578 = call "Get AI StringsAndValues.vi"("error in (no error)"=w1256, "Configuration.DAQ"=w1258) -> ("error out"=w1255:errorcluster, "AI StringsAndValues"=w1257:cluster{string, i32}[])  [unwired: 8 in]
            n579 = for {
              N -> [w1268]
              tunnel: w1259 -> [w1271]
              tunnel: w1257 -> [_] mode=indexing
              tunnel: w1255 -> [w1275]
              tunnel: w1254 -> [w1270]
              tunnel: [w1265] -> w1253 mode=indexing
              tunnel: w1252 -> [w1269]
              i -> [w1274]
              n580 = call-poly "Set Plot Color.vi"("Size (24)"=w1268, "error in (no error)"=w1275, "Active Plot"=w1274, "WFGraph in"=w1271) -> ("error out"=w1272:errorcluster, "Active Plot"=w1273:i32)  [unwired: 5 in, 1 out]
              n581 = call-poly "Set Plot Color.vi"("Size (24)"=w1268, "error in (no error)"=w1272, "Active Plot"=w1273, "WFGraph in"=w1270) -> ("error out"=w1266:errorcluster, "Active Plot"=w1267:i32)  [unwired: 5 in, 1 out]
              n582 = call-poly "Set Plot Color.vi"("Size (24)"=w1268, "error in (no error)"=w1266, "Active Plot"=w1267, "WFGraph (WDT) in"=w1269) -> ("error out"=w1265:errorcluster)  [unwired: 5 in, 2 out]
            }
            n583 = Merge Errors(w1253) -> (w1260:errorcluster)
            n584 = call <vilib>:"Add State(s) to Queue__jki_lib_state_machine.vi"("State(s) in (\"\")"=w1264) -> ("States Out"=w1263:string)  [unwired: 14 in]
          }
          frame "UI: Update AO Waveform Graphs Legends" {
            # "Do not put any code in this frame.\n(It is a separator no-op. You can make a copy of this frame to create a new UI frame)"
            n585 = Unbundle By Name(w1290) -> ("References.Graphs.AO Graph"=w1281:refnum<vi>, "References.Graphs.Sweep AO Graph"=w1288:refnum<vi>, "UI Config.DAQ.Configuration"=w1287:T11, "UI Config.Channels.Cfg_REF"=w1283:T7)
            n586 = call "Get AO StringsAndValues.vi"("error in (no error)"=w1285, "Configuration.DAQ"=w1287) -> ("error out"=w1282:errorcluster, "AO Strings and Values"=w1286:cluster{string, i32}[])  [unwired: 8 in]
            n587 = for {
              tunnel: w1288 -> [w1308]
              tunnel: w1286 -> [w1307] mode=indexing
              tunnel: w1282 -> [w1306]
              tunnel: [w1303] -> w1279
              i -> [w1304]
              n588 = Unbundle(w1307) -> (w1305:string)  [unwired: 1 out]
              n589 = call-poly "Set Legend.vi"("error in (no error)"=w1306, "Plot.Plot Name"=w1305, "Active Plot"=w1304, "WFGraph in"=w1308) -> ("error out"=w1303:errorcluster)  [unwired: 4 in, 3 out]
            }
            n590 = local read "Y Axis (Output)"() -> (w1284:enum16{"Analog Output", "Reference"})
            n591 = call "Get AI REF StringsAndValues.vi"("error in (no error)"=w1279, "Channels.REF"=w1283) -> ("error out"=w1278:errorcluster, "REF StringsAndValues"=w1277:cluster{string, i32}[])  [unwired: 8 in]
            n592 = case shown="\"Reference\"" w1284 {
              tunnel: [w1300 w1302] -> w1280
              tunnel: w1286 -> [w1300 _]
              tunnel: w1277 -> [_ w1301]
              frame "Analog Output", Default {
              }
              frame "Reference" {
                n593 = Interleave 1D Arrays(w1301, w1301) -> (w1302:cluster{string, i32}[])
              }
            }
            n594 = for {
              tunnel: w1281 -> [w1299]
              tunnel: w1280 -> [w1298] mode=indexing
              tunnel: w1278 -> [w1297]
              tunnel: [w1294] -> w1276 mode=indexing
              i -> [w1295]
              n595 = Unbundle(w1298) -> (w1296:string)  [unwired: 1 out]
              n596 = call-poly "Set Legend.vi"("error in (no error)"=w1297, "Plot.Plot Name"=w1296, "Active Plot"=w1295, "WFGraph in"=w1299) -> ("error out"=w1294:errorcluster)  [unwired: 4 in, 3 out]
            }
            n597 = Merge Errors(w1276) -> (w1289:errorcluster)
            n598 = call <vilib>:"Add State(s) to Queue__jki_lib_state_machine.vi"("State(s) in (\"\")"=w1293) -> ("States Out"=w1292:string)  [unwired: 14 in]
          }
          frame "UI: Update AO Waveform Graphs Colors" {
            # "Do not put any code in this frame.\n(It is a separator no-op. You can make a copy of this frame to create a new UI frame)"
            n599 = Unbundle By Name(w1323) -> ("References.Graphs.AO Graph"=w1314:refnum<vi>, "References.Graphs.Sweep AO Graph"=w1321:refnum<vi>, "UI Config.DAQ.Configuration"=w1320:T11, "UI Config.Channels.Cfg_REF"=w1316:T7)
            n600 = call "Get AO StringsAndValues.vi"("error in (no error)"=w1318, "Configuration.DAQ"=w1320) -> ("error out"=w1315:errorcluster, "AO Strings and Values"=w1319:cluster{string, i32}[])  [unwired: 8 in]
            n601 = for {
              N -> [w1335]
              tunnel: w1321 -> [w1339]
              tunnel: w1319 -> [_] mode=indexing
              tunnel: w1315 -> [w1338]
              tunnel: [w1336] -> w1312
              i -> [w1337]
              n602 = call-poly "Set Plot Color.vi"("Size (24)"=w1335, "error in (no error)"=w1338, "Active Plot"=w1337, "WFGraph in"=w1339) -> ("error out"=w1336:errorcluster)  [unwired: 5 in, 2 out]
            }
            n603 = local read "Y Axis (Output)"() -> (w1317:enum16{"Analog Output", "Reference"})
            n604 = call "Get AI REF StringsAndValues.vi"("error in (no error)"=w1312, "Channels.REF"=w1316) -> ("error out"=w1311:errorcluster, "REF StringsAndValues"=w1310:cluster{string, i32}[])  [unwired: 8 in]
            n605 = case shown="\"Reference\"" w1317 {
              tunnel: [w1332 w1334] -> w1313
              tunnel: w1319 -> [w1332 _]
              tunnel: w1310 -> [_ w1333]
              frame "Analog Output", Default {
              }
              frame "Reference" {
                n606 = Interleave 1D Arrays(w1333, w1333) -> (w1334:cluster{string, i32}[])
              }
            }
            n607 = for {
              N -> [w1327]
              tunnel: w1314 -> [w1331]
              tunnel: w1313 -> [_] mode=indexing
              tunnel: w1311 -> [w1330]
              tunnel: [w1328] -> w1309 mode=indexing
              i -> [w1329]
              n608 = call-poly "Set Plot Color.vi"("Size (24)"=w1327, "error in (no error)"=w1330, "Active Plot"=w1329, "WFGraph in"=w1331) -> ("error out"=w1328:errorcluster)  [unwired: 5 in, 2 out]
            }
            n609 = Merge Errors(w1309) -> (w1322:errorcluster)
            n610 = call <vilib>:"Add State(s) to Queue__jki_lib_state_machine.vi"("State(s) in (\"\")"=w1326) -> ("States Out"=w1325:string)  [unwired: 14 in]
          }
          frame "UI: Update Lockin Graphs Legends" {
            # "Do not put any code in this frame.\n(It is a separator no-op. You can make a copy of this frame to create a new UI frame)"
            n611 = Unbundle By Name(w1349) -> ("References.Graphs.Sweep X Graph"=w1348:refnum<vi>, "References.Graphs.Sweep Y Graph"=w1347:refnum<vi>, "References.Graphs.XY Graph"=w1346:refnum<vi>, "References.Graphs.Lockin 2"=w1345:refnum<vi>, "References.Graphs.Lockin 1"=w1344:refnum<vi>, "Plot Names"=w1342:string[])
            n612 = for {
              tunnel: w1344 -> [w1369]
              tunnel: w1345 -> [w1355]
              tunnel: [w1353] -> w1340 mode=indexing
              tunnel: w1341 -> [w1370]
              tunnel: w1346 -> [w1360]
              tunnel: w1347 -> [w1354]
              tunnel: w1348 -> [w1356]
              tunnel: w1342 -> [w1357] mode=indexing
              i -> [w1366]
              n613 = call-poly "Set Legend.vi"("error in (no error)"=w1370, "Plot.Plot Name"=w1357, "Active Plot"=w1366, "WaveformChart in"=w1369) -> ("error out"=w1367:errorcluster, "Plot.Plot Name"=w1362:string, "Active Plot"=w1368:i32)  [unwired: 4 in, 1 out]
              n614 = call-poly "Set Legend.vi"("error in (no error)"=w1367, "Plot.Plot Name"=w1362, "Active Plot"=w1368, "WaveformChart in"=w1355) -> ("error out"=w1363:errorcluster, "Active Plot"=w1359:i32)  [unwired: 4 in, 2 out]
              n615 = call-poly "Set Legend.vi"("error in (no error)"=w1363, "Plot.Plot Name"=w1362, "Active Plot"=w1359, "XYGraph in"=w1360) -> ("error out"=w1365:errorcluster, "Active Plot"=w1364:i32)  [unwired: 4 in, 2 out]
              n616 = call-poly "Set Legend.vi"("error in (no error)"=w1365, "Plot.Plot Name"=w1362, "Active Plot"=w1364, "WFGraph in"=w1354) -> ("error out"=w1361:errorcluster, "Active Plot"=w1358:i32)  [unwired: 4 in, 2 out]
              n617 = call-poly "Set Legend.vi"("error in (no error)"=w1361, "Plot.Plot Name"=w1362, "Active Plot"=w1358, "WFGraph in"=w1356) -> ("error out"=w1353:errorcluster)  [unwired: 4 in, 3 out]
            }
            n618 = Merge Errors(w1340) -> (w1343:errorcluster)
            n619 = call <vilib>:"Add State(s) to Queue__jki_lib_state_machine.vi"("State(s) in (\"\")"=w1352) -> ("States Out"=w1351:string)  [unwired: 14 in]
          }
          frame "UI: Update Lockin Graphs Colors" {
            # "Do not put any code in this frame.\n(It is a separator no-op. You can make a copy of this frame to create a new UI frame)"
            n620 = Unbundle By Name(w1380) -> ("References.Graphs.Sweep X Graph"=w1379:refnum<vi>, "References.Graphs.Sweep Y Graph"=w1378:refnum<vi>, "References.Graphs.XY Graph"=w1377:refnum<vi>, "References.Graphs.Lockin 2"=w1376:refnum<vi>, "References.Graphs.Lockin 1"=w1375:refnum<vi>, "Plot Names"=w1373:string[])
            n621 = for {
              N -> [w1384]
              tunnel: w1375 -> [w1399]
              tunnel: w1376 -> [w1387]
              tunnel: [w1385] -> w1371 mode=indexing
              tunnel: w1372 -> [w1400]
              tunnel: w1377 -> [w1391]
              tunnel: w1378 -> [w1386]
              tunnel: w1379 -> [w1388]
              tunnel: w1373 -> [_] mode=indexing
              i -> [w1396]
              n622 = call-poly "Set Plot Color.vi"("Size (24)"=w1384, "error in (no error)"=w1400, "Active Plot"=w1396, "WaveformChart in"=w1399) -> ("error out"=w1397:errorcluster, "Active Plot"=w1398:i32)  [unwired: 5 in, 1 out]
              n623 = call-poly "Set Plot Color.vi"("Size (24)"=w1384, "error in (no error)"=w1397, "Active Plot"=w1398, "WaveformChart in"=w1387) -> ("error out"=w1393:errorcluster, "Active Plot"=w1390:i32)  [unwired: 5 in, 1 out]
              n624 = call-poly "Set Plot Color.vi"("Size (24)"=w1384, "error in (no error)"=w1393, "Active Plot"=w1390, "XYGraph in"=w1391) -> ("error out"=w1395:errorcluster, "Active Plot"=w1394:i32)  [unwired: 5 in, 1 out]
              n625 = call-poly "Set Plot Color.vi"("Size (24)"=w1384, "error in (no error)"=w1395, "Active Plot"=w1394, "WFGraph in"=w1386) -> ("error out"=w1392:errorcluster, "Active Plot"=w1389:i32)  [unwired: 5 in, 1 out]
              n626 = call-poly "Set Plot Color.vi"("Size (24)"=w1384, "error in (no error)"=w1392, "Active Plot"=w1389, "WFGraph in"=w1388) -> ("error out"=w1385:errorcluster)  [unwired: 5 in, 2 out]
            }
            n627 = Merge Errors(w1371) -> (w1374:errorcluster)
            n628 = call <vilib>:"Add State(s) to Queue__jki_lib_state_machine.vi"("State(s) in (\"\")"=w1383) -> ("States Out"=w1382:string)  [unwired: 14 in]
          }
          frame "UI: Update Waveform Graphs" {
            w1405 = FALSE ("averaging")
            # "#todo\nshould be owned by Lockin UI"
            # "private"
            # "private"
            n629 = Unbundle By Name(w1414) -> ("UI Config.Amplifers.Gain_AI"=w1402:T9, "getAll.Waveforms.AI_wfm"=w1426:waveform(dbl)[], "getAll.Waveforms.AO_wfm"=w1420:waveform(dbl)[], "getAll.Waveforms.Ref_X_wfm"=w1417:waveform(dbl)[], "getAll.Waveforms.Ref_Y_wfm"=w1416:waveform(dbl)[])
            n630 = local read "Y Axis (Output)"() -> (w1413:enum16{"Analog Output", "Reference"})
            n631 = Interleave 1D Arrays(w1417, w1416) -> (w1415:waveform(dbl)[])
            n632 = for {
              tunnel: w1402 -> [w1432] mode=indexing
              tunnel: [w1431] -> w1401 mode=indexing
              n633 = Unbundle By Name(w1432) -> ("Gain"=w1431:dbl)
            }
            n634 = case shown="\"Analog Output\", Default" w1413 {
              tunnel: w1420 -> [w1433 _]
              tunnel: w1415 -> [_ w1434]
              tunnel: [w1433 w1434] -> w1419
              frame "Analog Output", Default {
              }
              frame "Reference" {
              }
            }
            n635 = local read "X Axis"() -> (w1412:enum16{"Time", "Samples"})
            n636 = local read "Decimate (UI)"() -> (w1411:enum16{"1", "10", "100", "1000"})
            n637 = call "Display n or dt.vi"("error in (no error)"=w1408, "X Axis"=w1412, "Input Waveforms"=w1426) -> ("error out"=w1425:errorcluster, "Output Waveforms"=w1418:waveform(dbl)[])  [unwired: 7 in]
            n638 = call "Display n or dt.vi"("error in (no error)"=w1408, "X Axis"=w1412, "Input Waveforms"=w1419) -> ("error out"=w1424:errorcluster, "Output Waveforms"=w1427:waveform(dbl)[])  [unwired: 7 in]
            n639 = Power Of 10(x=w1411) -> (10^x=w1421:dbl)
            n640 = local read "Y Axis (Input)"() -> (w1410:enum16{"Device", "ADC"})
            n641 = call "Decimate Waveforms.vi"("WFM"=w1427, "averaging"=w1405, "decimating factor"=w1421, "error in (no error)"=w1424) -> ("WFM out"=→"AO Graph":waveform(dbl)[], "error out"=w1406:errorcluster)  [unwired: 5 in]
            n642 = call "Decimate Waveforms.vi"("WFM"=w1418, "averaging"=w1405, "decimating factor"=w1421, "error in (no error)"=w1425) -> ("WFM out"=w1423:waveform(dbl)[], "error out"=w1422:errorcluster)  [unwired: 5 in]
            n643 = case shown="\"ADC\"" w1410 {
              tunnel: w1423 -> [w1436 w1441]
              tunnel: w1401 -> [_ w1439]
              tunnel: [w1436 w1440] -> w1404
              tunnel: w1422 -> [w1435 w1438]
              tunnel: [w1435 w1437] -> w1407
              frame "Device", Default {
              }
              frame "ADC" {
                n644 = call "Multiply by Gain.vi"("error in (no error)"=w1438, "Gain"=w1439, "WFM in"=w1441) -> ("error out"=w1437:errorcluster, "WFM out"=w1440:waveform(dbl)[])  [unwired: 7 in]
              }
            }
            "AI Graph" <- w1404
            n645 = Merge Errors(w1407, w1406) -> (w1409:errorcluster)
            n646 = call <vilib>:"Add State(s) to Queue__jki_lib_state_machine.vi"("State(s) in (\"\")"=w1430) -> ("States Out"=w1429:string)  [unwired: 14 in]
          }
          frame "UI: Update Waveform Graph Labels" {
            n647 = Unbundle By Name(w1450) -> ("References.Graphs.AO Graph"=w1445:refnum<vi>, "References.Graphs.AI Graph"=w1448:refnum<vi>)
            n648 = local read "Y Axis (Output)"() -> (w1447:enum16{"Analog Output", "Reference"})
            n649 = local read "X Axis"() -> (w1442:enum16{"Time", "Samples"})
            n650 = call "Set AO AI Graph X Axis (WFGraph).vi"("error in (no error)"=w1443, "X Axis"=w1442, "WaveformGraph in"=w1448) -> ("error out"=w1449:errorcluster)  [unwired: 8 in]
            n651 = call "Set AO AI Graph X Axis (WFGraph).vi"("error in (no error)"=w1449, "X Axis"=w1442, "WaveformGraph in"=w1445) -> ("error out"=w1446:errorcluster)  [unwired: 8 in]
            n652 = call "Set AO Graph Y Axis (WFGraph).vi"("error in (no error)"=w1446, "Y Axis (Output)"=w1447, "WaveformGraph in"=w1445) -> ("error out"=w1444:errorcluster)  [unwired: 8 in]
            n653 = call <vilib>:"Add State(s) to Queue__jki_lib_state_machine.vi"("State(s) in (\"\")"=w1453) -> ("States Out"=w1452:string)  [unwired: 14 in]
          }
          frame "UI: Initialize Lockin Charts" {
            # "Do not put any code in this frame.\n(It is a separator no-op. You can make a copy of this frame to create a new UI frame)"
            n654 = Unbundle By Name(w1457) -> ("References.Graphs.Lockin 1"=w1455:refnum<vi>, "References.Graphs.Lockin 2"=w1456:refnum<vi>)
            n655 = Build Array(w1455, w1456) -> (w1454:refnum<vi>[])
            n656 = for {
              tunnel: w1454 -> [w1462] mode=indexing
              n657 = property on="Property Node" class="WFChart (strict)"(reference=w1462, "History Data"=waveform(dbl)[][] []) -> ()  [unwired: 1 in, 2 out]
            }
            n658 = call <vilib>:"Add State(s) to Queue__jki_lib_state_machine.vi"("State(s) in (\"\")"=w1461) -> ("States Out"=w1460:string)  [unwired: 14 in]
          }
          frame "UI: Update Lockin Graphs" {
            n659 = Unbundle By Name(w1485) -> ("getAll.Results.Results (Dictionary)"=w1476:cluster{"key":string, "value":dbl}[], "UI Config.DAQ.Configuration"=w1475:T11, "UI Config.Amplifers.Gain_AI"=w1474:T9)
            n660 = call "Parse Results (table).vi"("error in (no error)"=w1484, "Input Gain"=w1474, "DAQ Config"=w1475, "Results (Dictionary)"=w1476) -> ("error out"=w1482:errorcluster, "Table"=→"Results":string[][], "Results (Dictionary) out"=w1480:cluster{"key":string, "value":dbl}[])  [unwired: 5 in]
            n661 = local read "Display"() -> (w1472:T25)
            n662 = call "Dictionary to Chart.vi"("error in (no error)"=w1482, "Display"=w1472, "Results (Dictionary)"=w1480) -> ("error out"=w1473:errorcluster, "Y/Theta Array"=→"Lockin 2":waveform(dbl)[], "X/R Array"=→"Lockin 1":waveform(dbl)[], "Results (Dictionary) out"=w1478:cluster{"key":string, "value":dbl}[])  [unwired: 5 in]
            n663 = call "Dictionary to XY Graph.vi"("error in (no error)"=w1473, "Results (Dictionary)"=w1478) -> ("error out"=w1470:errorcluster, "XY Graph"=→"XY Graph":cluster{dbl[], dbl[]}[], "Results (Dictionary) out"=w1471:cluster{"key":string, "value":dbl}[])  [unwired: 7 in]
            n664 = local read "Channel"() -> (w1477:i32)
            n665 = call "Dictionary to Indicator.vi"("Results (Dictionary)"=w1471, "AI Channel"=w1477, "error in (no error)"=w1470) -> ("X"=→"X":dbl, "Y"=→"Y":dbl, "R"=→"R":dbl, "Theta"=→"Theta":dbl, "error out"=w1483:errorcluster)  [unwired: 8 in]
            n666 = call <vilib>:"Add State(s) to Queue__jki_lib_state_machine.vi"("State(s) in (\"\")"=w1488) -> ("States Out"=w1487:string)  [unwired: 14 in]
          }
          frame "UI: Update Lockin Graph Range" {
            # "xy"
            # "2"
            # "1"
            # "Do not put any code in this frame.\n(It is a separator no-op. You can make a copy of this frame to create a new UI frame)"
            n667 = Unbundle By Name(w1496) -> ("References.Graphs.Lockin 1"=w1493:refnum<vi>, "References.Graphs.Lockin 2"=w1492:refnum<vi>, "References.Graphs.XY Graph"=w1491:refnum<vi>)
            n668 = Negate(x="X/R Range") -> (-x=w1497:dbl)
            n669 = Negate(x="Y/Theta Range") -> (-x=w1498:dbl)
            n670 = Negate(x="XY Range") -> (-x=w1490:dbl)
            n671 = property on="Property Node" class="WFChart (strict)"(reference=w1493, "YScale.Maximum"="X/R Range", "YScale.Minimum"=w1497) -> ()  [unwired: 1 in, 2 out]
            n672 = property on="Property Node" class="WFChart (strict)"(reference=w1492, "YScale.Maximum"="Y/Theta Range", "YScale.Minimum"=w1498) -> ()  [unwired: 1 in, 2 out]
            n673 = property on="Property Node" class="XYGraph (strict)"(reference=w1491, "XScale.Maximum"="XY Range", "YScale.Maximum"="XY Range", "XScale.Minimum"=w1490, "YScale.Minimum"=w1490) -> ()  [unwired: 1 in, 2 out]
            n674 = call <vilib>:"Add State(s) to Queue__jki_lib_state_machine.vi"("State(s) in (\"\")"=w1502) -> ("States Out"=w1501:string)  [unwired: 14 in]
          }
          frame "UI: Update Lockin Graph Labels" {
            n675 = local read "Display"() -> (w1508:T25)
            n676 = Unbundle By Name(w1505) -> ("References.Graphs.Lockin 1"=w1504:refnum<vi>, "References.Graphs.Lockin 2"=w1503:refnum<vi>)
            n677 = case shown="\"X and Y\", Default" w1508 {
              tunnel: ["Lockin X (V)" "R (V)"] -> w1507
              tunnel: ["Lockin Y (V)" "Theta (°)"] -> w1506
              frame "X and Y", Default {
              }
              frame "R and Theta" {
              }
            }
            n678 = property on="Property Node" class="WFChart (strict)"(reference=w1504, "YScale.NameLbl.Text"=w1507) -> ()  [unwired: 1 in, 2 out]
            n679 = property on="Property Node" class="WFChart (strict)"(reference=w1503, "YScale.NameLbl.Text"=w1506) -> ()  [unwired: 1 in, 2 out]
            n680 = call <vilib>:"Add State(s) to Queue__jki_lib_state_machine.vi"("State(s) in (\"\")"=w1512) -> ("States Out"=w1511:string)  [unwired: 14 in]
          }
          frame "UI: Initialize PS Graph" {
            # "Do not put any code in this frame.\n(It is a separator no-op. You can make a copy of this frame to create a new UI frame)"
            n681 = Unbundle By Name(w1528) -> ("References.Graphs.PS Chart"=w1522:refnum<vi>, "References.Graphs.PS WFGraph"=w1527:refnum<vi>, "UI Config.Plot.visibility.AI"=w1525:bool[])
            n682 = Array Size(array=w1525) -> (size(s)=w1520:i32)
            n683 = Initialize Array(cluster{"f0":dbl, "df":dbl, "magnitude":dbl[]} {"f0"=0.0, "df"=1.0, "magnitude"=[0.001]} ("power spectrum"), w1520) -> (w1523:cluster{"f0":dbl, "df":dbl, "magnitude":dbl[]}[])
            n684 = Initialize Array(0.0 ("df"), w1520) -> (w1517:dbl[])
            n685 = property on="Property Node" class="WFGraph (strict)"(reference=w1527, error in=w1524, "Value"=w1523) -> (error out=w1521:errorcluster)  [unwired: 1 out]
            n686 = local write "PS WFGraph"(w1523) -> ()
            n687 = Build Array(w1517) -> (w1518:dbl[][])
            n688 = property on="Property Node" class="WFChart (strict)"(reference=w1522, error in=w1521, "History Data"=w1518) -> ()  [unwired: 2 out]
            n689 = call <vilib>:"Add State(s) to Queue__jki_lib_state_machine.vi"("State(s) in (\"\")"=w1531) -> ("States Out"=w1530:string)  [unwired: 14 in]
          }
          frame "UI: Update Sweep Graphs" {
            # "Do not put any code in this frame.\n(It is a separator no-op. You can make a copy of this frame to create a new UI frame)"
            n690 = Unbundle By Name(w1536) -> ("getAll.Waveforms.AO_wfm"=→"Sweep AO":waveform(dbl)[], "getAll.Waveforms.AI_wfm"=→"Sweep AI":waveform(dbl)[], "getAll.Waveforms.X_wfm"=→"Sweep Results X":waveform(dbl)[], "getAll.Waveforms.Y_wfm"=→"Sweep Results Y":waveform(dbl)[])
            n691 = call <vilib>:"Add State(s) to Queue__jki_lib_state_machine.vi"("State(s) in (\"\")"=w1540) -> ("States Out"=w1539:string)  [unwired: 14 in]
          }
          frame "UI: Update Sweep Timer" {
            # "Do not put any code in this frame.\n(It is a separator no-op. You can make a copy of this frame to create a new UI frame)"
            n692 = local read "Sweep Time (s)"() -> (w1544:dbl)
            n693 = local read "Initial Wait (s)"() -> (w1543:dbl)
            n694 = Unbundle By Name(w1542) -> ("DAQ state"=w1541:T22)
            n695 = case shown="Default" w1541 {
              tunnel: [0.0 w1554] -> w1545
              tunnel: w1544 -> [_ w1552]
              tunnel: w1543 -> [_ w1551]
              frame Default {
              }
              frame "sweeping" {
                # "some overhead"
                n696 = call <userlib>:"MGI Milliseconds Since Last Reset.vi"() -> ("ms"=w1558:u32)  [unwired: 6 in, 1 out]
                n697 = Divide(x=w1558, y=u32 1000) -> (x/y=w1556:dbl)
                n698 = Negate(x=w1556) -> (-x=w1555:dbl)
                n699 = Compound Arithmetic op=ADD(2.0 ("value"), w1551, w1552, w1555) -> (w1554:dbl)
              }
            }
            n700 = local write "Sweep Timer (s)"(w1545) -> ()
            n701 = call <vilib>:"Add State(s) to Queue__jki_lib_state_machine.vi"("State(s) in (\"\")"=w1549) -> ("States Out"=w1548:string)  [unwired: 14 in]
          }
          frame "UI: Update Sweep Config" {
            # "UI: Update Sweep Config\n(Called by <DAQ Public Events.getSweepChannels>: User Event)"
            n702 = Unbundle By Name(w1565) -> ("UI Config.Sweep"=w1561:T54)
            n703 = Unbundle By Name(w1561) -> ("Sweep Time (s)"=w1563:dbl, "Initial Wait (s)"=w1564:dbl, "Return to Start"=w1562:bool, "Channels"=w1559:T18)
            n704 = for {
              tunnel: w1559 -> [w1573] mode=indexing
              tunnel: [w1570] -> w1560 mode=indexing
              n705 = Unbundle By Name(w1573) -> ("Channel"=w1572:u16, "Table"=w1571:dbl[])
              n706 = Bundle("Channel"=w1572, "Table"=w1571) -> (w1570:cluster{"Channel":u16, "Table":dbl[]})  [unwired: 1 in]
            }
            n707 = local write "Sweep Time (s)"(w1563) -> ()
            n708 = local write "Initial Wait (s)"(w1564) -> ()
            n709 = local write "Return to Start?"(w1562) -> ()
            n710 = local write "Sweep Channels"(w1559) -> ()
            n711 = local write "Sweep Pattern"(w1560) -> ()
            n712 = call <vilib>:"Add State(s) to Queue__jki_lib_state_machine.vi"("State(s) in (\"\")"=w1569) -> ("States Out"=w1568:string)  [unwired: 14 in]
          }
          frame "UI: Update Channel Ring" {
            # "Do not put any code in this frame.\n(It is a separator no-op. You can make a copy of this frame to create a new UI frame)"
            n713 = Unbundle By Name(w1576) -> ("Plot Names"=w1575:string[])
            n714 = property on="Channel" class="Ring (strict)"(error in=w1577, "Strings []"=w1575) -> (error out=w1574:errorcluster)  [unwired: 1 in, 1 out]
            n715 = call <vilib>:"Add State(s) to Queue__jki_lib_state_machine.vi"("State(s) in (\"\")"=w1580) -> ("States Out"=w1579:string)  [unwired: 14 in]
          }
          frame "UI: Update AI REF Channel Ring" {
            # "update AI Ref Channel ring"
            # "Do not put any code in this frame.\n(It is a separator no-op. You can make a copy of this frame to create a new UI frame)"
            n716 = Unbundle By Name(w1584) -> ("UI Config.Channels.Cfg_REF"=w1583:T7)
            n717 = call "Get REF StringsAndValues.vi"("error in (no error)"=w1582, "Channels.REF"=w1583) -> ("error out"=w1586:errorcluster, "REF Strings and Values"=w1585:cluster{string, i32}[])  [unwired: 8 in]
            n718 = property on="Reference" class="Ring (strict)"(error in=w1586, "StringsAndValues[]"=w1585) -> (error out=w1581:errorcluster)  [unwired: 1 in, 1 out]
            n719 = call <vilib>:"Add State(s) to Queue__jki_lib_state_machine.vi"("State(s) in (\"\")"=w1589) -> ("States Out"=w1588:string)  [unwired: 14 in]
          }
          frame "UI: Remove Unused References" {
            # "update Ch.AI after removing\nunused Ch.REF"
            # "Do not put any code in this frame.\n(It is a separator no-op. You can make a copy of this frame to create a new UI frame)"
            n720 = Unbundle By Name(w1595) -> ("UI Config.Channels.Cfg_AI"=w1594:T2, "UI Config.Channels.Cfg_REF"=w1593:T7)
            n721 = call "Remove Unused References.vi"("error in (no error)"=w1591, "Channels.REF"=w1593, "Channels.AI"=w1594) -> ("error out"=w1592:errorcluster, "Channels.AI out"=w1590:T2)  [unwired: 7 in]
            n722 = local write "AI Channels"(w1590) -> ()
            n723 = call <vilib>:"Add State(s) to Queue__jki_lib_state_machine.vi"("State(s) in (\"\")"=w1598) -> ("States Out"=w1597:string)  [unwired: 14 in]
          }
          frame "UI: Update AI REF Channels" {
            # "Do not put any code in this frame.\n(It is a separator no-op. You can make a copy of this frame to create a new UI frame)"
            n724 = Unbundle By Name(w1601) -> ("UI Config.Channels.Cfg_AI"=w1604:T2)
            n725 = case shown="\"Disable\", Default" w1600 {
              tunnel: [u16[] [1] ("References") u32[] [0] ("References")] -> w1603
              frame "All 1" {
              }
              frame "Disable", Default {
              }
            }
            n726 = for {
              tunnel: w1604 -> [w1613] mode=indexing
              tunnel: [w1612] -> w1599 mode=indexing
              tunnel: w1603 -> [w1611]
              n727 = Bundle By Name(cluster=w1613, "References"=w1611) -> (w1612:T3)
            }
            n728 = Bundle By Name(cluster=w1601, "UI Config.Channels.Cfg_AI"=w1599) -> (w1602:T63)
            n729 = local write "AI Channels"(w1599) -> ()
            n730 = call <vilib>:"Add State(s) to Queue__jki_lib_state_machine.vi"("State(s) in (\"\")"=w1608) -> ("States Out"=w1607:string)  [unwired: 14 in]
          }
          frame "UI: Cursor Set" {
            # "Argument"
            # "Initialize the User Interface, here.\n(this is called automatically, by the Macro: Init)"
            n731 = disable-structure shown="Default" {
              disable-tunnel: w1616 -> [w1621 w1624]
              disable-tunnel: [w1621 w1623] -> w1615
              disable-tunnel: w1614 -> [_ w1622]
              frame condition #0 {
              }
              frame condition #1 (active) {
                n732 = case shown="\"Idle\", Default" w1622 {
                  tunnel: w1624 -> [w1626 w1628]
                  tunnel: [w1625 w1627] -> w1623
                  frame "Idle", Default {
                    n733 = call <vilib>:"Unset Busy.vi"("error in (no error)"=w1626) -> ("error out"=w1625:errorcluster)  [unwired: 10 in]
                  }
                  frame "Busy" {
                    n734 = call <vilib>:"Set Busy.vi"("error in (no error)"=w1628) -> ("error out"=w1627:errorcluster)  [unwired: 9 in, 1 out]
                  }
                }
              }
            }
            n735 = call <vilib>:"Add State(s) to Queue__jki_lib_state_machine.vi"("State(s) in (\"\")"=w1620) -> ("States Out"=w1619:string)  [unwired: 14 in]
          }
          frame "UI: Defer Panel Updates" {
            # "Do not put any code in this frame.\n(It is a separator no-op. You can make a copy of this frame to create a new UI frame)"
            n736 = Unbundle By Name(w1633) -> ("Front Panel"=w1632:refnum<vi>)
            n737 = Scan From String(input string=w1630, default 1=FALSE) -> (output 1=w1631:bool)  [unwired: 3 in, 3 out]
            n738 = property class="Pnl"(reference=w1632, "Defer Panel Updates"=w1631) -> ()  [unwired: 1 in, 2 out]
            n739 = call <vilib>:"Add State(s) to Queue__jki_lib_state_machine.vi"("State(s) in (\"\")"=w1637) -> ("States Out"=w1636:string)  [unwired: 14 in]
          }
          frame "UI: Front Panel State" {
            # "Argument"
            # "Set Front Panel Open or Closed\n(Usage: \"UI: Front Panel State >> Open|Close\")"
            n740 = Unbundle By Name(w1641) -> ("Core.Current VI Reference"=w1640:refnum<vi>)
            n741 = disable-structure shown="Default" {
              disable-tunnel: w1643 -> [w1649 w1672]
              disable-tunnel: [w1648 w1672] -> w1642
              disable-tunnel: w1640 -> [w1647 _]
              disable-tunnel: w1639 -> [w1646 _]
              frame condition #0 (active) {
                n742 = case shown="\"Close\"" w1646 {
                  tunnel: w1649 -> [w1653 w1666]
                  tunnel: [w1655 w1667] -> w1648
                  tunnel: w1647 -> [w1654 w1664]
                  frame "Open", Default {
                    n743 = property class="VI"(reference=w1654, error in=w1653) -> (reference out=w1651:refnum<vi>, error out=w1652:errorcluster, "FP.State"=w1650:T37)
                    n744 = case shown="\"Closed\"" w1650 {
                      tunnel: [w1658 w1661] -> w1655
                      tunnel: w1652 -> [w1657 w1661]
                      tunnel: w1651 -> [w1656 _]
                      frame "Closed" {
                        n745 = invoke class="VI" method="FP.Open"(reference=w1656, error in=w1657, "Activate"=TRUE, "State"=T37."Standard") -> (error out=w1658:errorcluster)  [unwired: 1 in, 4 out]
                      }
                      frame Default {
                      }
                    }
                  }
                  frame "Close" {
                    n746 = property class="VI"(reference=w1664, error in=w1666) -> (reference out=w1663:refnum<vi>, error out=w1665:errorcluster, "FP.State"=w1662:T37)
                    n747 = case shown="Default" w1662 {
                      tunnel: [w1668 w1671] -> w1667
                      tunnel: w1665 -> [w1668 w1670]
                      tunnel: w1663 -> [_ w1669]
                      frame "Invalid", "Closed" {
                      }
                      frame Default {
                        n748 = invoke class="VI" method="FP.Close"(reference=w1669, error in=w1670) -> (error out=w1671:errorcluster)  [unwired: 1 in, 2 out]
                      }
                    }
                  }
                }
              }
              frame condition #1 {
              }
            }
            n749 = call <vilib>:"Add State(s) to Queue__jki_lib_state_machine.vi"("State(s) in (\"\")"=w1645) -> ("States Out"=w1644:string)  [unwired: 14 in]
          }
          frame "---------- Macro ----------" {
            # "Do not put any code in this frame.\n(It is a separator no-op. You can make a copy of this frame to create a new Macro frame)"
            n750 = call <vilib>:"Add State(s) to Queue__jki_lib_state_machine.vi"("State(s) in (\"\")"=w1677) -> ("States Out"=w1676:string)  [unwired: 14 in]
          }
          frame "Macro: Initialize" {
            # "Initialization Macro\n(This is called once, when the VI starts)"
            n751 = call <vilib>:"Add State(s) to Queue__jki_lib_state_machine.vi"("State(s) in Front (\"\")"="Data: Initialize\nInitialize Core Data\nEvents: Register", "State(s) in (\"\")"="") -> ("States Out"=w1678:string)  [unwired: 13 in]
            n752 = call <vilib>:"Add State(s) to Queue__jki_lib_state_machine.vi"("State(s) in Front (\"\")"=w1678, "State(s) in (\"\")"="Process: Sync", "State(s) at Back (\"\")"="UI: Initialize\nMacro: Initialize UI Before Open\nUI: Front Panel State >> Open\nMacro: Initialize UI After Open\nData: Wait >> 500\nMacro: Initialize III") -> ("States Out"=w1682:string)  [unwired: 12 in]
            n753 = call <vilib>:"Add State(s) to Queue__jki_lib_state_machine.vi"("State(s) in Front (\"\")"=w1682, "State(s) in (\"\")"=w1688) -> ("States Out"=w1687:string)  [unwired: 13 in]
          }
          frame "Macro: Post Error Handling" {
            # "Clear Last Error?"
            # "Do not put any code in this frame.\n(It is a separator no-op. You can make a copy of this frame to create a new Macro frame)"
            n754 = Unbundle By Name(w1690) -> ("Core.Last Error.remaining states"=w1692:string, "Core.Shutdown?"=w1693:bool)
            n755 = Unbundle By Name(w1690) -> ("Core.Last Error.error"=w1696:errorcluster)
            n756 = case shown="False" FALSE {
              tunnel: w1696 -> [w1704 _]
              tunnel: [w1704 _] -> w1695
              frame False {
              }
              frame True {
              }
            }
            n757 = case shown="True" w1693 {
              tunnel: w1692 -> [w1701 w1703]
              tunnel: [w1701 w1702] -> w1689
              frame False {
                # "These are the remaining states (at the moment the error occured). States can be altered according to business logic."
                # "NOT SHUTTING DOWN"
              }
              frame True {
                # "Developer can decide to alter the states but should be aware that during the shutdown process, there are certain states that must be run for the SMO to properly shut itself (and this process) down. As such, one can add states to perform additional clean-ups, but should append the remaining state to be executed."
                # "SHUTTING DOWN"
                n758 = call <vilib>:"Add State(s) to Queue__jki_lib_state_machine.vi"("State(s) in (\"\")"=w1703) -> ("States Out"=w1702:string)  [unwired: 14 in]
              }
            }
            n759 = Bundle By Name(cluster=w1690, "Core.Last Error.error"=w1695) -> (w1691:T63)
            n760 = call <vilib>:"Add State(s) to Queue__jki_lib_state_machine.vi"("State(s) in Front (\"\")"=w1689, "State(s) in (\"\")"=w1700) -> ("States Out"=w1699:string)  [unwired: 13 in]
          }
          frame "Macro: Initialize UI Before Open" {
            # "Initialize UI\n(This is called after UI: Initialize and before UI: Front Panel State >> Open)"
            n761 = local write "Show UI"(FALSE ("Show UI")) -> ()
            n762 = call <vilib>:"Add State(s) to Queue__jki_lib_state_machine.vi"("State(s) in Front (\"\")"="UI: Cursor Set >> Busy\n\nData: Initialize Control References\nData: Initialize Graph References\n\nUI: Reinit To Default\nUI: Disable Buttons\n\nConfiguration: Initialize\nConfiguration: Read File\nUI: Cluster to UI" ("State(s) in Front (\"\")"), "State(s) in (\"\")"=w1711) -> ("States Out"=w1710:string)  [unwired: 13 in]
          }
          frame "Macro: Initialize UI After Open" {
            w1712 = T26."AO/AI"  # Right Tab
            w1713 = T1."Status"  # Left Tab
            # "Initialize UI\n(This is called after UI: Initialize and before UI: Front Panel State >> Open)"
            n763 = Format Into String(format string="UI: Set Left Tab >> %s\nUI: Set Right Tab >> %s\n\nUI: Cursor Set >> Idle" ("State(s) in Front (\"\")"), w1713, w1712) -> (resulting string=w1714:string)  [unwired: 2 in, 1 out]
            n764 = call <vilib>:"Add State(s) to Queue__jki_lib_state_machine.vi"("State(s) in Front (\"\")"=w1714, "State(s) in (\"\")"=w1720) -> ("States Out"=w1719:string)  [unwired: 13 in]
          }
          frame "Macro: Initialize III" {
            w1721 = T26."AO/AI"  # Right Tab
            w1722 = T1."AO/AI/REF"  # Left Tab
            # "Initialize UI\n(This is called after UI: Initialize and before UI: Front Panel State >> Open)"
            n765 = Format Into String(format string="UI: Cursor Set >> Busy\n\nMacro: Initialize DAQ\nIdle\nMacro: Initialize Graphs\nIdle\nUI: Enable Buttons\n\nUI: Set Left Tab >> %s\nUI: Set Right Tab >> %s\n\nUI: Cursor Set >> Idle" ("State(s) in Front (\"\")"), w1722, w1721) -> (resulting string=w1723:string)  [unwired: 2 in, 1 out]
            n766 = call <vilib>:"Add State(s) to Queue__jki_lib_state_machine.vi"("State(s) in Front (\"\")"=w1723, "State(s) in (\"\")"=w1729) -> ("States Out"=w1728:string)  [unwired: 13 in]
          }
          frame "Macro: Initialize DAQ" {
            # "//Action: Offset"
            # "Do not put any code in this frame.\n(It is a separator no-op. You can make a copy of this frame to create a new Data frame)"
            n767 = call <vilib>:"Delimited String to 1D String Array.vi"("delimiter"="\n", "delimited string"="Action: DAQ Config\nAction: Sampling\nAction: Sampling Fs Mode\nAction: Sampling Fs Multiplier\nAction: Sampling Fs Output\nAction: Sampling Refresh Rate\nAction: Sampling Decimation Pre DSP\nAction: Sampling Decimation Post DSP\nAction: AI Simulate Mode\nAction: AI Channels\nAction: AO Channels\nAction: REF Channels\nAction: Sweep\nAction: Limit Amplitude\nAction: Link Frequencies\nAction: PreFilter\nAction: Offset Mode >> Remove\nAction: Input Gain\nAction: Output Gain\nAction: State >> reset" ("State(s) in Front (\"\")")) -> ("string array"=w1733:string[])  [unwired: 9 in]
            n768 = Array Size(array=w1733) -> (size(s)=w1737:i32)
            n769 = Initialize Array("Action: Command\nData: Wait >> 25\n//Idle", w1737) -> (w1736:string[])
            n770 = Interleave 1D Arrays(w1733, w1736) -> (w1735:string[])
            n771 = call <vilib>:"1D String Array to Delimited String.vi"("delimiter"="\n", "string array"=w1735) -> ("delimited string"=w1734:string)  [unwired: 9 in]
            n772 = call <vilib>:"Add State(s) to Queue__jki_lib_state_machine.vi"("State(s) in Front (\"\")"=w1734, "State(s) in (\"\")"=w1743) -> ("States Out"=w1742:string)  [unwired: 13 in]
          }
          frame "Macro: Initialize Graphs" {
            # "Do not put any code in this frame.\n(It is a separator no-op. You can make a copy of this frame to create a new Macro frame)"
            n773 = Unbundle By Name(w1747) -> ("getAll.Results.Results (Dictionary)"=w1744:cluster{"key":string, "value":dbl}[])
            n774 = call "Dictionary to Plot Names.vi"("error in (no error)"=w1746, "Results (Dictionary)"=w1744) -> ("error out"=w1745:errorcluster, "Plot Names"=w1748:string[])  [unwired: 7 in, 1 out]
            n775 = Bundle By Name(cluster=w1747, "Plot Names"=w1748) -> (w1749:T63)
            n776 = call <vilib>:"Add State(s) to Queue__jki_lib_state_machine.vi"("State(s) in Front (\"\")"="UI: Defer Panel Updates >> TRUE\nUI: Initialize Lockin Charts\nUI: Update Waveform Graphs\nUI: Update Lockin Graphs\nUI: Update Sweep Graphs\nUI: Initialize PS Graph\n\nUI: Update Channel Ring\nUI: Update AI REF Channel Ring\n\nUI: Update AI Waveform Graphs Legends\nUI: Update AI Waveform Graphs Colors\nUI: Update AO Waveform Graphs Legends\nUI: Update AO Waveform Graphs Colors\nUI: Update Lockin Graphs Legends\nUI: Update Lockin Graphs Colors\n\nUI: Set Plot Visibility //from UI cluster\nUI: Sync AI Plot Visibility\nUI: Sync AO Plot Visibility\nUI: Sync Lockin Plot Visibility\nUI: Defer Panel Updates >> FALSE" ("State(s) in Front (\"\")"), "State(s) in (\"\")"=w1753) -> ("States Out"=w1752:string)  [unwired: 13 in]
          }
          frame "Macro: Update Graphs" {
            # "Do not put any code in this frame.\n(It is a separator no-op. You can make a copy of this frame to create a new Macro frame)"
            n777 = Unbundle By Name(w1759) -> ("Plot Names"=w1766:string[], "getAll.Results.Results (Dictionary)"=w1769:cluster{"key":string, "value":dbl}[])
            n778 = local read "Right Tab"() -> (w1771:T26)
            n779 = call "Dictionary to Plot Names.vi"("error in (no error)"=w1767, "Results (Dictionary)"=w1769) -> ("error out"=w1768:errorcluster, "Plot Names"=w1758:string[])  [unwired: 7 in, 1 out]
            n780 = Not Equal?(x=w1766, y=w1758) -> (x != y?=w1764:bool)
            n781 = case shown="\"PS\"" w1771 {
              tunnel: ["UI: Update Waveform Graphs" ("State(s) in Front (\"\")") "Action: Power Spectrum" ("State(s) in Front (\"\")") "" ("State(s) in Front (\"\")")] -> w1770
              frame "AO/AI" {
              }
              frame "PS" {
              }
              frame Default {
              }
            }
            n782 = Select(t="UI: Update Channel Ring\nUI: Update Lockin Graphs Legends\nUI: Update Lockin Graphs Colors" ("State(s) in Front (\"\")"), s=w1764, f="") -> (s? t:f=w1761:string)
            n783 = Bundle By Name(cluster=w1759, "Plot Names"=w1758) -> (w1760:T63)
            n784 = call <vilib>:"Add State(s) to Queue__jki_lib_state_machine.vi"("State(s) in Front (\"\")"=w1770, "State(s) in (\"\")"=w1761, "State(s) at Back (\"\")"="UI: Update Lockin Graphs" ("State(s) in Front (\"\")")) -> ("States Out"=w1757:string)  [unwired: 12 in]
            n785 = call <vilib>:"Add State(s) to Queue__jki_lib_state_machine.vi"("State(s) in Front (\"\")"="UI: Defer Panel Updates >> TRUE" ("State(s) in Front (\"\")"), "State(s) in (\"\")"=w1757, "State(s) at Back (\"\")"="UI: Defer Panel Updates >> FALSE" ("State(s) in Front (\"\")")) -> ("States Out"=w1754:string)  [unwired: 12 in]
            n786 = call <vilib>:"Add State(s) to Queue__jki_lib_state_machine.vi"("State(s) in Front (\"\")"=w1754, "State(s) in (\"\")"=w1774) -> ("States Out"=w1773:string)  [unwired: 13 in]
          }
          frame "Macro: Save Configuration" {
            # "Do not put any code in this frame.\n(It is a separator no-op. You can make a copy of this frame to create a new Macro frame)"
            n787 = call <vilib>:"Add State(s) to Queue__jki_lib_state_machine.vi"("State(s) in Front (\"\")"="UI: Get Plot Visibility\nUI: UI to Cluster\nConfiguration: Write File", "State(s) in (\"\")"=w1783) -> ("States Out"=w1782:string)  [unwired: 13 in]
          }
          frame "Macro: Exit" {
            # "Exit Macro\n(This is called once, when the VI exits)"
            n788 = Unbundle By Name(w1786) -> ("Core.Close Panel on Exit?"=w1797:bool)
            n789 = Bundle By Name(cluster=w1786, "Core.Shutdown?"=TRUE) -> (w1787:T63)
            n790 = Select(t="UI: Front Panel State >> Open", s=w1797, f="") -> (s? t:f=w1784:string)
            n791 = call <vilib>:"Add State(s) to Queue__jki_lib_state_machine.vi"("State(s) in Front (\"\")"="Data: Cleanup\nEvents: Unregister\nProcess: Self Terminate", "State(s) in (\"\")"="Process: Sync", "State(s) at Back (\"\")"="Exit") -> ("States Out"=w1785:string)  [unwired: 12 in]
            n792 = call <vilib>:"Add State(s) to Queue__jki_lib_state_machine.vi"("State(s) in Front (\"\")"="Macro: Save Configuration", "State(s) in (\"\")"=w1784, "State(s) at Back (\"\")"=w1785) -> ("States Out"=w1794:string)  [unwired: 12 in]
            n793 = call <vilib>:"Add State(s) to Queue__jki_lib_state_machine.vi"("State(s) in Front (\"\")"=w1794, "State(s) in (\"\")"=w1800) -> ("States Out"=w1799:string)  [unwired: 13 in]
          }
          frame "---------- Process ----------" {
            # "Template Separator\n(You can make a copy of, or modify, this frame)"
            n794 = call <vilib>:"Add State(s) to Queue__jki_lib_state_machine.vi"("State(s) in (\"\")"=w1805) -> ("States Out"=w1804:string)  [unwired: 14 in]
          }
          frame "Process: Sync" {
            n795 = Unbundle By Name(w1813) -> ("SelfRef"=w1809:refnum<class "Instrument UI.Lockin.lvclass">)
            n796 = call <vilib>:"WaitOnProcessSync.vi"("error in (no error)"=w1808, "SMO"=w1809) -> ("error out"=w1807:errorcluster, "Don't run?"=w1812:bool)  [unwired: 7 in, 1 out]
            n797 = Select(t="Data: Cleanup\nEvents: Unregister\nExit", s=w1812, f="") -> (s? t:f=w1806:string)
            n798 = call <vilib>:"Add State(s) to Queue__jki_lib_state_machine.vi"("State(s) in Front (\"\")"=w1806, "State(s) in (\"\")"=w1816) -> ("States Out"=w1815:string)  [unwired: 13 in]
          }
          frame "Process: Self Terminate" {
            n799 = Unbundle By Name(w1818) -> ("SelfRef"=w1817:refnum<class "Instrument UI.Lockin.lvclass">)
            n800 = call <vilib>:"SelfTerminate.vi"("error in (no error)"=w1820, "SMO in"=w1817) -> ("error out"=w1819:errorcluster)  [unwired: 8 in, 1 out]
            n801 = call <vilib>:"Add State(s) to Queue__jki_lib_state_machine.vi"("State(s) in (\"\")"=w1823) -> ("States Out"=w1822:string)  [unwired: 14 in]
          }
          frame "---------- Events ----------" {
            # "Template Separator\n(You can make a copy of, or modify, this frame)"
            n802 = call <vilib>:"Add State(s) to Queue__jki_lib_state_machine.vi"("State(s) in (\"\")"=w1828) -> ("States Out"=w1827:string)  [unwired: 14 in]
          }
          frame "Events: Register" {
            # "Base Class Protected Events"
            n803 = Unbundle By Name(w1845) -> ("SelfRef"=w1841:refnum<class "Instrument UI.Lockin.lvclass">, "Lockin"=w1835:refnum<class "Instrument.Lockin.lvclass">)
            n804 = call <vilib>:"GetProtectedEvents.vi"("SMO"=w1841) -> ("error out"=w1842:errorcluster, "SMO Protected Events"=w1834:T66, "SMO out"=w1833:refnum<class "Instrument UI.Lockin.lvclass">)  [unwired: 8 in]
            n805 = call <userlib>:"Instrument.GetPublicEvents.vi"("Instrument"=w1835) -> ("error out"=w1840:errorcluster, "Instrument Public Events"=w1836:T67, "Instrument out"=w1837:refnum<class "Instrument.Lockin.lvclass">)  [unwired: 8 in]
            n806 = call <vilib>:"SMO.UI.GetPublicEvents.vi"("SMO.UI"=w1833) -> ("SMO.UI Public Events"=w1832:T68)  [unwired: 8 in, 2 out]
            n807 = call "Lockin.getDAQPublicEvents.vi"("Instrument.Lockin in"=w1837) -> ("error out"=w1830:errorcluster, "DAQ SMO Public Events"=w1831:T69, "DAQ Public Events"=w1829:T70)  [unwired: 7 in, 1 out]
            n808 = register-events(w1834, w1832, w1836, w1829, w1831) -> (reference out=w1844:refnum<event-registration>, error out=w1839:errorcluster)  [unwired: 2 in]
            n809 = Merge Errors(w1839, w1830, w1840, w1842, w1838) -> (w1843:errorcluster)
            n810 = call <vilib>:"Add State(s) to Queue__jki_lib_state_machine.vi"("State(s) in (\"\")"=w1847) -> ("States Out"=w1846:string)  [unwired: 14 in]
          }
          frame "Events: Unregister" {
            n811 = Unregister For Events(event registration refnum=w1850, error in=w1849) -> (error out=w1848:errorcluster)
            n812 = call <vilib>:"Add State(s) to Queue__jki_lib_state_machine.vi"("State(s) in (\"\")"=w1853) -> ("States Out"=w1852:string)  [unwired: 14 in]
          }
          frame "---------- Action ----------" {
            n813 = Unbundle By Name(w1854) -> ("SelfRef"=w1856:refnum<class "Instrument UI.Lockin.lvclass">)
            n814 = Bundle By Name(cluster=w1854, "SelfRef"=w1856) -> (w1855:T63)
            n815 = call <vilib>:"Add State(s) to Queue__jki_lib_state_machine.vi"("State(s) in (\"\")"=w1860) -> ("States Out"=w1859:string)  [unwired: 14 in]
          }
          frame "Action: ><><>Unhandled Controls<><><" {
            n816 = call <vilib>:"Add State(s) to Queue__jki_lib_state_machine.vi"("State(s) in (\"\")"=w1865) -> ("States Out"=w1864:string)  [unwired: 14 in]
          }
          frame "Action: Notify UI Closed" {
            # "Notify that the UI has been closed"
            n817 = Unbundle By Name(w1868) -> ("SelfRef"=w1869:refnum<class "Instrument UI.Lockin.lvclass">)
            n818 = call <vilib>:"Hide.vi"("error in (no error)"=w1867, "SMO.UI"=w1869) -> ("error out"=w1866:errorcluster)  [unwired: 8 in, 1 out]
            n819 = call <vilib>:"Add State(s) to Queue__jki_lib_state_machine.vi"("State(s) in (\"\")"=w1872) -> ("States Out"=w1871:string)  [unwired: 14 in]
          }
          frame "Action: Flush Queue" {
            n820 = Unbundle By Name(w1876) -> ("SelfRef"=w1878:refnum<class "Instrument UI.Lockin.lvclass">)
            n821 = disable-structure shown="Disabled" {
              disable-tunnel: w1875 -> [w1883 _]
              disable-tunnel: w1874 -> [w1882 w1884]
              disable-tunnel: [w1881 w1884] -> w1873
              frame Disabled {
                n822 = Flush Event Queue(0:w1883, 3:w1882) -> (11:w1881:errorcluster)  [unwired: 4 in, 2 out]
              }
              frame Enabled {
              }
            }
            n823 = Bundle By Name(cluster=w1876, "SelfRef"=w1878) -> (w1877:T63)
            n824 = call <vilib>:"Add State(s) to Queue__jki_lib_state_machine.vi"("State(s) in (\"\")"=w1880) -> ("States Out"=w1879:string)  [unwired: 14 in]
          }
          frame "Action: Command" {
            n825 = Unbundle By Name(w1889) -> ("Lockin"=w1887:refnum<class "Instrument.Lockin.lvclass">, "Message.Command"=w1885:variant, "Message.Data"=w1886:variant)
            n826 = call "Lockin.Local Client.vim"("error in (no error)"=w1891, "Data"=w1886, "Command"=w1885, "Instrument.Lockin in"=w1887) -> ("error out"=w1890:errorcluster, "Instrument.Lockin out"=w1892:refnum<class "Instrument.Lockin.lvclass">)  [unwired: 6 in]
            n827 = Bundle By Name(cluster=w1889, "Lockin"=w1892) -> (w1893:T63)
            n828 = call <vilib>:"Add State(s) to Queue__jki_lib_state_machine.vi"("State(s) in Front (\"\")"="" ("State(s) in Front (\"\")"), "State(s) in (\"\")"=w1896) -> ("States Out"=w1895:string)  [unwired: 13 in]
          }
          frame "Action: State" {
            n829 = Scan From String(input string=w1901, default 1=Set_State-enum."start" ("State")) -> (output 1=w1898:T31)  [unwired: 3 in, 3 out]
            n830 = Bundle By Name(cluster=T38 {"State"=enum."start"} ("setState"), "State"=w1898) -> (w1897:T38)
            n831 = Bundle By Name(cluster=w1903, "Message.Command"=Lockin.Commands--Enum."setState" ("Locking.Commands"), "Message.Data"=w1897) -> (w1904:T63)
            n832 = call <vilib>:"Add State(s) to Queue__jki_lib_state_machine.vi"("State(s) in (\"\")"=w1908) -> ("States Out"=w1907:string)  [unwired: 14 in]
          }
          frame "Action: showUI" {
            n833 = Scan From String(input string=w1912, default 1=T39 FALSE ("showDAQUI")) -> (output 1=w1909:T39)  [unwired: 3 in, 3 out]
            n834 = Bundle By Name(cluster=w1913, "Message.Command"=Lockin.Commands.Local--Enum."showUI" ("Locking.Commands.Local"), "Message.Data"=w1909) -> (w1914:T63)
            n835 = call <vilib>:"Add State(s) to Queue__jki_lib_state_machine.vi"("State(s) in (\"\")"=w1918) -> ("States Out"=w1917:string)  [unwired: 14 in]
          }
          frame "Action: Logging" {
            n836 = Scan From String(input string=w1930, default 1=FALSE ("showDAQUI")) -> (output 1=w1923:bool)  [unwired: 3 in, 3 out]
            n837 = Select(t=Lockin.Commands--Enum."startLogging" ("Locking.Commands"), s=w1923, f=Lockin.Commands--Enum."stopLogging" ("Locking.Commands")) -> (s? t:f=w1924:T29)
            n838 = Bundle By Name(cluster=T40 {"interval"=1} ("setLogging"), "interval"=u32 1000 ("LogMode")) -> (w1927:T40)
            n839 = To Variant(anything=w1927) -> (Variant=w1921:variant)
            n840 = Select(t=w1921, s=w1923, f=variant) -> (s? t:f=w1920:variant)
            n841 = Bundle By Name(cluster=w1931, "Message.Command"=w1924, "Message.Data"=w1920) -> (w1932:T63)
            n842 = call <vilib>:"Add State(s) to Queue__jki_lib_state_machine.vi"("State(s) in (\"\")"=w1936) -> ("States Out"=w1935:string)  [unwired: 14 in]
          }
          frame "Action: Auto DAQ" {
            n843 = Bundle By Name(cluster=w1938, "Message.Command"=Lockin.Commands.Local--Enum."autoConfigureDAQ" ("Locking.Commands.Local")) -> (w1939:T63)
            n844 = call <vilib>:"Add State(s) to Queue__jki_lib_state_machine.vi"("State(s) in (\"\")"=w1943) -> ("States Out"=w1942:string)  [unwired: 14 in]
          }
          frame "Action: DAQ Config" {
            n845 = Unbundle By Name(w1946) -> ("UI Config.DAQ.Configuration"=w1944:T11)
            n846 = Bundle By Name(cluster=w1946, "Message.Command"=Lockin.Commands--Enum."setDAQ" ("Locking.Commands"), "Message.Data"=w1944) -> (w1947:T63)
            n847 = call <vilib>:"Add State(s) to Queue__jki_lib_state_machine.vi"("State(s) in (\"\")"=w1951) -> ("States Out"=w1950:string)  [unwired: 14 in]
          }
          frame "Action: AI Channels" {
            n848 = Unbundle By Name(w1954) -> ("UI Config.Channels.Cfg_AI"=w1953:T2)
            n849 = Bundle By Name(cluster=w1954, "Message.Command"=Lockin.Commands.Local--Enum."setAI" ("Locking.Commands.Local"), "Message.Data"=w1953) -> (w1955:T63)
            n850 = call <vilib>:"Add State(s) to Queue__jki_lib_state_machine.vi"("State(s) in (\"\")"=w1959) -> ("States Out"=w1958:string)  [unwired: 14 in]
          }
          frame "Action: AO Channels" {
            n851 = Unbundle By Name(w1962) -> ("UI Config.Channels.Cfg_AO"=w1960:T4)
            n852 = Bundle By Name(cluster=w1962, "Message.Command"=Lockin.Commands--Enum."setAO" ("Locking.Commands"), "Message.Data"=w1960) -> (w1963:T63)
            n853 = call <vilib>:"Add State(s) to Queue__jki_lib_state_machine.vi"("State(s) in (\"\")"=w1967) -> ("States Out"=w1966:string)  [unwired: 14 in]
          }
          frame "Action: AO Zero Amplitude" {
            n854 = Unbundle By Name(w1968) -> ("UI Config.Channels.Cfg_AO"=w1971:T4)
            n855 = for {
              tunnel: w1971 -> [w1980] mode=indexing
              tunnel: [w1978] -> w1970 mode=indexing
              n856 = Bundle By Name(cluster=w1980, "Amplitude"=0.0 ("element")) -> (w1978:T5)
            }
            n857 = Bundle By Name(cluster=w1968, "Message.Command"=Lockin.Commands--Enum."setAO" ("Enum"), "Message.Data"=w1970) -> (w1969:T63)
            n858 = call <vilib>:"Add State(s) to Queue__jki_lib_state_machine.vi"("State(s) in Front (\"\")"="", "State(s) in (\"\")"=w1977) -> ("States Out"=w1976:string)  [unwired: 13 in]
          }
          frame "Action: REF Channels" {
            n859 = Unbundle By Name(w1983) -> ("UI Config.Channels.Cfg_REF"=w1981:T7)
            n860 = Bundle By Name(cluster=w1983, "Message.Command"=Lockin.Commands--Enum."setREF" ("Locking.Commands"), "Message.Data"=w1981) -> (w1984:T63)
            n861 = call <vilib>:"Add State(s) to Queue__jki_lib_state_machine.vi"("State(s) in (\"\")"=w1988) -> ("States Out"=w1987:string)  [unwired: 14 in]
          }
          frame "Action: Sweep" {
            n862 = Unbundle By Name(w1991) -> ("UI Config.Sweep"=w1989:T54)
            n863 = Bundle By Name(cluster=w1991, "Message.Command"=Lockin.Commands--Enum."setSweep" ("Locking.Commands"), "Message.Data"=w1989) -> (w1992:T63)
            n864 = call <vilib>:"Add State(s) to Queue__jki_lib_state_machine.vi"("State(s) in (\"\")"=w1996) -> ("States Out"=w1995:string)  [unwired: 14 in]
          }
          frame "Action: Sampling" {
            w1998 = Lockin.Commands--Enum."setSampling"  # Lockin.Commands
            n865 = Unbundle By Name(w1999) -> ("UI Config.DAQ.cfg.Sampling.Sampling"=w1997:T48)
            n866 = Bundle By Name(cluster=w1999, "Message.Command"=w1998, "Message.Data"=w1997) -> (w2000:T63)
            n867 = call <vilib>:"Add State(s) to Queue__jki_lib_state_machine.vi"("State(s) in (\"\")"=w2004) -> ("States Out"=w2003:string)  [unwired: 14 in]
          }
          frame "Action: Sampling Mode" {
            n868 = Unbundle By Name(w2009) -> ("UI Config.DAQ.cfg.Sampling.sample mode"=w2006:i32)
            n869 = Bundle By Name(cluster=T41 {"SampleMode"=10123} ("setSampleMode"), "SampleMode"=w2006) -> (w2005:T41)
            n870 = Bundle By Name(cluster=w2009, "Message.Command"=Lockin.Commands.Local--Enum."setSamplingMode" ("Enum"), "Message.Data"=w2005) -> (w2010:T63)
            n871 = call <vilib>:"Add State(s) to Queue__jki_lib_state_machine.vi"("State(s) in (\"\")"=w2014) -> ("States Out"=w2013:string)  [unwired: 14 in]
          }
          frame "Action: Sampling Fs Mode" {
            n872 = Unbundle By Name(w2019) -> ("UI Config.DAQ.cfg.Sampling.Fs Mode"=w2016:T16)
            n873 = Bundle By Name(cluster=T43 {"FsMode"=enum."Manual"} ("setSampleFsMode"), "FsMode"=w2016) -> (w2015:T43)
            n874 = Bundle By Name(cluster=w2019, "Message.Command"=Lockin.Commands--Enum."setSamplingFsMode" ("Commands"), "Message.Data"=w2015) -> (w2020:T63)
            n875 = call <vilib>:"Add State(s) to Queue__jki_lib_state_machine.vi"("State(s) in (\"\")"=w2024) -> ("States Out"=w2023:string)  [unwired: 14 in]
          }
          frame "Action: Sampling Fs Multiplier" {
            n876 = Unbundle By Name(w2027) -> ("UI Config.DAQ.cfg.Sampling.Fs Multiplier"=w2026:dbl)
            n877 = Bundle By Name(cluster=w2027, "Message.Command"=Lockin.Commands.Local--Enum."setSamplingFsMultiplier" ("Locking.Commands.Local"), "Message.Data"=w2026) -> (w2028:T63)
            n878 = call <vilib>:"Add State(s) to Queue__jki_lib_state_machine.vi"("State(s) in (\"\")"=w2032) -> ("States Out"=w2031:string)  [unwired: 14 in]
          }
          frame "Action: Sampling Fs Output" {
            n879 = Unbundle By Name(w2035) -> ("UI Config.DAQ.cfg.Sampling.Fs.Output"=w2034:dbl)
            n880 = Bundle By Name(cluster=w2035, "Message.Command"=Lockin.Commands.Local--Enum."setSamplingFsOutput" ("Locking.Commands.Local"), "Message.Data"=w2034) -> (w2036:T63)
            n881 = call <vilib>:"Add State(s) to Queue__jki_lib_state_machine.vi"("State(s) in (\"\")"=w2040) -> ("States Out"=w2039:string)  [unwired: 14 in]
          }
          frame "Action: Sampling Refresh Rate" {
            n882 = Unbundle By Name(w2043) -> ("UI Config.DAQ.cfg.Sampling.Refresh Rate (Hz)"=w2042:dbl)
            n883 = Bundle By Name(cluster=w2043, "Message.Command"=Lockin.Commands.Local--Enum."setSamplingRefreshRate" ("Locking.Commands.Local"), "Message.Data"=w2042) -> (w2044:T63)
            n884 = call <vilib>:"Add State(s) to Queue__jki_lib_state_machine.vi"("State(s) in (\"\")"=w2048) -> ("States Out"=w2047:string)  [unwired: 14 in]
          }
          frame "Action: Sampling Decimation Pre DSP" {
            n885 = Unbundle By Name(w2051) -> ("UI Config.DAQ.cfg.Sampling.Decimation.PreDSP"=w2050:i32)
            n886 = Bundle By Name(cluster=w2051, "Message.Command"=Lockin.Commands.Local--Enum."setSamplingDecimationPreDSP" ("Locking.Commands.Local"), "Message.Data"=w2050) -> (w2052:T63)
            n887 = call <vilib>:"Add State(s) to Queue__jki_lib_state_machine.vi"("State(s) in (\"\")"=w2056) -> ("States Out"=w2055:string)  [unwired: 14 in]
          }
          frame "Action: Sampling Decimation Post DSP" {
            n888 = Unbundle By Name(w2059) -> ("UI Config.DAQ.cfg.Sampling.Decimation.PostDSP"=w2058:i32)
            n889 = Bundle By Name(cluster=w2059, "Message.Command"=Lockin.Commands.Local--Enum."setSamplingDecimationPostDSP" ("Locking.Commands.Local"), "Message.Data"=w2058) -> (w2060:T63)
            n890 = call <vilib>:"Add State(s) to Queue__jki_lib_state_machine.vi"("State(s) in (\"\")"=w2064) -> ("States Out"=w2063:string)  [unwired: 14 in]
          }
          frame "Action: AI Simulate Mode" {
            n891 = Unbundle By Name(w2067) -> ("UI Config.DAQ.Simulation mode"=w2066:T17)
            n892 = Bundle By Name(cluster=w2067, "Message.Command"=Lockin.Commands.Local--Enum."setSimulationMode" ("Locking.Commands.Local"), "Message.Data"=w2066) -> (w2068:T63)
            n893 = call <vilib>:"Add State(s) to Queue__jki_lib_state_machine.vi"("State(s) in (\"\")"=w2072) -> ("States Out"=w2071:string)  [unwired: 14 in]
          }
          frame "Action: Limit Amplitude" {
            n894 = Unbundle By Name(w2075) -> ("UI Config.Limit Amplitude"=w2074:T51)
            n895 = Bundle By Name(cluster=w2075, "Message.Command"=Lockin.Commands.Local--Enum."setLimitAmplitude" ("Locking.Commands.Local"), "Message.Data"=w2074) -> (w2076:T63)
            n896 = call <vilib>:"Add State(s) to Queue__jki_lib_state_machine.vi"("State(s) in (\"\")"=w2080) -> ("States Out"=w2079:string)  [unwired: 14 in]
          }
          frame "Action: Limit DC" {
            n897 = Unbundle By Name(w2083) -> ("UI Config.Limit DC"=w2082:T52)
            n898 = Bundle By Name(cluster=w2083, "Message.Command"=Lockin.Commands.Local--Enum."setLimitDC" ("Locking.Commands.Local"), "Message.Data"=w2082) -> (w2084:T63)
            n899 = call <vilib>:"Add State(s) to Queue__jki_lib_state_machine.vi"("State(s) in (\"\")"=w2088) -> ("States Out"=w2087:string)  [unwired: 14 in]
          }
          frame "Action: Link Frequencies" {
            n900 = Unbundle By Name(w2091) -> ("UI Config.Link Frequencies"=w2090:T53)
            n901 = Bundle By Name(cluster=w2091, "Message.Command"=Lockin.Commands.Local--Enum."setLinkFrequencies" ("Locking.Commands.Local"), "Message.Data"=w2090) -> (w2092:T63)
            n902 = call <vilib>:"Add State(s) to Queue__jki_lib_state_machine.vi"("State(s) in (\"\")"=w2096) -> ("States Out"=w2095:string)  [unwired: 14 in]
          }
          frame "Action: PreFilter" {
            n903 = Unbundle By Name(w2099) -> ("UI Config.PreFilter"=w2098:T49)
            n904 = Bundle By Name(cluster=w2099, "Message.Command"=Lockin.Commands.Local--Enum."setPreFilter" ("Locking.Commands.Local"), "Message.Data"=w2098) -> (w2100:T63)
            n905 = call <vilib>:"Add State(s) to Queue__jki_lib_state_machine.vi"("State(s) in (\"\")"=w2104) -> ("States Out"=w2103:string)  [unwired: 14 in]
          }
          frame "Action: Input Gain" {
            n906 = Unbundle By Name(w2108) -> ("UI Config.Amplifers.Gain_AI"=w2106:T9)
            n907 = for {
              tunnel: w2106 -> [w2115] mode=indexing
              tunnel: [w2114] -> w2105 mode=indexing
              n908 = Unbundle By Name(w2115) -> ("Gain"=w2114:dbl)
            }
            n909 = Bundle By Name(cluster=w2108, "Message.Command"=Lockin.Commands--Enum."setInputGain" ("Locking.Commands"), "Message.Data"=w2105) -> (w2109:T63)
            n910 = call <vilib>:"Add State(s) to Queue__jki_lib_state_machine.vi"("State(s) in (\"\")"=w2113) -> ("States Out"=w2112:string)  [unwired: 14 in]
          }
          frame "Action: Output Gain" {
            n911 = Unbundle By Name(w2119) -> ("UI Config.Amplifers.Gain_AO"=w2117:T9)
            n912 = for {
              tunnel: w2117 -> [w2126] mode=indexing
              tunnel: [w2125] -> w2116 mode=indexing
              n913 = Unbundle By Name(w2126) -> ("Gain"=w2125:dbl)
            }
            n914 = Bundle By Name(cluster=w2119, "Message.Command"=Lockin.Commands--Enum."setOutputGain" ("Locking.Commands"), "Message.Data"=w2116) -> (w2120:T63)
            n915 = call <vilib>:"Add State(s) to Queue__jki_lib_state_machine.vi"("State(s) in (\"\")"=w2124) -> ("States Out"=w2123:string)  [unwired: 14 in]
          }
          frame "Action: Offset" {
            n916 = Unbundle By Name(w2128) -> ("UI Config.Amplifers.Offset_AI"=w2129:T9)
            n917 = for {
              tunnel: w2129 -> [w2137] mode=indexing
              tunnel: [w2136] -> w2127 mode=indexing
              n918 = Unbundle By Name(w2137) -> ("Gain"=w2136:dbl)
            }
            n919 = Bundle By Name(cluster=w2128, "Message.Command"=Lockin.Commands.Local--Enum."setOffset" ("Locking.Commands.Local"), "Message.Data"=w2127) -> (w2131:T63)
            n920 = call <vilib>:"Add State(s) to Queue__jki_lib_state_machine.vi"("State(s) in (\"\")"=w2135) -> ("States Out"=w2134:string)  [unwired: 14 in]
          }
          frame "Action: Offset Mode" {
            n921 = Scan From String(input string=w2141, default 1=Offset_Mode--Enum."Measure" ("Offset Mode")) -> (output 1=w2140:T33)  [unwired: 3 in, 3 out]
            n922 = Build Array(w2140) -> (w2139:T33[])
            n923 = Bundle By Name(cluster=w2143, "Message.Command"=Lockin.Commands.Local--Enum."setOffsetMode" ("Locking.Commands.Local"), "Message.Data"=w2139) -> (w2144:T63)
            n924 = call <vilib>:"Add State(s) to Queue__jki_lib_state_machine.vi"("State(s) in (\"\")"=w2148) -> ("States Out"=w2147:string)  [unwired: 14 in]
          }
          frame "Action: Calibrate" {
            n925 = Scan From String(input string=w2151, default 1=PrivateEvents--DAQ.setCalibration."Check" ("setCalibration")) -> (output 1=w2150:T34)  [unwired: 3 in, 3 out]
            n926 = Bundle By Name(cluster=w2153, "Message.Command"=Lockin.Commands.Local--Enum."setCalibration" ("Locking.Commands.Local"), "Message.Data"=w2150) -> (w2154:T63)
            n927 = call <vilib>:"Add State(s) to Queue__jki_lib_state_machine.vi"("State(s) in (\"\")"=w2158) -> ("States Out"=w2157:string)  [unwired: 14 in]
          }
          frame "Action: Zero Phase" {
            n928 = Bundle By Name(cluster=w2160, "Message.Command"=Lockin.Commands.Local--Enum."zeroPhase" ("Locking.Commands.Local")) -> (w2161:T63)
            n929 = call <vilib>:"Add State(s) to Queue__jki_lib_state_machine.vi"("State(s) in (\"\")"=w2165) -> ("States Out"=w2164:string)  [unwired: 14 in]
          }
          frame "Action: Power Spectrum" {
            n930 = Unbundle By Name(w2181) -> ("getAll.Waveforms.AI_wfm"=w2180:waveform(dbl)[])
            n931 = Bundle By Name(cluster=T44 {"averaging mode"=enum."No averaging", "weighting mode"=enum."Exponential", "number of averages"=10} ("averaging parameters"), "averaging mode"="averaging mode", "weighting mode"="weighting mode", "number of averages"="# averages") -> (w2168:T44)
            n932 = call-poly <vilib>:"FFT Power Spectrum and PSD.vi"("export mode"="export mode", "averaging parameters"=w2168, "restart averaging (F)"="restart", "error in (no error)"=w2178, "dB On (F)"=TRUE, "window"="window", "time signals"=w2180) -> ("error out"=w2179:errorcluster, "averages completed"=→"averages":dbl, "averaging done"=→"done?":bool, "Power Spectrum / PSD"=→"PS WFGraph":cluster{"f0":dbl, "df":dbl, "magnitude":dbl[]}[])  [unwired: 1 in]
            n933 = flat-sequence {
              frame #0 {
                # "Power Spectrum"
                n934 = disable-structure shown="Disabled" {
                  frame Disabled {
                    n935 = call "PS Chart.vi"() -> ("Chart"=→"PS Chart":dbl[][])  [unwired: 10 in, 1 out]
                  }
                  frame Enabled {
                  }
                }
              }
            }
            n936 = call <vilib>:"Add State(s) to Queue__jki_lib_state_machine.vi"("State(s) in (\"\")"=w2184) -> ("States Out"=w2183:string)  [unwired: 14 in]
          }
          frame "Action: Route" {
            n937 = Unbundle By Name(w2186) -> ("SelfRef"=w2188:refnum<class "Instrument UI.Lockin.lvclass">)
            n938 = flat-sequence {
              frame #0 {
                # "Route In to Out"
                n939 = disable-structure shown="Disabled" {
                  frame Disabled {
                    n940 = call "Parse Results (single).vi"("Type"="Type", "Reference Channel"="Reference Channel", "AI Channel"="AI Channel") -> ("Data"=w2193:dbl)  [unwired: 5 in, 3 out]
                    "Output (V)" <- w2193
                    n941 = call-dynamic "setAO_DC.vi"("DC (V)"=w2193, "AO Channel"="Output Channel") -> ()  [unwired: 8 in, 2 out]
                  }
                  frame Enabled {
                  }
                }
              }
            }
            n942 = Bundle By Name(cluster=w2186, "SelfRef"=w2188) -> (w2187:T63)
            n943 = call <vilib>:"Add State(s) to Queue__jki_lib_state_machine.vi"("State(s) in (\"\")"=w2192) -> ("States Out"=w2191:string)  [unwired: 14 in]
          }
          frame "Action: Aux" {
            n944 = Unbundle By Name(w2198) -> ("SelfRef"=w2200:refnum<class "Instrument UI.Lockin.lvclass">)
            n945 = flat-sequence {
              frame #0 {
                # "AUX Out"
                n946 = disable-structure shown="Disabled" {
                  frame Disabled {
                  }
                  frame Enabled {
                  }
                }
              }
            }
            n947 = Bundle By Name(cluster=w2198, "SelfRef"=w2200) -> (w2199:T63)
            n948 = call <vilib>:"Add State(s) to Queue__jki_lib_state_machine.vi"("State(s) in (\"\")"=w2204) -> ("States Out"=w2203:string)  [unwired: 14 in]
          }
        }
      }
    }
    frame Error {
    }
  }
  n949 = call-parent "Process.vi"("error in"=w7, "Instrument UI in"=w6) -> ("error out"=w4:errorcluster, "Instrument UI out"=→"Lockin.UI out":refnum<class "Instrument UI.Lockin.lvclass">)  [unwired: 8 in]
  n950 = Format Into String(w1) -> ()  [unwired: 3 in, 2 out]
  n951 = Format Into String(w2) -> ()  [unwired: 3 in, 2 out]
  n952 = Merge Errors(w4, w3) -> (→"error out":errorcluster)
